vi "数据编码.vi"(0 "table输入":string(combo), 1 "仪器参数上传时间":enum16{"精确到小时", "原始时间"}(ring), 5 "错误常量 2":errorcluster caption="错误输入", 7 "仪器参数":string[](array[string]), 9 "QN":string, 11 "参数":string, 13 "MN":string, 14 "PW":string) -> (4 "错误常量":errorcluster caption="错误输出", 15 "通讯包字符串":string)   [LabVIEW 2016, in "数据传输系统-02.lvlib"]
panel:
  out "核查数据发送次数":i32
  out "小时数据发送次数":i32
  out "长度":i32
  in  "数据块":T1
  out "通讯包":T2={"包头（2）"="##", "数据段长度（4）"="", "数据段"="", "CRC校验"="", "包尾"=""}
  # "范例代码：\n\n##0101QN=20160801085857223;ST=32;CN=1062;PW=100000;MN=010000A8900016F000169DC0;Flag=5\n;CP=&&RtdInterval=30&&1C80\\r\\n"
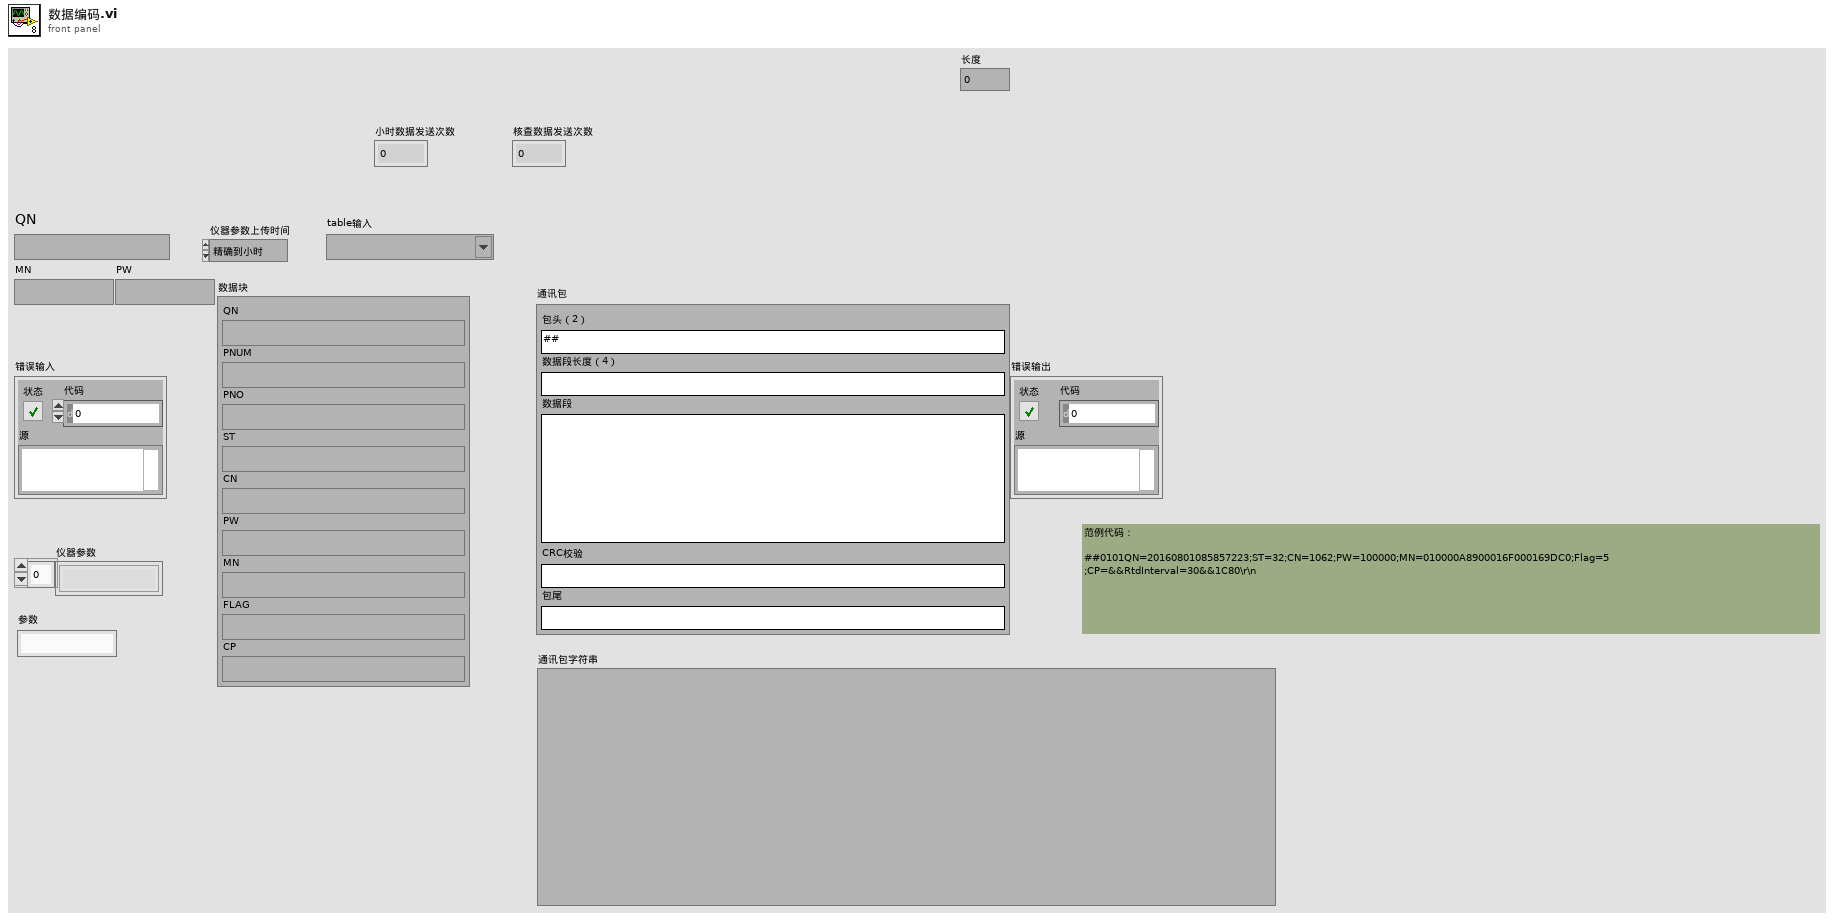
[diagram p1: front panel]
types:
  T1 = cluster{"QN":string, "ST":string, "CN":string, "PW":string, "MN":string, "FLAG":string, "PNUM":string, "PNO":string, "CP":string}
  T2 = cluster{"包头（2）":string, "数据段长度（4）":string, "数据段":string, "CRC校验":string, "包尾":string}
  T3 = cluster{"PH":string[][], "CODCr":string[][], "氨氮":string[][], "CODMn":string[][], "总氮":string[][], "总磷":string[][], "电导率":string[][], "水温":string[][], "COD":string[][], "DO":string[][], "浊度":string[][], "叶绿素":string[][], "藻密度":string[][], "铜":string[][], "盐度":string[][], "水位":string[][], "流速":string[][], "方向":string[][], "瞬时流量":string[][], "累积流量":string[][], "正累积流量":string[][], "负累积流量":string[][], "亚硝酸盐":string[][], "硫化物":string[][], "ORP":string[][], "铅":string[][], "镉":string[][], "锌":string[][], "镍":string[][], "锰":string[][], "汞":string[][], "气温":string[][], "气压":string[][], "风速":string[][], "风向":string[][], "空气温度":string[][], "相对湿度":string[][], "分钟雨量":string[][], "小时雨量":string[][], "日雨量":string[][], "累积雨量":string[][], "盐度":string[][], "磷酸盐":string[][], "硝氮":string[][], "氟化物":string[][], "挥发酚":string[][], "氯化物":string[][], "蓝绿藻":string[][], "余氯":string[][], "综合生物毒性":string[][], "水深":string[][]}
  T4 = enum16{"小时数据", "实时数据", "平行样测试", "集成干预测试", "加标回收测试", "核查数据", "空白零点跨度数据", "提取小时数据", "提取实时数据"}
  T5 = enum16{"小时数据", "实时数据", "平行样测试", "集成干预测试", "加标回收测试", "核查数据", "空白零点跨度数据", "提取小时数据", "提取实时数据", "操作日志"}
  T6 = enum16{"小时数据", "实时数据", "平行样测试", "集成干预测试", "加标回收测试", "核查数据", "空白零点跨度数据", "提取小时数据", "提取实时数据", "操作日志", "仪器参数", "3090仪器参数", "提取仪器参数", "报警信息"}
  T7 = cluster{"CODMn固件信息":string, "氨氮固件信息":string, "总磷固件信息":string, "总氮固件信息":string, "CODCr固件信息":string}
  T8 = typedef "数据传输系统-02.lvlib/应用环境.ctl" = enum16{"STD", "GB212", "婉仪平台"}
  T9 = cluster{"CODMn":dbl, "CODCr":dbl, "DO":dbl, "铜":dbl, "PH":dbl, "氨氮":dbl, "比电导率":dbl, "水温":dbl, "COD":dbl, "浊度":dbl, "总氮":dbl, "总磷":dbl, "叶绿素a":dbl, "藻密度":dbl, "水位":dbl, "流速":dbl, "方向":dbl, "瞬时流量":dbl, "累积流量":dbl, "正累积流量":dbl, "负累积流量":dbl, "亚硝酸盐":dbl, "硫化物":dbl, "ORP":dbl, "铅":dbl, "镉":dbl, "锌":dbl, "镍":dbl, "锰":dbl, "汞":dbl, "气温":dbl, "气压":dbl, "风速":dbl, "风向":dbl, "空气温度":dbl, "相对湿度":dbl, "分钟雨量":dbl, "小时雨量":dbl, "日雨量":dbl, "累积雨量":dbl, "盐度":dbl, "磷酸盐":dbl, "硝氮":dbl, "氟化物":dbl, "挥发酚":dbl, "氯化物":dbl, "蓝绿藻":dbl, "余氯":dbl, "综合生物毒性":dbl, "艏向":dbl, "横摇":dbl, "纵摇":dbl, "分层标志":dbl, "层状态1":dbl, "层状态2":dbl, "水平平均流速":dbl, "流向":dbl, "北向流速分量":dbl, "东向流速分量":dbl, "垂直流速分量":dbl, "最大波高":dbl, "最大波周期":dbl, "1/10波高":dbl, "1/10波周期":dbl, "有效波高":dbl, "有效波周期":dbl, "平均波高":dbl, "平均波周期":dbl, "波向":dbl, "波个数":dbl, "水深":dbl, "X轴流速":dbl, "Y轴流速":dbl, "信号强度":dbl, "电压":dbl, "悬浮物":dbl}
  T10 = cluster{"CODMn":string, "CODCr":string, "DO":string, "铜":string, "PH":string, "氨氮":string, "比电导率":string, "水温":string, "COD":string, "浊度":string, "总氮":string, "总磷":string, "叶绿素a":string, "藻密度":string, "水位":string, "流速":string, "方向":string, "瞬时流量":string, "累积流量":string, "正累积流量":string, "负累积流量":string, "亚硝酸盐":string, "硫化物":string, "ORP":string, "铅":string, "镉":string, "锌":string, "镍":string, "锰":string, "汞":string, "气温":string, "气压":string, "风速":string, "风向":string, "空气温度":string, "相对湿度":string, "分钟雨量":string, "小时雨量":string, "日雨量":string, "累积雨量":string, "盐度":string, "磷酸盐":string, "硝氮":string, "氟化物":string, "挥发酚":string, "氯化物":string, "蓝绿藻":string, "余氯":string, "综合生物毒性":string, "艏向":string, "横摇":string, "纵摇":string, "分层标志":string, "层状态1":string, "层状态2":string, "水平平均流速":string, "流向":string, "北向流速分量":string, "东向流速分量":string, "垂直流速分量":string, "最大波高":string, "最大波周期":string, "1/10波高":string, "1/10波周期":string, "有效波高":string, "有效波周期":string, "平均波高":string, "平均波周期":string, "波向":string, "波个数":string, "水深":string, "X轴流速":string, "Y轴流速":string, "信号强度":string, "电压":string, "悬浮物":string}
  T11 = typedef "LVDateTimeRec.ctl" = cluster{"秒数的小数部分":dbl, "秒":i32, "分":i32, "时":i32, "日":i32, "月":i32, "年":i32, "天数（周）":i32, "天数（年）":i32, "DST":i32}
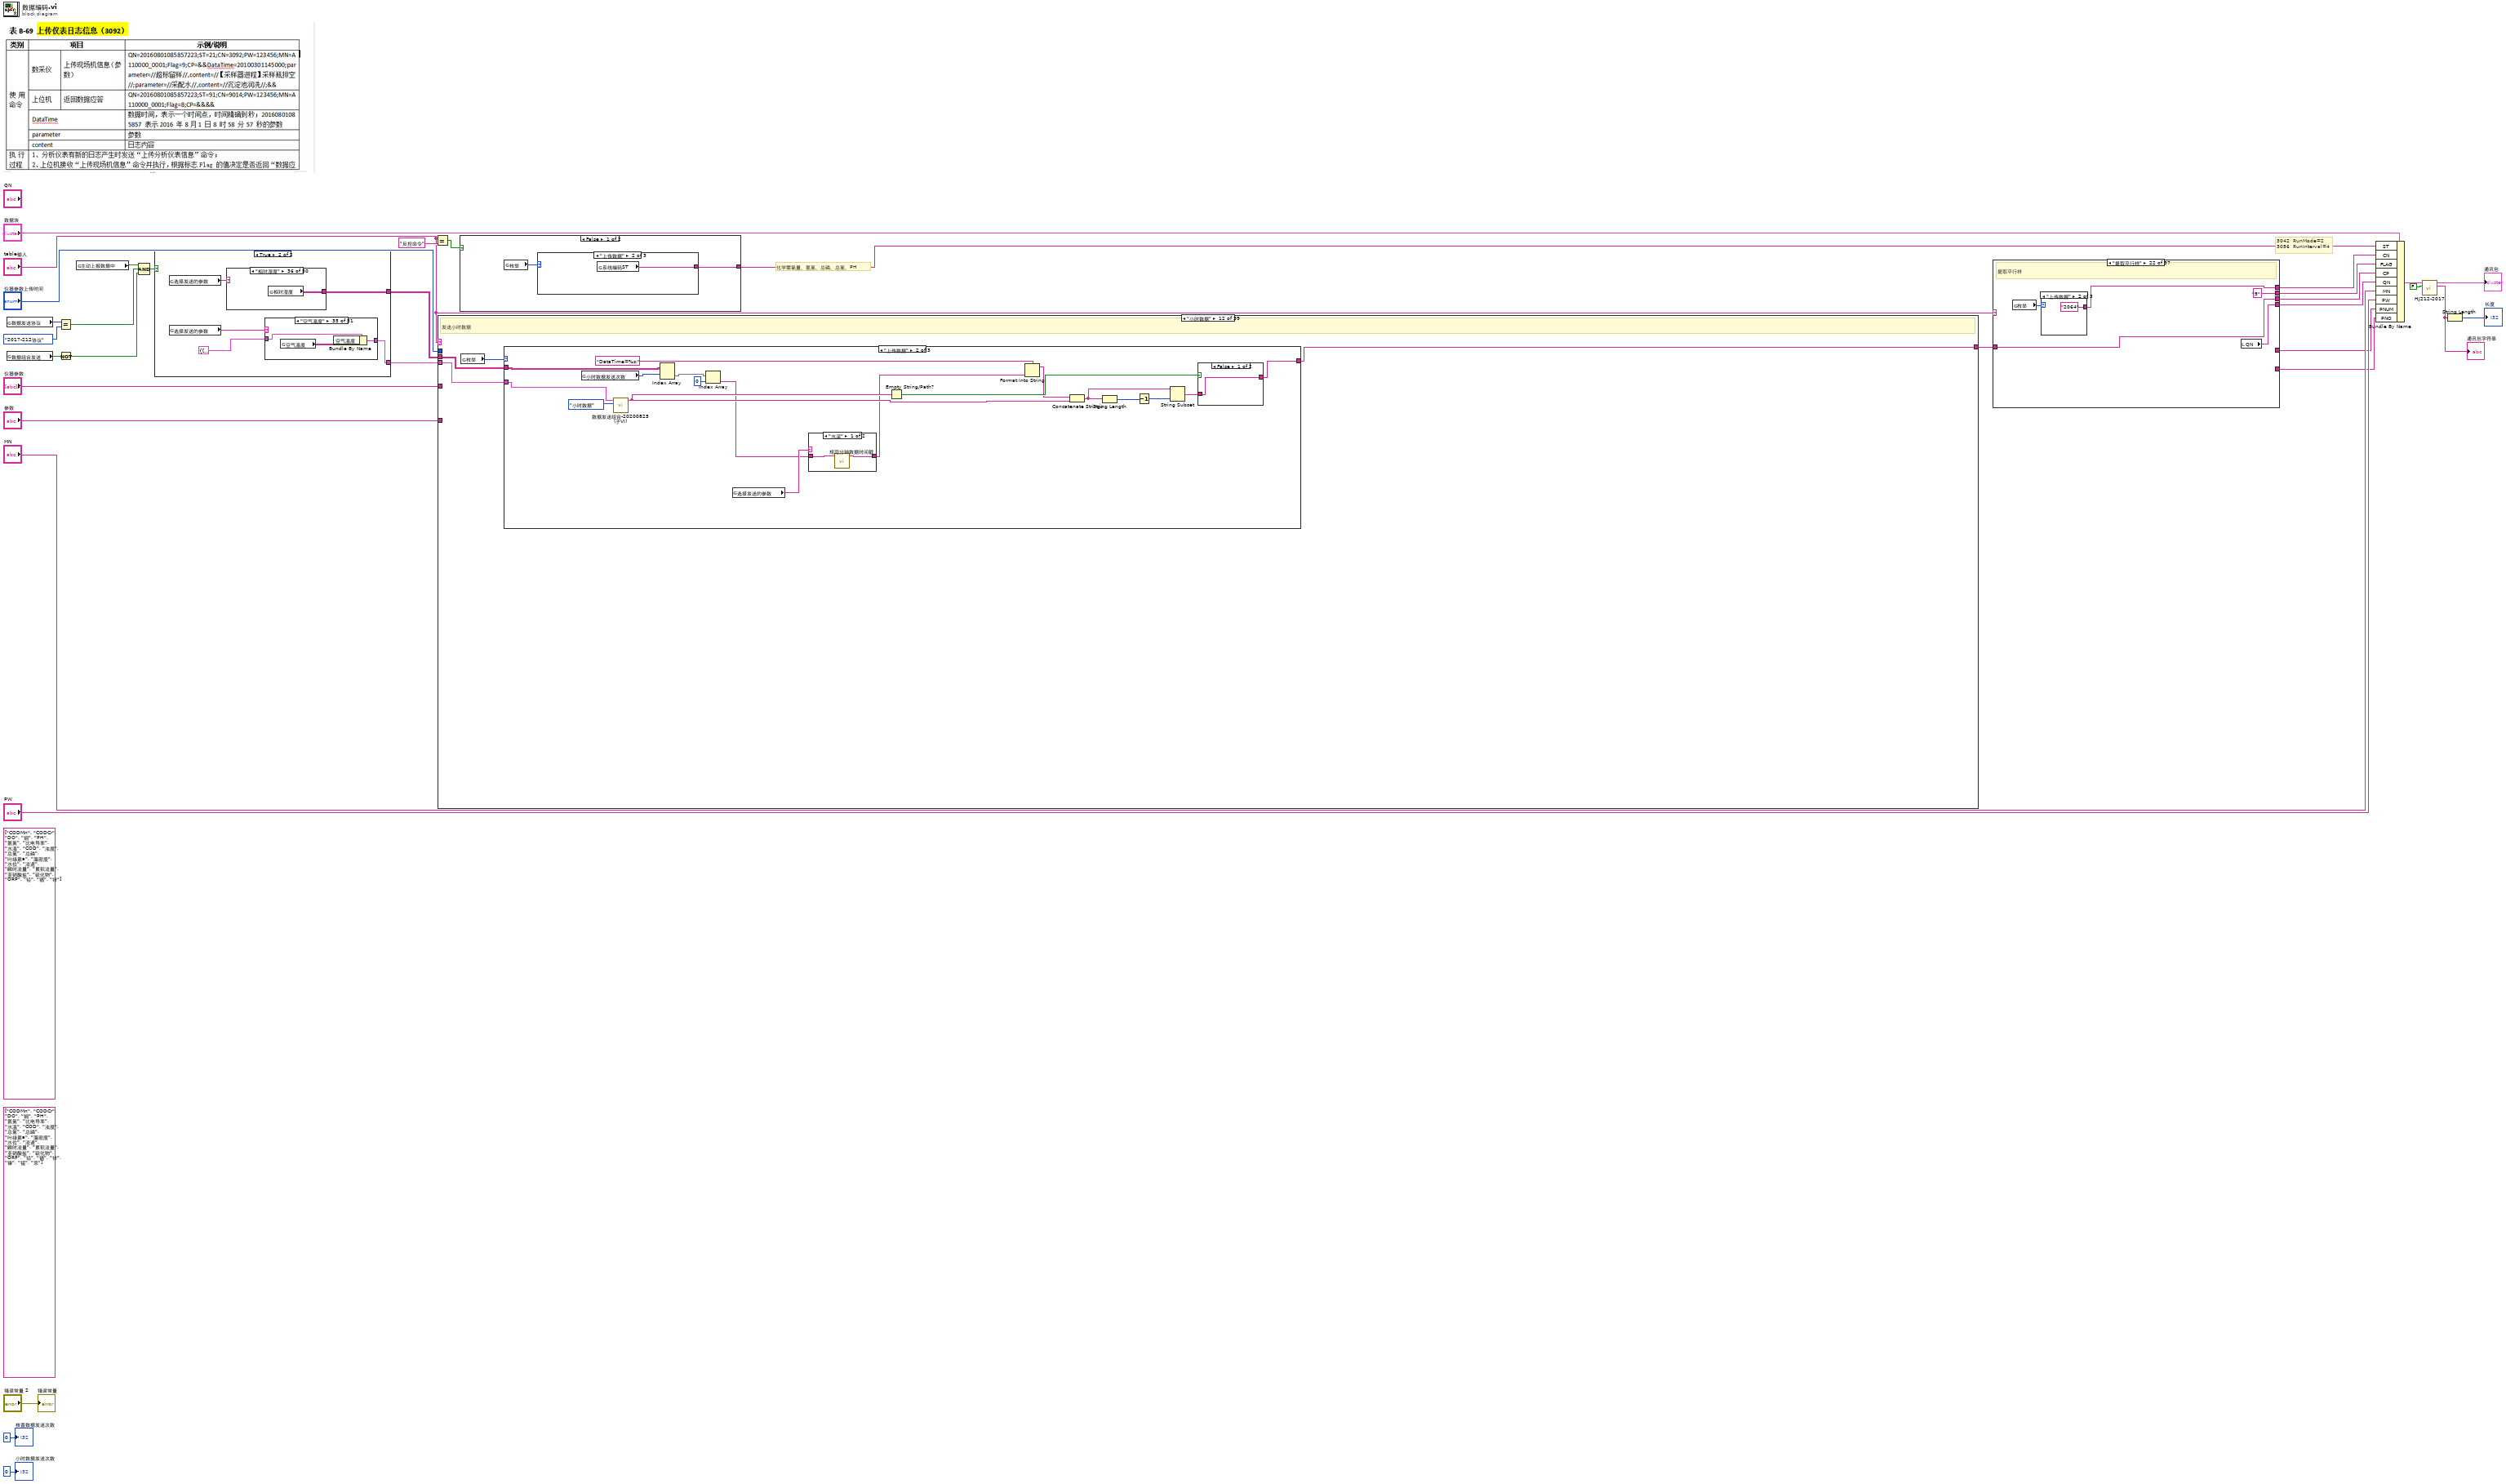
[diagram p0: block diagram]
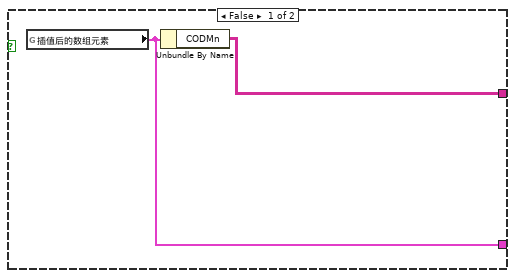
[diagram p2: hidden frame]
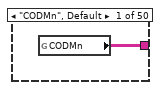
[diagram p3: hidden frame]
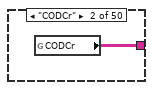
[diagram p4: hidden frame]
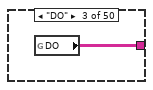
[diagram p5: hidden frame]
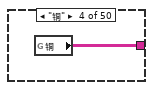
[diagram p6: hidden frame]
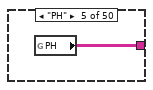
[diagram p7: hidden frame]
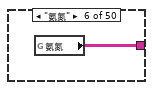
[diagram p8: hidden frame]
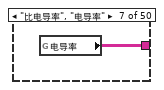
[diagram p9: hidden frame]
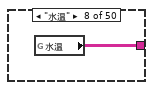
[diagram p10: hidden frame]
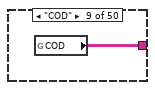
[diagram p11: hidden frame]
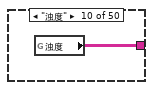
[diagram p12: hidden frame]
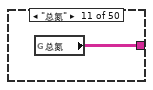
[diagram p13: hidden frame]
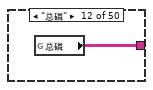
[diagram p14: hidden frame]
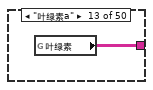
[diagram p15: hidden frame]
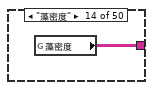
[diagram p16: hidden frame]
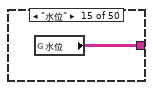
[diagram p17: hidden frame]
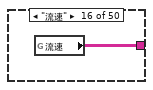
[diagram p18: hidden frame]
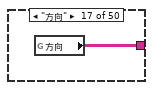
[diagram p19: hidden frame]
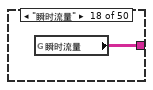
[diagram p20: hidden frame]
diagram:
  (unwired) string[] ["CODMn", "CODCr", "DO", "铜", "PH", "氨氮", "比电导率", "水温", "COD", "浊度", "总氮", "总磷", "叶绿素a", "藻密度", "水位", "流速", "瞬时流量", "累积流量", "亚硝酸盐", "硫化物", "ORP", "铅", "镉", "锌"] ("数组")
  (unwired) string[] ["CODMn", "CODCr", "DO", "铜", "PH", "氨氮", "比电导率", "水温", "COD", "浊度", "总氮", "总磷", "叶绿素a", "藻密度", "水位", "流速", "瞬时流量", "累积流量", "亚硝酸盐", "硫化物", "ORP", "铅", "镉", "锌", "镍", "锰", "汞"] ("数组")
  # "化学需氧量、氨氮、总磷、总氮、PH"
  # "3042  RunMode=2\n3056  RunInterval=4"
  n1 = global read "断电保存全局.vi" "数据发送协议"() -> (w13:enum16{"2005-212协议", "2017-212协议"})
  n2 = global read "断电保存全局.vi" "数据组合发送"() -> (w15:bool)
  n3 = Equal?(x=w13, y=enum16{"2005-212协议", "2017-212协议"}."2017-212协议" ("数据发送版本")) -> (x = y?=w16:bool)
  n4 = Not(x=w15) -> (.not. x?=w14:bool)
  n5 = global read "全局 数据发送重叠.vi" "主动上报数据中"() -> (w19:bool)
  n6 = Compound Arithmetic op=AND ("复合运算")(w19, w16, w14) -> (w17:bool)
  n7 = case shown="True" w17 {
    tunnel: [w36 w40] -> w11
    tunnel: [w35 w38] -> w10
    frame False {
      n8 = global read "插值后的新数组.vi" "插值后的数组元素"() -> (w36:T3)
      n9 = Unbundle By Name(w36) -> ("CODMn"=w35:string[][])
    }
    frame True {
      n10 = global read "全局 水样时间.vi" "选择发送的参数"() -> (w39:string)
      n11 = global read "全局 水样时间.vi" "选择发送的参数"() -> (w41:string)
      n12 = case shown="\"相对湿度\"" w39 {
        tunnel: [w42 w43 w44 w45 w46 w47 w48 w49 w50 w51 w52 w53 w54 w55 w56 w57 w58 w59 w60 w61 w62 w63 w64 w65 w66 w67 w68 w69 w70 w71 w72 w73 w74 w75 w76 w77 w78 w79 w80 w81 w82 w83 w84 w85 w86 w87 w88 w89 w90 w91] -> w38
        frame "CODMn", Default {
          n13 = global read "全局 所有参数.vi" "CODMn"() -> (w42:string[][])
        }
        frame "CODCr" {
          n14 = global read "全局 所有参数.vi" "CODCr"() -> (w43:string[][])
        }
        frame "DO" {
          n15 = global read "全局 所有参数.vi" "DO"() -> (w44:string[][])
        }
        frame "铜" {
          n16 = global read "全局 所有参数.vi" "铜"() -> (w45:string[][])
        }
        frame "PH" {
          n17 = global read "全局 所有参数.vi" "PH"() -> (w46:string[][])
        }
        frame "氨氮" {
          n18 = global read "全局 所有参数.vi" "氨氮"() -> (w47:string[][])
        }
        frame "比电导率", "电导率" {
          n19 = global read "全局 所有参数.vi" "电导率"() -> (w48:string[][])
        }
        frame "水温" {
          n20 = global read "全局 所有参数.vi" "水温"() -> (w49:string[][])
        }
        frame "COD" {
          n21 = global read "全局 所有参数.vi" "COD"() -> (w50:string[][])
        }
        frame "浊度" {
          n22 = global read "全局 所有参数.vi" "浊度"() -> (w51:string[][])
        }
        frame "总氮" {
          n23 = global read "全局 所有参数.vi" "总氮"() -> (w52:string[][])
        }
        frame "总磷" {
          n24 = global read "全局 所有参数.vi" "总磷"() -> (w53:string[][])
        }
        frame "叶绿素a" {
          n25 = global read "全局 所有参数.vi" "叶绿素"() -> (w54:string[][])
        }
        frame "藻密度" {
          n26 = global read "全局 所有参数.vi" "藻密度"() -> (w55:string[][])
        }
        frame "水位" {
          n27 = global read "全局 所有参数.vi" "水位"() -> (w56:string[][])
        }
        frame "流速" {
          n28 = global read "全局 所有参数.vi" "流速"() -> (w57:string[][])
        }
        frame "方向" {
          n29 = global read "全局 所有参数.vi" "方向"() -> (w58:string[][])
        }
        frame "瞬时流量" {
          n30 = global read "全局 所有参数.vi" "瞬时流量"() -> (w59:string[][])
        }
        frame "累积流量" {
          n31 = global read "全局 所有参数.vi" "累积流量"() -> (w60:string[][])
        }
        frame "正累积流量" {
          n32 = global read "全局 所有参数.vi" "正累积流量"() -> (w61:string[][])
        }
        frame "负累积流量" {
          n33 = global read "全局 所有参数.vi" "负累积流量"() -> (w62:string[][])
        }
        frame "亚硝氮" {
          n34 = global read "全局 所有参数.vi" "亚硝酸盐"() -> (w63:string[][])
        }
        frame "硫化物" {
          n35 = global read "全局 所有参数.vi" "硫化物"() -> (w64:string[][])
        }
        frame "ORP" {
          n36 = global read "全局 所有参数.vi" "ORP"() -> (w65:string[][])
        }
        frame "铅" {
          n37 = global read "全局 所有参数.vi" "铅"() -> (w66:string[][])
        }
        frame "镉" {
          n38 = global read "全局 所有参数.vi" "镉"() -> (w67:string[][])
        }
        frame "锌" {
          n39 = global read "全局 所有参数.vi" "锌"() -> (w68:string[][])
        }
        frame "镍" {
          n40 = global read "全局 所有参数.vi" "镍"() -> (w69:string[][])
        }
        frame "锰" {
          n41 = global read "全局 所有参数.vi" "锰"() -> (w70:string[][])
        }
        frame "汞" {
          n42 = global read "全局 所有参数.vi" "汞"() -> (w71:string[][])
        }
        frame "气温" {
          n43 = global read "全局 所有参数.vi" "气温"() -> (w72:string[][])
        }
        frame "气压" {
          n44 = global read "全局 所有参数.vi" "气压"() -> (w73:string[][])
        }
        frame "风速" {
          n45 = global read "全局 所有参数.vi" "风速"() -> (w74:string[][])
        }
        frame "风向" {
          n46 = global read "全局 所有参数.vi" "风向"() -> (w75:string[][])
        }
        frame "空气温度" {
          n47 = global read "全局 所有参数.vi" "空气温度"() -> (w76:string[][])
        }
        frame "相对湿度" {
          n48 = global read "全局 所有参数.vi" "相对湿度"() -> (w77:string[][])
        }
        frame "分钟雨量" {
          n49 = global read "全局 所有参数.vi" "分钟雨量"() -> (w78:string[][])
        }
        frame "小时雨量" {
          n50 = global read "全局 所有参数.vi" "小时雨量"() -> (w79:string[][])
        }
        frame "日雨量" {
          n51 = global read "全局 所有参数.vi" "日雨量"() -> (w80:string[][])
        }
        frame "累积雨量" {
          n52 = global read "全局 所有参数.vi" "累积雨量"() -> (w81:string[][])
        }
        frame "盐度" {
          n53 = global read "全局 所有参数.vi" "盐度"() -> (w82:string[][])
        }
        frame "磷酸盐" {
          n54 = global read "全局 所有参数.vi" "磷酸盐"() -> (w83:string[][])
        }
        frame "硝氮" {
          n55 = global read "全局 所有参数.vi" "硝氮"() -> (w84:string[][])
        }
        frame "氟化物" {
          n56 = global read "全局 所有参数.vi" "氟化物"() -> (w85:string[][])
        }
        frame "挥发酚" {
          n57 = global read "全局 所有参数.vi" "挥发酚"() -> (w86:string[][])
        }
        frame "氯化物" {
          n58 = global read "全局 所有参数.vi" "氯化物"() -> (w87:string[][])
        }
        frame "蓝绿藻" {
          n59 = global read "全局 所有参数.vi" "蓝绿藻"() -> (w88:string[][])
        }
        frame "余氯" {
          n60 = global read "全局 所有参数.vi" "余氯"() -> (w89:string[][])
        }
        frame "综合生物毒性" {
          n61 = global read "全局 所有参数.vi" "综合生物毒性"() -> (w90:string[][])
        }
        frame "水深" {
          n62 = global read "全局 所有参数.vi" "水深"() -> (w91:string[][])
        }
      }
      n63 = case shown="\"空气温度\"" w41 {
        tunnel: T3 {"PH"=[], "CODCr"=[], "氨氮"=[], "CODMn"=[], "总氮"=[], "总磷"=[], "电导率"=[], "水温"=[], "COD"=[], "DO"=[], "浊度"=[], "叶绿素"=[], "藻密度"=[], "铜"=[], "盐度"=[], "水位"=[], "流速"=[], "方向"=[], "瞬时流量"=[], "累积流量"=[], "正累积流量"=[], "负累积流量"=[], "亚硝酸盐"=[], "硫化物"=[], "ORP"=[], "铅"=[], "镉"=[], "锌"=[], "镍"=[], "锰"=[], "汞"=[], "气温"=[], "气压"=[], "风速"=[], "风向"=[], "空气温度"=[], "相对湿度"=[], "分钟雨量"=[], "小时雨量"=[], "日雨量"=[], "累积雨量"=[], "盐度"=[], "磷酸盐"=[], "硝氮"=[], "氟化物"=[], "挥发酚"=[], "氯化物"=[], "蓝绿藻"=[], "余氯"=[], "综合生物毒性"=[], "水深"=[]} ("插值后的数组元素") -> [w92 w94 w98 w101 w104 w107 w110 w113 w116 w119 w122 w125 w128 w130 w134 w137 w140 w142 w145 w148 w151 w154 w157 w160 w163 w166 w169 w172 w175 w178 w181 w184 w187 w190 w193 w196 w199 w202 w205 w208 w211 w214 w217 w220 w223 w226 w229 w232 w235 w238 w241]
        tunnel: [w92 w93 w96 w99 w102 w105 w108 w112 w115 w117 w120 w123 w126 w129 w132 w135 w138 w141 w144 w147 w150 w153 w156 w159 w162 w165 w168 w171 w174 w177 w180 w183 w186 w189 w192 w195 w198 w201 w204 w207 w210 w213 w216 w219 w222 w225 w228 w231 w234 w237 w240] -> w40
        frame Default {
        }
        frame "CODMn" {
          n64 = global read "全局 所有参数.vi" "CODMn"() -> (w95:string[][])
          n65 = Bundle By Name(cluster=w94, "CODMn"=w95) -> (w93:T3)
        }
        frame "CODCr" {
          n66 = global read "全局 所有参数.vi" "CODCr"() -> (w97:string[][])
          n67 = Bundle By Name(cluster=w98, "CODCr"=w97) -> (w96:T3)
        }
        frame "DO" {
          n68 = global read "全局 所有参数.vi" "DO"() -> (w100:string[][])
          n69 = Bundle By Name(cluster=w101, "DO"=w100) -> (w99:T3)
        }
        frame "铜" {
          n70 = global read "全局 所有参数.vi" "铜"() -> (w103:string[][])
          n71 = Bundle By Name(cluster=w104, "铜"=w103) -> (w102:T3)
        }
        frame "PH" {
          n72 = global read "全局 所有参数.vi" "PH"() -> (w106:string[][])
          n73 = Bundle By Name(cluster=w107, "PH"=w106) -> (w105:T3)
        }
        frame "氨氮" {
          n74 = global read "全局 所有参数.vi" "氨氮"() -> (w109:string[][])
          n75 = Bundle By Name(cluster=w110, "氨氮"=w109) -> (w108:T3)
        }
        frame "比电导率", "电导率" {
          n76 = global read "全局 所有参数.vi" "电导率"() -> (w111:string[][])
          n77 = Bundle By Name(cluster=w113, "电导率"=w111) -> (w112:T3)
        }
        frame "水温" {
          n78 = global read "全局 所有参数.vi" "水温"() -> (w114:string[][])
          n79 = Bundle By Name(cluster=w116, "水温"=w114) -> (w115:T3)
        }
        frame "浊度" {
          n80 = global read "全局 所有参数.vi" "浊度"() -> (w118:string[][])
          n81 = Bundle By Name(cluster=w119, "浊度"=w118) -> (w117:T3)
        }
        frame "总氮" {
          n82 = global read "全局 所有参数.vi" "总氮"() -> (w121:string[][])
          n83 = Bundle By Name(cluster=w122, "总氮"=w121) -> (w120:T3)
        }
        frame "总磷" {
          n84 = global read "全局 所有参数.vi" "总磷"() -> (w124:string[][])
          n85 = Bundle By Name(cluster=w125, "总磷"=w124) -> (w123:T3)
        }
        frame "叶绿素a" {
          n86 = global read "全局 所有参数.vi" "叶绿素"() -> (w127:string[][])
          n87 = Bundle By Name(cluster=w128, "叶绿素"=w127) -> (w126:T3)
        }
        frame "藻密度" {
          n88 = global read "全局 所有参数.vi" "藻密度"() -> (w131:string[][])
          n89 = Bundle By Name(cluster=w130, "藻密度"=w131) -> (w129:T3)
        }
        frame "水位" {
          n90 = global read "全局 所有参数.vi" "水位"() -> (w133:string[][])
          n91 = Bundle By Name(cluster=w134, "水位"=w133) -> (w132:T3)
        }
        frame "流速" {
          n92 = global read "全局 所有参数.vi" "流速"() -> (w136:string[][])
          n93 = Bundle By Name(cluster=w137, "流速"=w136) -> (w135:T3)
        }
        frame "方向" {
          n94 = global read "全局 所有参数.vi" "方向"() -> (w139:string[][])
          n95 = Bundle By Name(cluster=w140, "方向"=w139) -> (w138:T3)
        }
        frame "瞬时流量" {
          n96 = global read "全局 所有参数.vi" "瞬时流量"() -> (w143:string[][])
          n97 = Bundle By Name(cluster=w142, "瞬时流量"=w143) -> (w141:T3)
        }
        frame "累积流量" {
          n98 = global read "全局 所有参数.vi" "累积流量"() -> (w146:string[][])
          n99 = Bundle By Name(cluster=w145, "累积流量"=w146) -> (w144:T3)
        }
        frame "正累积流量" {
          n100 = global read "全局 所有参数.vi" "正累积流量"() -> (w149:string[][])
          n101 = Bundle By Name(cluster=w148, "正累积流量"=w149) -> (w147:T3)
        }
        frame "负累积流量" {
          n102 = global read "全局 所有参数.vi" "负累积流量"() -> (w152:string[][])
          n103 = Bundle By Name(cluster=w151, "负累积流量"=w152) -> (w150:T3)
        }
        frame "亚硝氮" {
          n104 = global read "全局 所有参数.vi" "亚硝酸盐"() -> (w155:string[][])
          n105 = Bundle By Name(cluster=w154, "亚硝酸盐"=w155) -> (w153:T3)
        }
        frame "硫化物" {
          n106 = global read "全局 所有参数.vi" "硫化物"() -> (w158:string[][])
          n107 = Bundle By Name(cluster=w157, "硫化物"=w158) -> (w156:T3)
        }
        frame "ORP" {
          n108 = global read "全局 所有参数.vi" "ORP"() -> (w161:string[][])
          n109 = Bundle By Name(cluster=w160, "ORP"=w161) -> (w159:T3)
        }
        frame "铅" {
          n110 = global read "全局 所有参数.vi" "铅"() -> (w164:string[][])
          n111 = Bundle By Name(cluster=w163, "铅"=w164) -> (w162:T3)
        }
        frame "镉" {
          n112 = global read "全局 所有参数.vi" "镉"() -> (w167:string[][])
          n113 = Bundle By Name(cluster=w166, "镉"=w167) -> (w165:T3)
        }
        frame "锌" {
          n114 = global read "全局 所有参数.vi" "锌"() -> (w170:string[][])
          n115 = Bundle By Name(cluster=w169, "锌"=w170) -> (w168:T3)
        }
        frame "镍" {
          n116 = global read "全局 所有参数.vi" "镍"() -> (w173:string[][])
          n117 = Bundle By Name(cluster=w172, "镍"=w173) -> (w171:T3)
        }
        frame "锰" {
          n118 = global read "全局 所有参数.vi" "锰"() -> (w176:string[][])
          n119 = Bundle By Name(cluster=w175, "锰"=w176) -> (w174:T3)
        }
        frame "汞" {
          n120 = global read "全局 所有参数.vi" "汞"() -> (w179:string[][])
          n121 = Bundle By Name(cluster=w178, "汞"=w179) -> (w177:T3)
        }
        frame "气温" {
          n122 = global read "全局 所有参数.vi" "气温"() -> (w182:string[][])
          n123 = Bundle By Name(cluster=w181, "气温"=w182) -> (w180:T3)
        }
        frame "气压" {
          n124 = global read "全局 所有参数.vi" "气压"() -> (w185:string[][])
          n125 = Bundle By Name(cluster=w184, "气压"=w185) -> (w183:T3)
        }
        frame "风速" {
          n126 = global read "全局 所有参数.vi" "风速"() -> (w188:string[][])
          n127 = Bundle By Name(cluster=w187, "风速"=w188) -> (w186:T3)
        }
        frame "风向" {
          n128 = global read "全局 所有参数.vi" "风向"() -> (w191:string[][])
          n129 = Bundle By Name(cluster=w190, "风向"=w191) -> (w189:T3)
        }
        frame "空气温度" {
          n130 = global read "全局 所有参数.vi" "空气温度"() -> (w194:string[][])
          n131 = Bundle By Name(cluster=w193, "空气温度"=w194) -> (w192:T3)
        }
        frame "相对湿度" {
          n132 = global read "全局 所有参数.vi" "相对湿度"() -> (w197:string[][])
          n133 = Bundle By Name(cluster=w196, "相对湿度"=w197) -> (w195:T3)
        }
        frame "分钟雨量" {
          n134 = global read "全局 所有参数.vi" "分钟雨量"() -> (w200:string[][])
          n135 = Bundle By Name(cluster=w199, "分钟雨量"=w200) -> (w198:T3)
        }
        frame "小时雨量" {
          n136 = global read "全局 所有参数.vi" "小时雨量"() -> (w203:string[][])
          n137 = Bundle By Name(cluster=w202, "小时雨量"=w203) -> (w201:T3)
        }
        frame "日雨量" {
          n138 = global read "全局 所有参数.vi" "日雨量"() -> (w206:string[][])
          n139 = Bundle By Name(cluster=w205, "日雨量"=w206) -> (w204:T3)
        }
        frame "累积雨量" {
          n140 = global read "全局 所有参数.vi" "累积雨量"() -> (w209:string[][])
          n141 = Bundle By Name(cluster=w208, "累积雨量"=w209) -> (w207:T3)
        }
        frame "盐度" {
          n142 = global read "全局 所有参数.vi" "盐度"() -> (w212:string[][])
          n143 = Bundle By Name(cluster=w211, "盐度"=w212) -> (w210:T3)
        }
        frame "COD" {
          n144 = global read "全局 所有参数.vi" "COD"() -> (w215:string[][])
          n145 = Bundle By Name(cluster=w214, "COD"=w215) -> (w213:T3)
        }
        frame "磷酸盐" {
          n146 = global read "全局 所有参数.vi" "磷酸盐"() -> (w218:string[][])
          n147 = Bundle By Name(cluster=w217, "磷酸盐"=w218) -> (w216:T3)
        }
        frame "硝氮" {
          n148 = global read "全局 所有参数.vi" "硝氮"() -> (w221:string[][])
          n149 = Bundle By Name(cluster=w220, "硝氮"=w221) -> (w219:T3)
        }
        frame "氟化物" {
          n150 = global read "全局 所有参数.vi" "氟化物"() -> (w224:string[][])
          n151 = Bundle By Name(cluster=w223, "氟化物"=w224) -> (w222:T3)
        }
        frame "挥发酚" {
          n152 = global read "全局 所有参数.vi" "挥发酚"() -> (w227:string[][])
          n153 = Bundle By Name(cluster=w226, "挥发酚"=w227) -> (w225:T3)
        }
        frame "氯化物" {
          n154 = global read "全局 所有参数.vi" "氯化物"() -> (w230:string[][])
          n155 = Bundle By Name(cluster=w229, "氯化物"=w230) -> (w228:T3)
        }
        frame "蓝绿藻" {
          n156 = global read "全局 所有参数.vi" "蓝绿藻"() -> (w233:string[][])
          n157 = Bundle By Name(cluster=w232, "蓝绿藻"=w233) -> (w231:T3)
        }
        frame "余氯" {
          n158 = global read "全局 所有参数.vi" "余氯"() -> (w236:string[][])
          n159 = Bundle By Name(cluster=w235, "余氯"=w236) -> (w234:T3)
        }
        frame "综合生物毒性" {
          n160 = global read "全局 所有参数.vi" "综合生物毒性"() -> (w239:string[][])
          n161 = Bundle By Name(cluster=w238, "综合生物毒性"=w239) -> (w237:T3)
        }
        frame "水深" {
          n162 = global read "全局 所有参数.vi" "水深"() -> (w242:string[][])
          n163 = Bundle By Name(cluster=w241, "水深"=w242) -> (w240:T3)
        }
      }
    }
  }
  n164 = Equal?(x="table输入", y="反控命令") -> (x = y?=w25:bool)
  n165 = case shown="\"小时数据\"" "table输入" {
    tunnel: [w244 w251 w265 w307 w345 _ w359 w368 w375 w385 w396 w551 w587 w638 w666 w684 w732 w784 w818 w850 w881 w907 w936 w966 w1002 w1035 w1068 w1107 w1272 w1314 w1479 w1507 w1530 w1566 w1589 w1600 w1608 w1618 w1628] -> w20
    tunnel: w10 -> [_ _ _ _ _ _ _ _ _ _ w393 w550 _ _ _ _ _ w783 w819 w845 w876 w908 w935 w965 w1001 _ _ _ _ _ w1478 _ w1529 _ _ _ _ _ _]
    tunnel: w11 -> [_ _ _ _ _ _ _ _ _ _ w394 w552 _ _ _ _ _ w779 w814 w846 w877 w906 w934 w964 w997 _ _ _ _ _ w1474 w1505 w1525 _ _ _ _ _ _]
    tunnel: "仪器参数" -> [_ _ _ _ _ _ _ _ _ _ _ _ _ _ _ _ _ _ _ _ _ _ _ _ _ _ _ w1103 w1270 w1310 _ _ _ _ _ _ _ _ _]
    tunnel: "参数" -> [_ _ _ _ _ _ _ _ _ _ _ _ _ _ _ _ _ _ _ _ _ _ _ _ _ _ _ w1105 _ w1312 _ _ _ _ _ _ _ _ _]
    tunnel: "仪器参数上传时间" -> [_ _ _ _ _ _ _ _ _ _ _ _ _ _ _ _ _ _ _ _ _ _ _ _ _ _ _ w1102 w1269 w1309 _ _ _ _ _ _ _ _ _]
    frame "反控命令" {
      n166 = global read "全局 反控命令枚举.vi" "反控命令枚举"() -> (w243:enum16{"返回请求应答", "返回执行结果"})
      n167 = case shown="\"返回执行结果\"" w243 {
        tunnel: ["QnRtn=1" w247] -> w244
        frame "返回请求应答", Default {
        }
        frame "返回执行结果" {
          n168 = global read "全局 反控命令枚举.vi" "执行结果定义"() -> (w248:u16)
          n169 = Number To Decimal String(number=w248) -> (decimal integer string=w246:string)  [unwired: 1 in]
          n170 = Concatenate Strings("ExeRtn=", w246) -> (w247:string)
        }
      }
    }
    frame "超标留样返回" {
      n171 = global read "全局1.vi" "枚举"() -> (w250:enum16{"返回请求应答", "上传数据", "返回执行结果"})
      n172 = case shown="\"上传数据\"" w250 {
        tunnel: ["QnRtn=1" w253 "ExeRtn=1"] -> w251
        frame "返回请求应答", Default {
        }
        frame "上传数据" {
          n173 = global read "全局1.vi" "register values"() -> (w262:u16[])
          n174 = Get Date/Time In Seconds() -> (seconds since 1Jan1904=w260:timestamp)
          n175 = Index Array(array=w262, index=7 ("索引")) -> (element=w255:u16)
          n176 = Format Date/Time String(time format string (%c)="%Y%m%d%H%M%S" ("时间格式字符串(%c)"), seconds (now)=w260) -> (date/time string=w258:string)  [unwired: 1 in]
          n177 = Number To Decimal String(number=w255) -> (decimal integer string=w256:string)  [unwired: 1 in]
          n178 = Format Into String(format string="VaseNo=%s" ("格式字符串"), w256) -> (resulting string=w254:string)  [unwired: 2 in, 1 out]
          n179 = Format Into String(format string="DataTime=%s;%s" ("格式字符串"), w258, w254) -> (resulting string=w253:string)  [unwired: 2 in, 1 out]
        }
        frame "返回执行结果" {
        }
      }
    }
    frame "提取经纬度环境信息" {
      # "BDS纬度"
      # "BDS纬度"
      # "GPS纬度"
      # "GPS经度"
      # "湿度"
      # "温度"
      # "电压"
      # "时间"
      n180 = global read "全局1.vi" "枚举"() -> (w266:enum16{"返回请求应答", "上传数据", "返回执行结果"})
      n181 = case shown="\"返回执行结果\"" w266 {
        tunnel: ["QnRtn=1" w279 "ExeRtn=1"] -> w265
        frame "返回请求应答", Default {
        }
        frame "上传数据" {
          n182 = global read "全局 环境参数.vi" "环境参数"() -> (w269:string[][])
          n183 = global read "全局 环境参数.vi" "columns输出"() -> (w276:string[])
          n184 = Index Array(array=w269, index (row)=0 ("索引 (行)")) -> (element=w272:string[])  [unwired: 1 in]
          n185 = Get Date/Time In Seconds() -> (seconds since 1Jan1904=w281:timestamp)
          n186 = Array Subset(array=w276, index=1 ("索引")) -> (w277:string[])  [unwired: 1 in]
          n187 = for {
            tunnel: w277 -> [w285] mode=indexing
            tunnel: [w284] -> w278 mode=indexing
            n188 = case shown="\"BDS经度\"" w285 {
              tunnel: ["" "Volt=%s;" "Temp=%s;" ("格式字符串") "Hum=%s;" ("格式字符串") "Lng=%s;" "Lat=%s;" "Lng2=%s;" "Lat2=%s;"] -> w284
              frame "假", Default {
              }
              frame "电压" {
              }
              frame "室温" {
              }
              frame "湿度" {
              }
              frame "GPS经度" {
              }
              frame "GPS纬度" {
              }
              frame "BDS经度" {
              }
              frame "BDS纬度" {
              }
            }
          }
          n189 = Format Date/Time String(time format string (%c)="%Y%m%d%H%M%S" ("时间格式字符串(%c)"), seconds (now)=w281) -> (date/time string=w280:string)  [unwired: 1 in]
          n190 = Array Subset(array=w272, index=1 ("索引")) -> (w274:string[])  [unwired: 1 in]
          n191 = for {
            shift-right: [w299] -> w268
            shift-left: "" -> [w298]
            tunnel: w278 -> [w297] mode=indexing
            tunnel: w274 -> [w295] mode=indexing
            n192 = Empty String/Path?(string/path=w295) -> (empty?=w301:bool)
            n193 = Fract/Exp String To Number(string=w295) -> (number=w296:dbl)  [unwired: 3 in, 1 out]
            n194 = Number To Fractional String(number=w296) -> (F-format string=w294:string)  [unwired: 3 in]
            n195 = case shown="False" w301 {
              tunnel: [w304 w305] -> w300
              tunnel: w297 -> [w303 _]
              tunnel: w294 -> [w302 _]
              tunnel: w294 -> [_ w305]
              frame False {
                n196 = Format Into String(format string=w303, w302) -> (resulting string=w304:string)  [unwired: 2 in, 1 out]
              }
              frame True {
              }
            }
            n197 = Concatenate Strings(w298, w300) -> (w299:string)
          }
          n198 = Format Into String(format string="DataTime=%s;%s" ("格式字符串"), w280, w268) -> (resulting string=w279:string)  [unwired: 2 in, 1 out]
        }
        frame "返回执行结果" {
        }
      }
    }
    frame "提取现场系统信息" {
      n199 = global read "全局1.vi" "枚举"() -> (w308:enum16{"返回请求应答", "上传数据", "返回执行结果"})
      n200 = case shown="\"返回执行结果\"" w308 {
        tunnel: ["QnRtn=1" w342 "ExeRtn=1"] -> w307
        frame "返回请求应答", Default {
        }
        frame "上传数据" {
          n201 = global read "全局1.vi" "register values"() -> (w341:u16[])
          n202 = global read "全局1.vi" "系统信息"() -> (w323:u16[])
          n203 = Get Date/Time In Seconds() -> (seconds since 1Jan1904=w328:timestamp)
          n204 = Format Date/Time String(time format string (%c)="%Y%m%d%H%M%S%u" ("时间格式字符串(%c)"), seconds (now)=w328) -> (date/time string=w331:string)  [unwired: 1 in]
          n205 = Number To Decimal String(number=w323) -> (decimal integer string=w322:string[])  [unwired: 1 in]
          n206 = Index Array(array=w341, index #1=0 ("索引"), index #2=6 ("索引")) -> (element #1=w337:u16, element #2=w325:u16)
          n207 = Number To Decimal String(number=w337) -> (decimal integer string=w339:string)  [unwired: 1 in]
          n208 = Number To Decimal String(number=w325) -> (decimal integer string=w334:string)  [unwired: 1 in]
          n209 = Index Array(array=w322) -> (element #1=w320:string, element #2=w317:string, element #3=w314:string, element #4=w311:string)  [unwired: 4 in]
          n210 = Search and Replace String(input string=w331, search string="." ("搜索字符串")) -> (result string=w327:string)  [unwired: 6 in, 3 out]
          n211 = Format Into String(format string="SystemTask=%s;" ("格式字符串"), w320) -> (resulting string=w319:string)  [unwired: 2 in, 1 out]
          n212 = Format Into String(format string="PumpState=%s;" ("格式字符串"), w317) -> (resulting string=w316:string)  [unwired: 2 in, 1 out]
          n213 = Format Into String(format string="AlgClean=%s;" ("格式字符串"), w314) -> (resulting string=w313:string)  [unwired: 2 in, 1 out]
          n214 = Format Into String(format string="SystemAlarm=0%s;" ("格式字符串"), w311) -> (resulting string=w310:string)  [unwired: 2 in, 1 out]
          n215 = Format Into String(format string="RunMode=%s;" ("格式字符串"), w339) -> (resulting string=w324:string)  [unwired: 2 in, 1 out]
          n216 = Format Into String(format string="RunInterval=%s;" ("格式字符串"), w334) -> (resulting string=w335:string)  [unwired: 2 in, 1 out]
          n217 = Format Into String(format string="SystemTime=%s;" ("格式字符串"), w327) -> (resulting string=w332:string)  [unwired: 2 in, 1 out]
          n218 = Concatenate Strings(w324, w316, w319, w313, w310, w335, w332) -> (w342:string)
        }
        frame "返回执行结果" {
        }
      }
    }
    frame "提取监测仪表时间" {
      n219 = global read "全局1.vi" "枚举"() -> (w344:enum16{"返回请求应答", "上传数据", "返回执行结果"})
      n220 = case shown="\"上传数据\"" w344 {
        tunnel: ["QnRtn=1" w357 "ExeRtn=1"] -> w345
        frame "返回请求应答", Default {
        }
        frame "上传数据" {
          n221 = global read "全局 提取仪器参数.vi" "仪器编码"() -> (w347:string)
          n222 = Format Into String(format string="PolId=%s;" ("格式字符串"), w347) -> (resulting string=w355:string)  [unwired: 2 in, 1 out]
          n223 = Get Date/Time In Seconds() -> (seconds since 1Jan1904=w350:timestamp)
          n224 = Format Date/Time String(time format string (%c)="%Y%m%d%H%M%S%u" ("时间格式字符串(%c)"), seconds (now)=w350) -> (date/time string=w353:string)  [unwired: 1 in]
          n225 = Search and Replace String(input string=w353, search string="." ("搜索字符串")) -> (result string=w349:string)  [unwired: 6 in, 3 out]
          n226 = Format Into String(format string="SystemTime=%s;" ("格式字符串"), w349) -> (resulting string=w348:string)  [unwired: 2 in, 1 out]
          n227 = Concatenate Strings(w355, w348) -> (w357:string)
        }
        frame "返回执行结果" {
        }
      }
    }
    frame "心跳包", Default {
    }
    frame "提取数采仪时间" {
      (unwired) ""
      n228 = global read "全局1.vi" "枚举"() -> (w360:enum16{"返回请求应答", "上传数据", "返回执行结果"})
      n229 = case shown="\"上传数据\"" w360 {
        tunnel: ["QnRtn=1" w362 "ExeRtn=1"] -> w359
        frame "返回请求应答", Default {
        }
        frame "上传数据" {
          n230 = Get Date/Time In Seconds() -> (seconds since 1Jan1904=w366:timestamp)
          n231 = Format Date/Time String(time format string (%c)="%Y%m%d%H%M%S" ("时间格式字符串(%c)"), seconds (now)=w366) -> (date/time string=w363:string)  [unwired: 1 in]
          n232 = Concatenate Strings("SystemTime=", w363) -> (w362:string)
        }
        frame "返回执行结果" {
        }
      }
    }
    frame "获取软件版本号" {
      (unwired) ""
      n233 = global read "全局1.vi" "枚举"() -> (w369:enum16{"返回请求应答", "上传数据", "返回执行结果"})
      n234 = case shown="\"上传数据\"" w369 {
        tunnel: ["QnRtn=1" w372 "ExeRtn=1"] -> w368
        frame "返回请求应答", Default {
        }
        frame "上传数据" {
          n235 = global read "全局1.vi" "版本信息"() -> (w371:string)
          n236 = Concatenate Strings("Version=", w371) -> (w372:string)
        }
        frame "返回执行结果" {
        }
      }
    }
    frame "获取仪器软件版本号" {
      (unwired) ""
      n237 = global read "全局1.vi" "枚举"() -> (w376:enum16{"返回请求应答", "上传数据", "返回执行结果"})
      n238 = case shown="\"上传数据\"" w376 {
        tunnel: ["QnRtn=1" w382 "ExeRtn=1"] -> w375
        frame "返回请求应答", Default {
        }
        frame "上传数据" {
          n239 = global read "全局1.vi" "固件版本"() -> (w381:T7)
          n240 = global read "全局 小时数据发送次数.vi" "小时数据发送次数"() -> (w379:i32)
          n241 = Cluster To Array(cluster=w381) -> (array=w380:string[])
          n242 = Index Array(array=w380, index=w379) -> (element=w378:string)
          n243 = Concatenate Strings("FirmwareVersion=", w378) -> (w382:string)
        }
        frame "返回执行结果" {
        }
      }
    }
    frame "提取实时数据间隔" {
      (unwired) ""
      n244 = global read "全局1.vi" "枚举"() -> (w386:enum16{"返回请求应答", "上传数据", "返回执行结果"})
      n245 = case shown="\"上传数据\"" w386 {
        tunnel: ["QnRtn=1" w390 "ExeRtn=1"] -> w385
        frame "返回请求应答", Default {
        }
        frame "上传数据" {
          n246 = global read "实时数据发送间隔全局.vi" "实时数据发送间隔"() -> (w389:u32)
          n247 = Number To Decimal String(number=w389) -> (decimal integer string=w388:string)  [unwired: 1 in]
          n248 = Concatenate Strings("RtdInterval=", w388) -> (w390:string)
        }
        frame "返回执行结果" {
        }
      }
    }
    frame "实时数据" {
      # "包含质控数据主动上传"
      n249 = global read "全局 实时数据参数.vi" "实时数据参数"() -> (w395:string)
      n250 = case shown="\"平行样测试\"" w395 {
        tunnel: [w399 w424 w449 w480 w504 w525] -> w396
        tunnel: w394 -> [w398 w423 w448 w478 w502 w523]
        tunnel: w393 -> [w397 w422 w447 w477 w501 w522]
        frame "水样测试", Default {
          n251 = global read "全局1.vi" "枚举"() -> (w400:enum16{"返回请求应答", "上传数据", "返回执行结果"})
          n252 = case shown="\"上传数据\"" w400 {
            tunnel: ["QnRtn=1" w418 "ExeRtn=1"] -> w399
            tunnel: w398 -> [_ w404 _]
            tunnel: w397 -> [_ w402 _]
            frame "返回请求应答", Default {
            }
            frame "上传数据" {
              n253 = call "数据发送组合-20200825 (子VI).vi"("枚举"=T4."实时数据", "插值后的数组元素"=w404) -> ("字符串"=w405:string)  [unwired: 9 in]
              n254 = global read "全局 小时数据发送次数.vi" "小时数据发送次数"() -> (w416:i32)
              n255 = Index Array(array=w402, index (row)=w416) -> (element=w415:string[])  [unwired: 1 in]
              n256 = Index Array(array=w415, index=0 ("索引")) -> (element=w413:string)
              n257 = call "规范时间戳.vi"("字符串"=w413) -> ("result string"=w411:string)  [unwired: 10 in]
              n258 = Empty String/Path?(string/path=w405) -> (empty?=w417:bool)
              n259 = Format Into String(format string="DataTime=%s;", w411) -> (resulting string=w410:string)  [unwired: 2 in, 1 out]
              n260 = Concatenate Strings(w410, w405) -> (w407:string)
              n261 = String Length(string=w407) -> (length=w409:i32)
              n262 = Decrement(x=w409) -> (x-1=w408:i32)
              n263 = String Subset(string=w407, length (rest)=w408) -> (substring=w406:string)  [unwired: 1 in]
              n264 = case shown="False" w417 {
                tunnel: [w419 ""] -> w418
                tunnel: w406 -> [w419 _]
                frame False {
                }
                frame True {
                }
              }
            }
            frame "返回执行结果" {
            }
          }
        }
        frame "平行样测试" {
          n265 = global read "全局1.vi" "枚举"() -> (w425:enum16{"返回请求应答", "上传数据", "返回执行结果"})
          n266 = case shown="\"上传数据\"" w425 {
            tunnel: ["QnRtn=1" w437 "ExeRtn=1"] -> w424
            tunnel: w422 -> [_ w431 _]
            tunnel: w423 -> [_ w428 _]
            frame "返回请求应答", Default {
            }
            frame "上传数据" {
              # "CODMn"
              n267 = call "数据发送组合-20200825 (子VI).vi"("枚举"=T4."平行样测试", "插值后的数组元素"=w428) -> ("字符串"=w427:string)  [unwired: 9 in]
              n268 = global read "全局 小时数据发送次数.vi" "小时数据发送次数"() -> (w430:i32)
              n269 = Index Array(array=w431, index (row)=w430) -> (element=w435:string[])  [unwired: 1 in]
              n270 = Index Array(array=w435, index=0 ("索引")) -> (element=w432:string)
              n271 = call "规范时间戳.vi"("字符串"=w432) -> ("result string"=w433:string)  [unwired: 10 in]
              n272 = Empty String/Path?(string/path=w432) -> (empty?=w436:bool)
              n273 = Format Into String(format string="DataTime=%s;%s" ("格式字符串"), w433, w427) -> (resulting string=w438:string)  [unwired: 2 in, 1 out]
              n274 = case shown="True" w436 {
                tunnel: [w442 ""] -> w437
                tunnel: w438 -> [w442 _]
                frame False {
                  n275 = global read "全局 小时数据发送次数.vi" "小时数据发送次数"() -> (w441:i32)
                  n276 = Increment(x=w441) -> (x+1=w440:i32)
                  n277 = global write "全局 小时数据发送次数.vi" "小时数据发送次数"(w440) -> ()
                }
                frame True {
                  n278 = global read "全局 小时数据发送次数.vi" "小时数据发送次数"() -> (w444:i32)
                  n279 = Increment(x=w444) -> (x+1=w443:i32)
                  n280 = global write "全局 小时数据发送次数.vi" "小时数据发送次数"(w443) -> ()
                }
              }
            }
            frame "返回执行结果" {
            }
          }
        }
        frame "集成干预测试" {
          n281 = global read "全局1.vi" "枚举"() -> (w450:enum16{"返回请求应答", "上传数据", "返回执行结果"})
          n282 = case shown="\"上传数据\"" w450 {
            tunnel: ["QnRtn=1" w463 "ExeRtn=1"] -> w449
            tunnel: w447 -> [_ w457 _]
            tunnel: w448 -> [_ w454 _]
            frame "返回请求应答", Default {
            }
            frame "上传数据" {
              # "CODMn"
              n283 = global read "全局 小时数据发送次数.vi" "小时数据发送次数"() -> (w456:i32)
              n284 = call "数据发送组合-20200825 (子VI).vi"("枚举"=T4."集成干预测试", "插值后的数组元素"=w454) -> ("字符串"=w453:string)  [unwired: 9 in]
              n285 = Index Array(array=w457, index (row)=w456) -> (element=w461:string[])  [unwired: 1 in]
              n286 = global read "断电保存全局.vi" "应用环境"() -> (w452:T8)
              n287 = Index Array(array=w461, index=0 ("索引")) -> (element=w458:string)
              n288 = case shown="\"GB212\", Default" w452 {
                tunnel: [w467 w468] -> w459
                tunnel: w458 -> [w466 w469]
                frame "STD" {
                  n289 = call "规范时间戳.vi"("字符串"=w466) -> ("result string"=w467:string)  [unwired: 10 in]
                }
                frame "GB212", Default {
                  n290 = call "规范分钟数据时间戳.vi"("字符串"=w469) -> ("result string"=w468:string)  [unwired: 10 in]
                }
              }
              n291 = Empty String/Path?(string/path=w458) -> (empty?=w462:bool)
              n292 = Format Into String(format string="DataTime=%s;%s" ("格式字符串"), w459, w453) -> (resulting string=w464:string)  [unwired: 2 in, 1 out]
              n293 = case shown="False" w462 {
                tunnel: [w472 ""] -> w463
                tunnel: w464 -> [w472 _]
                frame False {
                  n294 = global read "全局 小时数据发送次数.vi" "小时数据发送次数"() -> (w471:i32)
                  n295 = Increment(x=w471) -> (x+1=w470:i32)
                  n296 = global write "全局 小时数据发送次数.vi" "小时数据发送次数"(w470) -> ()
                }
                frame True {
                  n297 = global read "全局 小时数据发送次数.vi" "小时数据发送次数"() -> (w474:i32)
                  n298 = Increment(x=w474) -> (x+1=w473:i32)
                  n299 = global write "全局 小时数据发送次数.vi" "小时数据发送次数"(w473) -> ()
                }
              }
            }
            frame "返回执行结果" {
            }
          }
        }
        frame "加标回收测试" {
          n300 = global read "全局1.vi" "枚举"() -> (w479:enum16{"返回请求应答", "上传数据", "返回执行结果"})
          n301 = case shown="\"上传数据\"" w479 {
            tunnel: ["QnRtn=1" w490 "ExeRtn=1"] -> w480
            tunnel: w477 -> [_ w485 _]
            tunnel: w478 -> [_ w487 _]
            frame "返回请求应答", Default {
            }
            frame "上传数据" {
              # "w01001-Check=63.0,w01001-WaterTime=20160801080000,w01001-Water=45.23,w01001-Chroma=1000,w01001-Volume=0.2,w01001-DVolume=200,w01003-Flag=N;"
              # "CODMn"
              n302 = global read "全局 小时数据发送次数.vi" "小时数据发送次数"() -> (w484:i32)
              n303 = call "加标回收数据组合 (子VI).vi"("小时数据发送次数"=w484, "数据"=w485, "污染物编码"="CODMn") -> ("datatime"=w483:string)  [unwired: 7 in, 1 out]
              n304 = call "规范时间戳.vi"("字符串"=w483) -> ("result string"=w492:string)  [unwired: 10 in]
              n305 = Empty String/Path?(string/path=w492) -> (empty?=w489:bool)
              n306 = call "数据发送组合-20200825 (子VI).vi"("枚举"=T4."加标回收测试", "插值后的数组元素"=w487) -> ("字符串"=w486:string)  [unwired: 9 in]
              n307 = Format Into String(format string="DataTime=%s;%s" ("格式字符串"), w492, w486) -> (resulting string=w491:string)  [unwired: 2 in, 1 out]
              n308 = case shown="True" w489 {
                tunnel: [w496 ""] -> w490
                tunnel: w491 -> [w496 _]
                frame False {
                  n309 = global read "全局 小时数据发送次数.vi" "小时数据发送次数"() -> (w495:i32)
                  n310 = Increment(x=w495) -> (x+1=w494:i32)
                  n311 = global write "全局 小时数据发送次数.vi" "小时数据发送次数"(w494) -> ()
                }
                frame True {
                  n312 = global read "全局 小时数据发送次数.vi" "小时数据发送次数"() -> (w498:i32)
                  n313 = Increment(x=w498) -> (x+1=w497:i32)
                  n314 = global write "全局 小时数据发送次数.vi" "小时数据发送次数"(w497) -> ()
                }
              }
            }
            frame "返回执行结果" {
            }
          }
        }
        frame "核查数据" {
          n315 = global read "全局1.vi" "枚举"() -> (w503:enum16{"返回请求应答", "上传数据", "返回执行结果"})
          n316 = case shown="\"上传数据\"" w503 {
            tunnel: ["QnRtn=1" w514 "ExeRtn=1"] -> w504
            tunnel: w502 -> [_ w507 _]
            tunnel: w501 -> [_ w506 _]
            frame "返回请求应答", Default {
            }
            frame "上传数据" {
              # "将非空数组的时间戳写入"
              n317 = global read "全局 小时数据发送次数.vi" "小时数据发送次数"() -> (w510:i32)
              n318 = Index Array(array=w506, index (row)=w510) -> (element=w513:string[])  [unwired: 1 in]
              n319 = call "数据发送组合-20200825 (子VI).vi"("枚举"=T4."核查数据", "插值后的数组元素"=w507) -> ("字符串"=w508:string)  [unwired: 9 in]
              n320 = Index Array(array=w513, index=0 ("索引")) -> (element=w512:string)
              n321 = call "规范分钟数据时间戳.vi"("字符串"=w512) -> ("result string"=w511:string)  [unwired: 10 in]
              n322 = Empty String/Path?(string/path=w511) -> (empty?=w516:bool)
              n323 = Format Into String(format string="DataTime=%s;%s" ("格式字符串"), w511, w508) -> (resulting string=w515:string)  [unwired: 2 in, 1 out]
              n324 = case shown="False" w516 {
                tunnel: [w519 ""] -> w514
                tunnel: w515 -> [w519 _]
                frame False {
                }
                frame True {
                }
              }
            }
            frame "返回执行结果" {
            }
          }
        }
        frame "空白测试", "跨度核查" {
          n325 = global read "全局1.vi" "枚举"() -> (w524:enum16{"返回请求应答", "上传数据", "返回执行结果"})
          n326 = case shown="\"上传数据\"" w524 {
            tunnel: ["QnRtn=1" w536 "ExeRtn=1"] -> w525
            tunnel: w523 -> [_ w532 _]
            tunnel: w522 -> [_ w530 _]
            frame "返回请求应答", Default {
            }
            frame "上传数据" {
              n327 = global read "全局 小时数据发送次数.vi" "小时数据发送次数"() -> (w534:i32)
              n328 = call "数据发送组合-20200825 (子VI).vi"("枚举"=T4."空白零点跨度数据", "插值后的数组元素"=w532) -> ("字符串"=w531:string)  [unwired: 9 in]
              n329 = Index Array(array=w530, index (row)=w534) -> (element=w540:string[])  [unwired: 1 in]
              n330 = Index Array(array=w540, index #1=0 ("索引"), index #2=3 ("索引"), index #3=5 ("索引")) -> (element #1=w528:string, element #3=w529:string)  [unwired: 1 out]
              n331 = case shown="\"pf\"" w529 {
                tunnel: [w543 w545] -> w527
                tunnel: w528 -> [w544 w546]
                frame "假", Default {
                  n332 = call "规范小时时间戳.vi"("字符串"=w544) -> ("result string"=w543:string)  [unwired: 10 in]
                }
                frame "pf" {
                  # "pf数据时间戳不变"
                  n333 = call "规范时间戳.vi"("字符串"=w546) -> ("result string"=w545:string)  [unwired: 10 in]
                }
              }
              n334 = Empty String/Path?(string/path=w527) -> (empty?=w537:bool)
              n335 = Format Into String(format string="DataTime=%s;%s" ("格式字符串"), w527, w531) -> (resulting string=w535:string)  [unwired: 2 in, 1 out]
              n336 = case shown="False" w537 {
                tunnel: [w547 ""] -> w536
                tunnel: w535 -> [w547 _]
                frame False {
                }
                frame True {
                }
              }
            }
            frame "返回执行结果" {
            }
          }
        }
      }
    }
    frame "小时数据" {
      # "发送小时数据"
      n337 = global read "全局1.vi" "枚举"() -> (w553:enum16{"返回请求应答", "上传数据", "返回执行结果"})
      n338 = case shown="\"上传数据\"" w553 {
        tunnel: ["QnRtn=1" w576 "ExeRtn=1"] -> w551
        tunnel: w552 -> [_ w566 _]
        tunnel: w550 -> [_ w564 _]
        frame "返回请求应答", Default {
          (unwired) 0 ("当前包数")
          n339 = global read "全局 数据数组大小.vi" "数据数组大小"() -> (w554:i32)
          n340 = global write "全局1.vi" "枚举"(enum16{"返回请求应答", "上传数据", "返回执行结果"}."上传数据" ("枚举")) -> ()
          n341 = Equal To 0?(x=w554) -> (x = 0?=w555:bool)
          n342 = case shown="True" w555 {
            frame False {
            }
            frame True {
              n343 = global read "全局 小时数据发送次数.vi" "小时数据发送次数"() -> (w559:i32)
              n344 = Increment(x=w559) -> (x+1=w558:i32)
              n345 = global write "全局 小时数据发送次数.vi" "小时数据发送次数"(w558) -> ()
            }
          }
        }
        frame "上传数据" {
          n346 = global read "全局 小时数据发送次数.vi" "小时数据发送次数"() -> (w575:i32)
          n347 = call "数据发送组合-20200825 (子VI).vi"("枚举"=enum16{"小时数据", "实时数据"}."小时数据", "插值后的数组元素"=w566) -> ("字符串"=w563:string)  [unwired: 9 in]
          n348 = Index Array(array=w564, index (row)=w575) -> (element=w574:string[])  [unwired: 1 in]
          n349 = Index Array(array=w574, index=0 ("索引")) -> (element=w561:string)
          n350 = global read "全局 水样时间.vi" "选择发送的参数"() -> (w562:string)
          n351 = case shown="\"水深\"" w562 {
            tunnel: [w578 w581] -> w560
            tunnel: w561 -> [w579 w580]
            frame "水深" {
              n352 = call "规范分钟数据时间戳.vi"("字符串"=w579) -> ("result string"=w578:string)  [unwired: 10 in]
            }
            frame "真", Default {
              n353 = call "规范小时时间戳.vi"("字符串"=w580) -> ("result string"=w581:string)  [unwired: 10 in]
            }
          }
          n354 = Empty String/Path?(string/path=w563) -> (empty?=w577:bool)
          n355 = Format Into String(format string="DataTime=%s;", w560) -> (resulting string=w572:string)  [unwired: 2 in, 1 out]
          n356 = Concatenate Strings(w572, w563) -> (w568:string)
          n357 = String Length(string=w568) -> (length=w570:i32)
          n358 = Decrement(x=w570) -> (x-1=w569:i32)
          n359 = String Subset(string=w568, length (rest)=w569) -> (substring=w567:string)  [unwired: 1 in]
          n360 = case shown="False" w577 {
            tunnel: [w582 ""] -> w576
            tunnel: w567 -> [w582 _]
            frame False {
            }
            frame True {
            }
          }
        }
        frame "返回执行结果" {
          (unwired) 0 ("当前包数")
          n361 = global write "全局1.vi" "枚举"(enum16{"返回请求应答", "上传数据", "返回执行结果"}."返回请求应答" ("枚举")) -> ()
        }
      }
    }
    frame "剖面数据" {
      # "{\"data\":[{\"time\":\"21-06-08 01:08:00\",\"w01010Value\":23,\"w01001Value\":7,\"w01009Value\":6,\"w01014Value\":22,\"w01003Value\":100,\"depth\":0.5,\"row\":3},{\"time\":\"21-06-08 01:08:00\",\"w01010Value\":22,\"w01001Value\":8,\"w01009Value\":7,\"w01014Value\":25,\"w01003Value\":96,\"depth\":0.8,\"row\":3},{\"time\":\"21-06-08 01:08:00\",\"w01010Value\":21,\"w01001Value\":7,\"w01009Value\":7,\"w01014Value\":24,\"w01003Value\":95,\"depth\":1,\"row\":3}]}"
      # "发送剖面数据"
      n362 = global read "全局1.vi" "枚举"() -> (w586:enum16{"返回请求应答", "上传数据", "返回执行结果"})
      n363 = case shown="\"上传数据\"" w586 {
        tunnel: ["QnRtn=1" w597 "ExeRtn=1"] -> w587
        frame "返回请求应答", Default {
          (unwired) 0 ("当前包数")
          n364 = global read "全局 数据数组大小.vi" "数据数组大小"() -> (w588:i32)
          n365 = global write "全局1.vi" "枚举"(enum16{"返回请求应答", "上传数据", "返回执行结果"}."上传数据" ("枚举")) -> ()
          n366 = Equal To 0?(x=w588) -> (x = 0?=w589:bool)
          n367 = case shown="True" w589 {
            frame False {
            }
            frame True {
              n368 = global read "全局 小时数据发送次数.vi" "小时数据发送次数"() -> (w593:i32)
              n369 = Increment(x=w593) -> (x+1=w592:i32)
              n370 = global write "全局 小时数据发送次数.vi" "小时数据发送次数"(w592) -> ()
            }
          }
        }
        frame "上传数据" {
          n371 = global read "断电保存全局.vi" "数据发送协议"() -> (w596:enum16{"2005-212协议", "2017-212协议"})
          n372 = case shown="\"2017-212协议\", Default" w596 {
            tunnel: ["" ("编码输出") w618] -> w595
            tunnel: [_ w614] -> w594
            frame "2005-212协议" {
            }
            frame "2017-212协议", Default {
              w608 = 0 ("索引 (行)")
              (unwired) "w01010" ("污染物编码")
              (unwired) "w01016" ("污染物编码")
              (unwired) "w01003" ("污染物编码")
              (unwired) "w01014" ("污染物编码")
              # "时间,测量模式,数据类型,数据标识,层数,Temp,SpCond,Cond,Sal,TDS,pH,pHmV,ORP,ODO%,ODOmg/L,Turb,Chla,Depth,"
              n373 = global read "全局 小时数据发送次数.vi" "小时数据发送次数"() -> (w617:i32)
              n374 = global read "全局 所有参数.vi" "剖面多参数"() -> (w605:string[][])
              n375 = global read "全局 数据数组大小.vi" "分包标准"() -> (w616:i32)
              n376 = global read "全局 所有参数.vi" "columns"() -> (w615:string[])
              n377 = Array Subset(array=w605, index (row)=w617, length (row)=w616) -> (w614:string[][])  [unwired: 2 in]
              n378 = Array Subset(array=w605, index (row)=0 ("索引"), length (row)=1 ("长度")) -> (w603:string[][])  [unwired: 2 in]
              n379 = call "新剖面数据组合.vi"("columns"=w615, "剖面数据"=w614) -> ("结果字符串"=w612:string)  [unwired: 9 in]
              n380 = Index Array(array=w603, index (row) #1=w608, index (col) #1=0 ("索引 (行)"), index (row) #2=w608, index (col) #2=1 ("索引 (列)"), index (row) #3=w608, index (col) #3=2 ("索引 (列)")) -> (element #1=w601:string, element #2=w607:string, element #3=w606:string)
              n381 = call "规范小时时间戳.vi"("字符串"=w601) -> ("result string"=w600:string)  [unwired: 10 in]
              n382 = Empty String/Path?(string/path=w612) -> (empty?=w619:bool)
              n383 = Format Into String(format string="DataTime=%s;total=%s;waterdepth=%s;data=%s", w600, w607, w606, w612) -> (resulting string=w611:string)  [unwired: 2 in, 1 out]
              n384 = case shown="True" w619 {
                tunnel: [w621 ""] -> w618
                tunnel: w611 -> [w621 _]
                frame False {
                }
                frame True {
                }
              }
            }
          }
          n385 = Empty String/Path?(string/path=w595) -> (empty?=w598:bool)
          n386 = case shown="False" w598 {
            tunnel: [w628 ""] -> w597
            tunnel: w595 -> [w628 _]
            tunnel: w594 -> [w627 w629]
            frame False {
              n387 = Array Size(array=w627) -> (size(s)=w626:i32[])
              n388 = global read "全局 小时数据发送次数.vi" "小时数据发送次数"() -> (w624:i32)
              n389 = Index Array(array=w626) -> (element=w625:i32)  [unwired: 1 in]
              n390 = Add(x=w625, y=w624) -> (x+y=w623:i32)
              n391 = global write "全局 小时数据发送次数.vi" "小时数据发送次数"(w623) -> ()
            }
            frame True {
              n392 = Array Size(array=w629) -> (size(s)=w633:i32[])
              n393 = global read "全局 小时数据发送次数.vi" "小时数据发送次数"() -> (w631:i32)
              n394 = Index Array(array=w633) -> (element=w632:i32)  [unwired: 1 in]
              n395 = Add(x=w632, y=w631) -> (x+y=w630:i32)
              n396 = global write "全局 小时数据发送次数.vi" "小时数据发送次数"(w630) -> ()
            }
          }
        }
        frame "返回执行结果" {
          (unwired) 0 ("当前包数")
          n397 = global write "全局1.vi" "枚举"(enum16{"返回请求应答", "上传数据", "返回执行结果"}."返回请求应答" ("枚举")) -> ()
        }
      }
    }
    frame "海流计" {
      # "发送海流计剖面数据"
      n398 = global read "全局1.vi" "枚举"() -> (w637:enum16{"返回请求应答", "上传数据", "返回执行结果"})
      n399 = case shown="\"上传数据\"" w637 {
        tunnel: ["QnRtn=1" w648 "ExeRtn=1"] -> w638
        frame "返回请求应答", Default {
          n400 = global write "全局1.vi" "枚举"(enum16{"返回请求应答", "上传数据", "返回执行结果"}."上传数据" ("枚举")) -> ()
          n401 = disable-structure shown="禁用" {
            frame Disabled {
              (unwired) 0 ("当前包数")
              n402 = global read "全局 数据数组大小.vi" "数据数组大小"() -> (w641:i32)
              n403 = Equal To 0?(x=w641) -> (x = 0?=w642:bool)
              n404 = case shown="True" w642 {
                frame False {
                }
                frame True {
                  n405 = global read "全局 小时数据发送次数.vi" "小时数据发送次数"() -> (w644:i32)
                  n406 = Increment(x=w644) -> (x+1=w643:i32)
                  n407 = global write "全局 小时数据发送次数.vi" "小时数据发送次数"(w643) -> ()
                }
              }
            }
            frame Enabled {
            }
          }
        }
        frame "上传数据" {
          n408 = global read "断电保存全局.vi" "数据发送协议"() -> (w647:enum16{"2005-212协议", "2017-212协议"})
          n409 = case shown="\"2017-212协议\", Default" w647 {
            tunnel: ["" ("编码输出") w652] -> w646
            tunnel: [_ w651] -> w645
            frame "2005-212协议" {
            }
            frame "2017-212协议", Default {
              # "上传的数据进行分包"
              n410 = disable-structure shown="Enabled" {
                disable-tunnel: [w655 w660] -> w652
                disable-tunnel: [w654 _] -> w651
                frame Disabled {
                  n411 = call "海流计数据拆分.vi"() -> ("不再发送"=w653:bool, "当前要发送的海流计参数"=w654:string[][])  [unwired: 10 in]
                  n412 = case shown="False" w653 {
                    tunnel: [w658 ""] -> w655
                    tunnel: w654 -> [w657 _]
                    tunnel: w653 -> [w656 _]
                    frame False {
                      n413 = call "海流计数据组合.vi"("不再发送"=w656, "要发送的海流计参数"=w657) -> ("发送的信息"=w658:string)  [unwired: 9 in]
                    }
                    frame True {
                    }
                  }
                  n414 = global write "全局 数据数组大小.vi" "海流计数据发送完毕"(w653) -> ()
                }
                frame Enabled {
                  n415 = call "海流计数据编码.vi"() -> ("发送的信息"=w660:string)  [unwired: 11 in]
                }
              }
            }
          }
          n416 = Empty String/Path?(string/path=w646) -> (empty?=w649:bool)
          n417 = case shown="False" w649 {
            tunnel: [w661 ""] -> w648
            tunnel: w646 -> [w661 _]
            tunnel: w645 -> [_ _]
            frame False {
            }
            frame True {
            }
          }
        }
        frame "返回执行结果" {
          (unwired) 0 ("当前包数")
          n418 = global write "全局1.vi" "枚举"(enum16{"返回请求应答", "上传数据", "返回执行结果"}."返回请求应答" ("枚举")) -> ()
        }
      }
    }
    frame "ADCP过程数据" {
      # "发送海流计剖面数据"
      n419 = global read "全局1.vi" "枚举"() -> (w665:enum16{"返回请求应答", "上传数据", "返回执行结果"})
      n420 = case shown="\"上传数据\"" w665 {
        tunnel: ["QnRtn=1" w675 "ExeRtn=1"] -> w666
        frame "返回请求应答", Default {
          (unwired) 0 ("当前包数")
          n421 = global write "全局1.vi" "枚举"(enum16{"返回请求应答", "上传数据", "返回执行结果"}."上传数据" ("枚举")) -> ()
          n422 = disable-structure shown="禁用" {
            frame Disabled {
              n423 = global read "全局 数据数组大小.vi" "数据数组大小"() -> (w669:i32)
              n424 = Equal To 0?(x=w669) -> (x = 0?=w670:bool)
              n425 = case shown="True" w670 {
                frame False {
                }
                frame True {
                  n426 = global read "全局 小时数据发送次数.vi" "小时数据发送次数"() -> (w672:i32)
                  n427 = Increment(x=w672) -> (x+1=w671:i32)
                  n428 = global write "全局 小时数据发送次数.vi" "小时数据发送次数"(w671) -> ()
                }
              }
            }
            frame Enabled {
            }
          }
        }
        frame "上传数据" {
          n429 = global read "断电保存全局.vi" "数据发送协议"() -> (w674:enum16{"2005-212协议", "2017-212协议"})
          n430 = case shown="\"2017-212协议\", Default" w674 {
            tunnel: ["" ("编码输出") w678] -> w673
            frame "2005-212协议" {
            }
            frame "2017-212协议", Default {
              # "上传的数据进行分包"
              n431 = call "ADCP过程数据编码.vi"() -> ("发送的信息"=w678:string)  [unwired: 11 in]
            }
          }
          n432 = Empty String/Path?(string/path=w673) -> (empty?=w676:bool)
          n433 = case shown="False" w676 {
            tunnel: [w679 ""] -> w675
            tunnel: w673 -> [w679 _]
            frame False {
            }
            frame True {
            }
          }
        }
        frame "返回执行结果" {
          (unwired) 0 ("当前包数")
          n434 = global write "全局1.vi" "枚举"(enum16{"返回请求应答", "上传数据", "返回执行结果"}."返回请求应答" ("枚举")) -> ()
        }
      }
    }
    frame "剖面多参数H" {
      # "发送小时数据"
      n435 = global read "全局1.vi" "枚举"() -> (w683:enum16{"返回请求应答", "上传数据", "返回执行结果"})
      n436 = case shown="\"上传数据\"" w683 {
        tunnel: ["QnRtn=1" w693 "ExeRtn=1"] -> w684
        frame "返回请求应答", Default {
          (unwired) 0 ("当前包数")
          n437 = global read "全局 数据数组大小.vi" "数据数组大小"() -> (w685:i32)
          n438 = global write "全局1.vi" "枚举"(enum16{"返回请求应答", "上传数据", "返回执行结果"}."上传数据" ("枚举")) -> ()
          n439 = Equal To 0?(x=w685) -> (x = 0?=w686:bool)
          n440 = case shown="True" w686 {
            frame False {
            }
            frame True {
              n441 = global read "全局 小时数据发送次数.vi" "小时数据发送次数"() -> (w690:i32)
              n442 = Increment(x=w690) -> (x+1=w689:i32)
              n443 = global write "全局 小时数据发送次数.vi" "小时数据发送次数"(w689) -> ()
            }
          }
        }
        frame "上传数据" {
          n444 = global read "断电保存全局.vi" "数据发送协议"() -> (w692:enum16{"2005-212协议", "2017-212协议"})
          n445 = case shown="\"2017-212协议\", Default" w692 {
            tunnel: ["" ("编码输出") w699] -> w691
            frame "2005-212协议" {
            }
            frame "2017-212协议", Default {
              (unwired) "w01010" ("污染物编码")
              (unwired) "w01016" ("污染物编码")
              (unwired) "w01003" ("污染物编码")
              (unwired) "w01009" ("污染物编码")
              (unwired) "w01001" ("污染物编码")
              (unwired) "w01014" ("污染物编码")
              (unwired) "w01100" ("污染物编码")
              # "时间,测量模式,数据类型,数据标识,层数,Temp,SpCond,Cond,Sal,TDS,pH,pHmV,ORP,ODO%,ODOmg/L,Turb,Chla,Depth,"
              n446 = global read "全局 小时数据发送次数.vi" "小时数据发送次数"() -> (w717:i32)
              n447 = global read "全局 所有参数.vi" "剖面多参数"() -> (w720:string[][])
              n448 = Index Array(array=w720, index (row)=w717) -> (element=w718:string[])  [unwired: 1 in]
              n449 = Index Array(array=w718, index #1=0 ("索引")) -> (element #1=w702:string, element #3=w716:string, element #4=w715:string, element #5=w714:string, element #6=w713:string, element #7=w712:string, element #11=w710:string, element #13=w709:string, element #15=w708:string, element #16=w707:string, element #17=w706:string, element #18=w696:string)  [unwired: 17 in, 6 out]
              n450 = call "规范小时时间戳.vi"("字符串"=w702) -> ("result string"=w703:string)  [unwired: 10 in]
              n451 = Build Array(w713, w712, w710, w709, w708, w707, w706, w696) -> (w711:string[])
              n452 = call "剖面多参数组合(子VI).vi"("数据类型实时小时"="-Avg=", "数据值"=w711, "层数"=w714, "数据标识"=w715, "数据类型"=w716) -> ("编码输出"=w698:string)  [unwired: 6 in]
              n453 = Format Into String(format string="DataTime=%s;", w703) -> (resulting string=w704:string)  [unwired: 2 in, 1 out]
              n454 = Empty String/Path?(string/path=w698) -> (empty?=w701:bool)
              n455 = Concatenate Strings(w704, w698) -> (w700:string)
              n456 = case shown="True" w701 {
                tunnel: [w721 ""] -> w699
                tunnel: w700 -> [w721 _]
                frame False {
                }
                frame True {
                }
              }
            }
          }
          n457 = Empty String/Path?(string/path=w691) -> (empty?=w694:bool)
          n458 = case shown="False" w694 {
            tunnel: [w725 ""] -> w693
            tunnel: w691 -> [w725 _]
            frame False {
              n459 = global read "全局 小时数据发送次数.vi" "小时数据发送次数"() -> (w724:i32)
              n460 = Increment(x=w724) -> (x+1=w723:i32)
              n461 = global write "全局 小时数据发送次数.vi" "小时数据发送次数"(w723) -> ()
            }
            frame True {
              n462 = global read "全局 小时数据发送次数.vi" "小时数据发送次数"() -> (w727:i32)
              n463 = Increment(x=w727) -> (x+1=w726:i32)
              n464 = global write "全局 小时数据发送次数.vi" "小时数据发送次数"(w726) -> ()
            }
          }
        }
        frame "返回执行结果" {
          (unwired) 0 ("当前包数")
          n465 = global write "全局1.vi" "枚举"(enum16{"返回请求应答", "上传数据", "返回执行结果"}."返回请求应答" ("枚举")) -> ()
        }
      }
    }
    frame "剖面多参数S" {
      # "发送实时数据"
      n466 = global read "全局1.vi" "枚举"() -> (w731:enum16{"返回请求应答", "上传数据", "返回执行结果"})
      n467 = case shown="\"上传数据\"" w731 {
        tunnel: ["QnRtn=1" w741 "ExeRtn=1"] -> w732
        frame "返回请求应答", Default {
          (unwired) 0 ("当前包数")
          n468 = global read "全局 数据数组大小.vi" "数据数组大小"() -> (w733:i32)
          n469 = global write "全局1.vi" "枚举"(enum16{"返回请求应答", "上传数据", "返回执行结果"}."上传数据" ("枚举")) -> ()
          n470 = Equal To 0?(x=w733) -> (x = 0?=w734:bool)
          n471 = case shown="True" w734 {
            frame False {
            }
            frame True {
              n472 = global read "全局 小时数据发送次数.vi" "小时数据发送次数"() -> (w738:i32)
              n473 = Increment(x=w738) -> (x+1=w737:i32)
              n474 = global write "全局 小时数据发送次数.vi" "小时数据发送次数"(w737) -> ()
            }
          }
        }
        frame "上传数据" {
          n475 = global read "断电保存全局.vi" "数据发送协议"() -> (w740:enum16{"2005-212协议", "2017-212协议"})
          n476 = case shown="\"2017-212协议\", Default" w740 {
            tunnel: ["" ("编码输出") w749] -> w739
            frame "2005-212协议" {
            }
            frame "2017-212协议", Default {
              (unwired) "w01010" ("污染物编码")
              (unwired) "w01016" ("污染物编码")
              (unwired) "w01003" ("污染物编码")
              (unwired) "w01009" ("污染物编码")
              (unwired) "w01001" ("污染物编码")
              (unwired) "w01014" ("污染物编码")
              (unwired) "w01100" ("污染物编码")
              # "时间,测量模式,数据类型,数据标识,层数,Temp,SpCond,Cond,Sal,TDS,pH,pHmV,ORP,ODO%,ODOmg/L,Turb,Chla,Depth,"
              n477 = global read "全局 小时数据发送次数.vi" "小时数据发送次数"() -> (w765:i32)
              n478 = global read "全局 所有参数.vi" "剖面多参数"() -> (w768:string[][])
              n479 = Index Array(array=w768, index (row)=w765) -> (element=w766:string[])  [unwired: 1 in]
              n480 = Index Array(array=w766, index #1=0 ("索引")) -> (element #1=w746:string, element #3=w764:string, element #4=w763:string, element #5=w762:string, element #6=w761:string, element #7=w760:string, element #11=w758:string, element #13=w757:string, element #15=w756:string, element #16=w755:string, element #17=w754:string, element #18=w744:string)  [unwired: 17 in, 6 out]
              n481 = call "规范时间戳.vi"("字符串"=w746) -> ("result string"=w745:string)  [unwired: 10 in]
              n482 = Build Array(w761, w760, w758, w757, w756, w755, w754, w744) -> (w759:string[])
              n483 = call "剖面多参数组合(子VI).vi"("数据类型实时小时"="-Rtd=", "数据值"=w759, "层数"=w762, "数据标识"=w763, "数据类型"=w764) -> ("编码输出"=w748:string)  [unwired: 6 in]
              n484 = Format Into String(format string="DataTime=%s;", w745) -> (resulting string=w752:string)  [unwired: 2 in, 1 out]
              n485 = Empty String/Path?(string/path=w748) -> (empty?=w751:bool)
              n486 = Concatenate Strings(w752, w748) -> (w750:string)
              n487 = case shown="False" w751 {
                tunnel: [w769 ""] -> w749
                tunnel: w750 -> [w769 _]
                frame False {
                }
                frame True {
                }
              }
            }
          }
          n488 = Empty String/Path?(string/path=w739) -> (empty?=w742:bool)
          n489 = case shown="False" w742 {
            tunnel: [w773 ""] -> w741
            tunnel: w739 -> [w773 _]
            frame False {
              n490 = global read "全局 小时数据发送次数.vi" "小时数据发送次数"() -> (w772:i32)
              n491 = Increment(x=w772) -> (x+1=w771:i32)
              n492 = global write "全局 小时数据发送次数.vi" "小时数据发送次数"(w771) -> ()
            }
            frame True {
              n493 = global read "全局 小时数据发送次数.vi" "小时数据发送次数"() -> (w775:i32)
              n494 = Increment(x=w775) -> (x+1=w774:i32)
              n495 = global write "全局 小时数据发送次数.vi" "小时数据发送次数"(w774) -> ()
            }
          }
        }
        frame "返回执行结果" {
          (unwired) 0 ("当前包数")
          n496 = global write "全局1.vi" "枚举"(enum16{"返回请求应答", "上传数据", "返回执行结果"}."返回请求应答" ("枚举")) -> ()
        }
      }
    }
    frame "提取小时数据" {
      # "发送小时数据"
      n497 = global read "全局 小时数据发送次数.vi" "小时数据发送次数"() -> (w781:i32)
      n498 = Index Array(array=w783, index (row)=w781) -> (element=w780:string[])  [unwired: 1 in]
      n499 = global read "全局1.vi" "枚举"() -> (w782:enum16{"返回请求应答", "上传数据", "返回执行结果"})
      n500 = case shown="\"上传数据\"" w782 {
        tunnel: ["QnRtn=1" w799 "ExeRtn=1"] -> w784
        tunnel: w780 -> [_ w801 _]
        tunnel: w779 -> [_ w792 _]
        frame "返回请求应答", Default {
          n501 = global read "全局 数据数组大小.vi" "数据数组大小"() -> (w785:i32)
          n502 = Equal To 0?(x=w785) -> (x = 0?=w786:bool)
          n503 = case shown="True" w786 {
            frame False {
            }
            frame True {
              n504 = global read "全局 小时数据发送次数.vi" "小时数据发送次数"() -> (w789:i32)
              n505 = Increment(x=w789) -> (x+1=w788:i32)
              n506 = global write "全局 小时数据发送次数.vi" "小时数据发送次数"(w788) -> ()
            }
          }
        }
        frame "上传数据" {
          n507 = global read "全局 水样时间.vi" "选择发送的参数"() -> (w791:string)
          n508 = Index Array(array=w801, index #2=1 ("索引")) -> (element #1=w795:string)  [unwired: 1 in, 1 out]
          n509 = case shown="\"水深\"" w791 {
            tunnel: [w803 w806] -> w796
            tunnel: w795 -> [w804 w805]
            frame "水深" {
              n510 = call "规范分钟数据时间戳.vi"("字符串"=w804) -> ("result string"=w803:string)  [unwired: 10 in]
            }
            frame "真", Default {
              n511 = call "规范小时时间戳.vi"("字符串"=w805) -> ("result string"=w806:string)  [unwired: 10 in]
            }
          }
          n512 = call "数据发送组合-20200825 (子VI).vi"("枚举"=T4."提取小时数据", "插值后的数组元素"=w792) -> ("字符串"=w793:string)  [unwired: 9 in]
          n513 = Format Into String(format string="DataTime=%s;", w796) -> (resulting string=w798:string)  [unwired: 2 in, 1 out]
          n514 = Empty String/Path?(string/path=w793) -> (empty?=w800:bool)
          n515 = Concatenate Strings(w798, w793) -> (w790:string)
          n516 = case shown="False" w800 {
            tunnel: [w809 ""] -> w799
            tunnel: w790 -> [w809 _]
            frame False {
              n517 = global read "全局 小时数据发送次数.vi" "小时数据发送次数"() -> (w808:i32)
              n518 = Increment(x=w808) -> (x+1=w807:i32)
              n519 = global write "全局 小时数据发送次数.vi" "小时数据发送次数"(w807) -> ()
            }
            frame True {
              n520 = global read "全局 小时数据发送次数.vi" "小时数据发送次数"() -> (w811:i32)
              n521 = Increment(x=w811) -> (x+1=w810:i32)
              n522 = global write "全局 小时数据发送次数.vi" "小时数据发送次数"(w810) -> ()
            }
          }
        }
        frame "返回执行结果" {
        }
      }
    }
    frame "提取实时数据" {
      # "提取实时数据"
      n523 = global read "全局 小时数据发送次数.vi" "小时数据发送次数"() -> (w816:i32)
      n524 = Index Array(array=w819, index (row)=w816) -> (element=w815:string[])  [unwired: 1 in]
      n525 = global read "全局1.vi" "枚举"() -> (w817:enum16{"返回请求应答", "上传数据", "返回执行结果"})
      n526 = case shown="\"上传数据\"" w817 {
        tunnel: ["QnRtn=1" w828 "ExeRtn=1"] -> w818
        tunnel: w815 -> [_ w834 _]
        tunnel: w814 -> [_ w826 _]
        frame "返回请求应答", Default {
          n527 = global read "全局 数据数组大小.vi" "数据数组大小"() -> (w820:i32)
          n528 = Equal To 0?(x=w820) -> (x = 0?=w821:bool)
          n529 = case shown="True" w821 {
            frame False {
            }
            frame True {
              n530 = global read "全局 小时数据发送次数.vi" "小时数据发送次数"() -> (w824:i32)
              n531 = Increment(x=w824) -> (x+1=w823:i32)
              n532 = global write "全局 小时数据发送次数.vi" "小时数据发送次数"(w823) -> ()
            }
          }
        }
        frame "上传数据" {
          n533 = Index Array(array=w834, index #1=0 ("索引"), index #2=3 ("索引"), index #3=5 ("索引")) -> (element #1=w832:string)  [unwired: 2 out]
          n534 = call "规范时间戳.vi"("字符串"=w832) -> ("result string"=w831:string)  [unwired: 10 in]
          n535 = call "数据发送组合-20200825 (子VI).vi"("枚举"=T4."提取实时数据", "插值后的数组元素"=w826) -> ("字符串"=w825:string)  [unwired: 9 in]
          n536 = Empty String/Path?(string/path=w831) -> (empty?=w830:bool)
          n537 = Format Into String(format string="DataTime=%s;%s" ("格式字符串"), w831, w825) -> (resulting string=w829:string)  [unwired: 2 in, 1 out]
          n538 = case shown="True" w830 {
            tunnel: [w838 ""] -> w828
            tunnel: w829 -> [w838 _]
            frame False {
              n539 = global read "全局 小时数据发送次数.vi" "小时数据发送次数"() -> (w840:i32)
              n540 = Increment(x=w840) -> (x+1=w839:i32)
              n541 = global write "全局 小时数据发送次数.vi" "小时数据发送次数"(w839) -> ()
            }
            frame True {
              n542 = global read "全局 小时数据发送次数.vi" "小时数据发送次数"() -> (w842:i32)
              n543 = Increment(x=w842) -> (x+1=w841:i32)
              n544 = global write "全局 小时数据发送次数.vi" "小时数据发送次数"(w841) -> ()
            }
          }
        }
        frame "返回执行结果" {
        }
      }
    }
    frame "核查数据" {
      # "提取标样核查数据"
      n545 = global read "全局 小时数据发送次数.vi" "小时数据发送次数"() -> (w848:i32)
      n546 = Index Array(array=w845, index (row)=w848) -> (element=w847:string[])  [unwired: 1 in]
      n547 = global read "全局1.vi" "枚举"() -> (w849:enum16{"返回请求应答", "上传数据", "返回执行结果"})
      n548 = case shown="\"上传数据\"" w849 {
        tunnel: ["QnRtn=1" w861 "ExeRtn=1"] -> w850
        tunnel: w847 -> [_ w867 _]
        tunnel: w846 -> [_ w857 _]
        frame "返回请求应答", Default {
          n549 = global read "全局 数据数组大小.vi" "数据数组大小"() -> (w852:i32)
          n550 = Equal To 0?(x=w852) -> (x = 0?=w851:bool)
          n551 = case shown="True" w851 {
            frame False {
            }
            frame True {
              n552 = global read "全局 小时数据发送次数.vi" "小时数据发送次数"() -> (w855:i32)
              n553 = Increment(x=w855) -> (x+1=w854:i32)
              n554 = global write "全局 小时数据发送次数.vi" "小时数据发送次数"(w854) -> ()
            }
          }
        }
        frame "上传数据" {
          # "将非空数组的时间戳写入"
          n555 = Index Array(array=w867, index #1=0 ("索引"), index #2=3 ("索引"), index #3=6 ("索引")) -> (element #1=w860:string)  [unwired: 2 out]
          n556 = call "数据发送组合-20200825 (子VI).vi"("枚举"=T4."核查数据", "插值后的数组元素"=w857) -> ("字符串"=w856:string)  [unwired: 9 in]
          n557 = call "规范时间戳.vi"("字符串"=w860) -> ("result string"=w859:string)  [unwired: 10 in]
          n558 = Empty String/Path?(string/path=w859) -> (empty?=w863:bool)
          n559 = Format Into String(format string="DataTime=%s;%s" ("格式字符串"), w859, w856) -> (resulting string=w862:string)  [unwired: 2 in, 1 out]
          n560 = case shown="False" w863 {
            tunnel: [w871 ""] -> w861
            tunnel: w862 -> [w871 _]
            frame False {
              n561 = global read "全局 小时数据发送次数.vi" "小时数据发送次数"() -> (w870:i32)
              n562 = Increment(x=w870) -> (x+1=w869:i32)
              n563 = global write "全局 小时数据发送次数.vi" "小时数据发送次数"(w869) -> ()
            }
            frame True {
              n564 = global read "全局 小时数据发送次数.vi" "小时数据发送次数"() -> (w873:i32)
              n565 = Increment(x=w873) -> (x+1=w872:i32)
              n566 = global write "全局 小时数据发送次数.vi" "小时数据发送次数"(w872) -> ()
            }
          }
        }
        frame "返回执行结果" {
        }
      }
    }
    frame "空白测试", "跨度核查", "零点核查" {
      # "提取空白测试数据/零点核查数据/跨度核查数据"
      n567 = global read "全局 小时数据发送次数.vi" "小时数据发送次数"() -> (w879:i32)
      n568 = Index Array(array=w876, index (row)=w879) -> (element=w878:string[])  [unwired: 1 in]
      n569 = global read "全局1.vi" "枚举"() -> (w880:enum16{"返回请求应答", "上传数据", "返回执行结果"})
      n570 = case shown="\"上传数据\"" w880 {
        tunnel: ["QnRtn=1" w892 "ExeRtn=1"] -> w881
        tunnel: w878 -> [_ w897 _]
        tunnel: w877 -> [_ w888 _]
        frame "返回请求应答", Default {
          (unwired) 0 ("当前包数")
          n571 = global read "全局 数据数组大小.vi" "数据数组大小"() -> (w883:i32)
          n572 = Equal To 0?(x=w883) -> (x = 0?=w882:bool)
          n573 = case shown="True" w882 {
            frame False {
            }
            frame True {
              n574 = global read "全局 小时数据发送次数.vi" "小时数据发送次数"() -> (w886:i32)
              n575 = Increment(x=w886) -> (x+1=w885:i32)
              n576 = global write "全局 小时数据发送次数.vi" "小时数据发送次数"(w885) -> ()
            }
          }
        }
        frame "上传数据" {
          # "将非空数组的时间戳写入"
          n577 = Index Array(array=w897, index #1=0 ("索引"), index #2=3 ("索引")) -> (element #1=w891:string)  [unwired: 1 out]
          n578 = call "数据发送组合-20200825 (子VI).vi"("枚举"=T4."空白零点跨度数据", "插值后的数组元素"=w888) -> ("字符串"=w887:string)  [unwired: 9 in]
          n579 = call "规范时间戳.vi"("字符串"=w891) -> ("result string"=w890:string)  [unwired: 10 in]
          n580 = Empty String/Path?(string/path=w890) -> (empty?=w894:bool)
          n581 = Format Into String(format string="DataTime=%s;%s" ("格式字符串"), w890, w887) -> (resulting string=w893:string)  [unwired: 2 in, 1 out]
          n582 = case shown="False" w894 {
            tunnel: [w901 ""] -> w892
            tunnel: w893 -> [w901 _]
            frame False {
              n583 = global read "全局 小时数据发送次数.vi" "小时数据发送次数"() -> (w900:i32)
              n584 = Increment(x=w900) -> (x+1=w899:i32)
              n585 = global write "全局 小时数据发送次数.vi" "小时数据发送次数"(w899) -> ()
            }
            frame True {
              n586 = global read "全局 小时数据发送次数.vi" "小时数据发送次数"() -> (w903:i32)
              n587 = Increment(x=w903) -> (x+1=w902:i32)
              n588 = global write "全局 小时数据发送次数.vi" "小时数据发送次数"(w902) -> ()
            }
          }
        }
        frame "返回执行结果" {
        }
      }
    }
    frame "提取加标回收" {
      # "提取加标回收数据"
      n589 = global read "全局1.vi" "枚举"() -> (w909:enum16{"返回请求应答", "上传数据", "返回执行结果"})
      n590 = case shown="\"上传数据\"" w909 {
        tunnel: ["QnRtn=1" w921 "ExeRtn=1"] -> w907
        tunnel: w908 -> [_ w923 _]
        tunnel: w906 -> [_ w915 _]
        frame "返回请求应答", Default {
          n591 = global read "全局 数据数组大小.vi" "数据数组大小"() -> (w910:i32)
          n592 = Equal To 0?(x=w910) -> (x = 0?=w911:bool)
          n593 = case shown="True" w911 {
            frame False {
            }
            frame True {
              n594 = global read "全局 小时数据发送次数.vi" "小时数据发送次数"() -> (w914:i32)
              n595 = Increment(x=w914) -> (x+1=w913:i32)
              n596 = global write "全局 小时数据发送次数.vi" "小时数据发送次数"(w913) -> ()
            }
          }
        }
        frame "上传数据" {
          # "w01001-Check=63.0,w01001-WaterTime=20160801080000,w01001-Water=45.23,w01001-Chroma=1000,w01001-Volume=0.2,w01001-DVolume=200,w01003-Flag=N;"
          # "CODMn"
          n597 = global read "全局 小时数据发送次数.vi" "小时数据发送次数"() -> (w918:i32)
          n598 = call "数据发送组合-20200825 (子VI).vi"("枚举"=T4."加标回收测试", "插值后的数组元素"=w915) -> ("字符串"=w916:string)  [unwired: 9 in]
          n599 = call "加标回收数据组合 (子VI).vi"("小时数据发送次数"=w918, "数据"=w923, "污染物编码"="w01019") -> ("datatime"=w925:string)  [unwired: 7 in, 1 out]
          n600 = call "规范时间戳.vi"("字符串"=w925) -> ("result string"=w924:string)  [unwired: 10 in]
          n601 = Empty String/Path?(string/path=w924) -> (empty?=w920:bool)
          n602 = Format Into String(format string="DataTime=%s;%s" ("格式字符串"), w924, w916) -> (resulting string=w922:string)  [unwired: 2 in, 1 out]
          n603 = case shown="True" w920 {
            tunnel: [w929 ""] -> w921
            tunnel: w922 -> [w929 _]
            frame False {
              n604 = global read "全局 小时数据发送次数.vi" "小时数据发送次数"() -> (w928:i32)
              n605 = Increment(x=w928) -> (x+1=w927:i32)
              n606 = global write "全局 小时数据发送次数.vi" "小时数据发送次数"(w927) -> ()
            }
            frame True {
              n607 = global read "全局 小时数据发送次数.vi" "小时数据发送次数"() -> (w931:i32)
              n608 = Increment(x=w931) -> (x+1=w930:i32)
              n609 = global write "全局 小时数据发送次数.vi" "小时数据发送次数"(w930) -> ()
            }
          }
        }
        frame "返回执行结果" {
        }
      }
    }
    frame "提取平行样" {
      # "提取平行样数据"
      n610 = global read "全局1.vi" "枚举"() -> (w937:enum16{"返回请求应答", "上传数据", "返回执行结果"})
      n611 = case shown="\"上传数据\"" w937 {
        tunnel: ["QnRtn=1" w953 "ExeRtn=1"] -> w936
        tunnel: w935 -> [_ w947 _]
        tunnel: w934 -> [_ w943 _]
        frame "返回请求应答", Default {
          n612 = global read "全局 数据数组大小.vi" "数据数组大小"() -> (w938:i32)
          n613 = Equal To 0?(x=w938) -> (x = 0?=w939:bool)
          n614 = case shown="True" w939 {
            frame False {
            }
            frame True {
              n615 = global read "全局 小时数据发送次数.vi" "小时数据发送次数"() -> (w942:i32)
              n616 = Increment(x=w942) -> (x+1=w941:i32)
              n617 = global write "全局 小时数据发送次数.vi" "小时数据发送次数"(w941) -> ()
            }
          }
        }
        frame "上传数据" {
          # "CODMn"
          n618 = global read "全局 小时数据发送次数.vi" "小时数据发送次数"() -> (w946:i32)
          n619 = call "数据发送组合-20200825 (子VI).vi"("枚举"=T4."平行样测试", "插值后的数组元素"=w943) -> ("字符串"=w944:string)  [unwired: 9 in]
          n620 = Index Array(array=w947, index (row)=w946) -> (element=w951:string[])  [unwired: 1 in]
          n621 = Index Array(array=w951, index=0 ("索引")) -> (element=w948:string)
          n622 = call "规范时间戳.vi"("字符串"=w948) -> ("result string"=w949:string)  [unwired: 10 in]
          n623 = Empty String/Path?(string/path=w948) -> (empty?=w952:bool)
          n624 = Format Into String(format string="DataTime=%s;%s" ("格式字符串"), w949, w944) -> (resulting string=w954:string)  [unwired: 2 in, 1 out]
          n625 = case shown="True" w952 {
            tunnel: [w958 ""] -> w953
            tunnel: w954 -> [w958 _]
            frame False {
              n626 = global read "全局 小时数据发送次数.vi" "小时数据发送次数"() -> (w957:i32)
              n627 = Increment(x=w957) -> (x+1=w956:i32)
              n628 = global write "全局 小时数据发送次数.vi" "小时数据发送次数"(w956) -> ()
            }
            frame True {
              n629 = global read "全局 小时数据发送次数.vi" "小时数据发送次数"() -> (w960:i32)
              n630 = Increment(x=w960) -> (x+1=w959:i32)
              n631 = global write "全局 小时数据发送次数.vi" "小时数据发送次数"(w959) -> ()
            }
          }
        }
        frame "返回执行结果" {
        }
      }
    }
    frame "提取集成干预" {
      # "提取平行样数据"
      n632 = global read "全局1.vi" "枚举"() -> (w963:enum16{"返回请求应答", "上传数据", "返回执行结果"})
      n633 = case shown="\"上传数据\"" w963 {
        tunnel: ["QnRtn=1" w983 "ExeRtn=1"] -> w966
        tunnel: w965 -> [_ w978 _]
        tunnel: w964 -> [_ w975 _]
        frame "返回请求应答", Default {
          n634 = global read "全局 数据数组大小.vi" "数据数组大小"() -> (w967:i32)
          n635 = Equal To 0?(x=w967) -> (x = 0?=w968:bool)
          n636 = case shown="True" w968 {
            frame False {
            }
            frame True {
              n637 = global read "全局 小时数据发送次数.vi" "小时数据发送次数"() -> (w971:i32)
              n638 = Increment(x=w971) -> (x+1=w970:i32)
              n639 = global write "全局 小时数据发送次数.vi" "小时数据发送次数"(w970) -> ()
            }
          }
        }
        frame "上传数据" {
          # "CODMn"
          n640 = global read "全局 小时数据发送次数.vi" "小时数据发送次数"() -> (w979:i32)
          n641 = call "数据发送组合-20200825 (子VI).vi"("枚举"=T4."集成干预测试", "插值后的数组元素"=w975) -> ("字符串"=w976:string)  [unwired: 9 in]
          n642 = Index Array(array=w978, index (row)=w979) -> (element=w981:string[])  [unwired: 1 in]
          n643 = global read "断电保存全局.vi" "应用环境"() -> (w974:T8)
          n644 = Index Array(array=w981, index=0 ("索引")) -> (element=w973:string)
          n645 = case shown="\"GB212\", Default" w974 {
            tunnel: [w987 w988] -> w972
            tunnel: w973 -> [w986 w989]
            frame "STD" {
              n646 = call "规范时间戳.vi"("字符串"=w986) -> ("result string"=w987:string)  [unwired: 10 in]
            }
            frame "GB212", Default {
              n647 = call "规范分钟数据时间戳.vi"("字符串"=w989) -> ("result string"=w988:string)  [unwired: 10 in]
            }
          }
          n648 = Empty String/Path?(string/path=w973) -> (empty?=w982:bool)
          n649 = Format Into String(format string="DataTime=%s;%s" ("格式字符串"), w972, w976) -> (resulting string=w984:string)  [unwired: 2 in, 1 out]
          n650 = case shown="True" w982 {
            tunnel: [w992 ""] -> w983
            tunnel: w984 -> [w992 _]
            frame False {
              n651 = global read "全局 小时数据发送次数.vi" "小时数据发送次数"() -> (w991:i32)
              n652 = Increment(x=w991) -> (x+1=w990:i32)
              n653 = global write "全局 小时数据发送次数.vi" "小时数据发送次数"(w990) -> ()
            }
            frame True {
              n654 = global read "全局 小时数据发送次数.vi" "小时数据发送次数"() -> (w994:i32)
              n655 = Increment(x=w994) -> (x+1=w993:i32)
              n656 = global write "全局 小时数据发送次数.vi" "小时数据发送次数"(w993) -> ()
            }
          }
        }
        frame "返回执行结果" {
        }
      }
    }
    frame "操作日志" {
      n657 = global read "全局 小时数据发送次数.vi" "小时数据发送次数"() -> (w999:i32)
      n658 = Index Array(array=w1001, index (row)=w999) -> (element=w998:string[])  [unwired: 1 in]
      n659 = global read "全局1.vi" "枚举"() -> (w1000:enum16{"返回请求应答", "上传数据", "返回执行结果"})
      n660 = case shown="\"上传数据\"" w1000 {
        tunnel: ["QnRtn=1" w1019 "ExeRtn=1"] -> w1002
        tunnel: w998 -> [_ w1021 _]
        tunnel: w997 -> [_ w1009 _]
        frame "返回请求应答", Default {
          n661 = global read "全局 数据数组大小.vi" "数据数组大小"() -> (w1005:i32)
          n662 = Equal To 0?(x=w1005) -> (x = 0?=w1004:bool)
          n663 = case shown="True" w1004 {
            frame False {
            }
            frame True {
              n664 = global read "全局 小时数据发送次数.vi" "小时数据发送次数"() -> (w1007:i32)
              n665 = Increment(x=w1007) -> (x+1=w1006:i32)
              n666 = global write "全局 小时数据发送次数.vi" "小时数据发送次数"(w1006) -> ()
            }
          }
        }
        frame "上传数据" {
          n667 = Index Array(array=w1021, index #1=0 ("索引"), index #2=2 ("索引")) -> (element #1=w1014:string)  [unwired: 1 out]
          n668 = call "规范时间戳.vi"("字符串"=w1014) -> ("result string"=w1012:string)  [unwired: 10 in]
          n669 = call "数据发送组合-20200825 (子VI).vi"("枚举"=T5."操作日志", "插值后的数组元素"=w1009) -> ("字符串"=w1008:string)  [unwired: 9 in]
          n670 = Format Into String(format string="DataTime=%s;", w1012) -> (resulting string=w1011:string)  [unwired: 2 in, 1 out]
          n671 = Concatenate Strings(w1011, w1008) -> (w1016:string)
          n672 = Empty String/Path?(string/path=w1016) -> (empty?=w1020:bool)
          n673 = String Length(string=w1016) -> (length=w1018:i32)
          n674 = Decrement(x=w1018) -> (x-1=w1017:i32)
          n675 = String Subset(string=w1016, length (rest)=w1017) -> (substring=w1015:string)  [unwired: 1 in]
          n676 = case shown="False" w1020 {
            tunnel: [w1026 ""] -> w1019
            tunnel: w1015 -> [w1026 _]
            frame False {
              n677 = global read "全局 小时数据发送次数.vi" "小时数据发送次数"() -> (w1025:i32)
              n678 = Increment(x=w1025) -> (x+1=w1024:i32)
              n679 = global write "全局 小时数据发送次数.vi" "小时数据发送次数"(w1024) -> ()
            }
            frame True {
              n680 = global read "全局 小时数据发送次数.vi" "小时数据发送次数"() -> (w1028:i32)
              n681 = Increment(x=w1028) -> (x+1=w1027:i32)
              n682 = global write "全局 小时数据发送次数.vi" "小时数据发送次数"(w1027) -> ()
            }
          }
        }
        frame "返回执行结果" {
        }
      }
    }
    frame "3092日志信息" {
      n683 = global read "全局 小时数据发送次数.vi" "小时数据发送次数"() -> (w1033:i32)
      n684 = global read "全局 所有参数.vi" "CODMn"() -> (w1031:string[][])
      n685 = Index Array(array=w1031, index (row)=w1033) -> (element=w1032:string[])  [unwired: 1 in]
      n686 = global read "全局1.vi" "枚举"() -> (w1034:enum16{"返回请求应答", "上传数据", "返回执行结果"})
      n687 = case shown="\"上传数据\"" w1034 {
        tunnel: ["QnRtn=1" w1053 "ExeRtn=1"] -> w1035
        tunnel: w1032 -> [_ w1055 _]
        frame "返回请求应答", Default {
          n688 = global read "全局 数据数组大小.vi" "数据数组大小"() -> (w1038:i32)
          n689 = Equal To 0?(x=w1038) -> (x = 0?=w1037:bool)
          n690 = case shown="True" w1037 {
            frame False {
            }
            frame True {
              n691 = global read "全局 小时数据发送次数.vi" "小时数据发送次数"() -> (w1040:i32)
              n692 = Increment(x=w1040) -> (x+1=w1039:i32)
              n693 = global write "全局 小时数据发送次数.vi" "小时数据发送次数"(w1039) -> ()
            }
          }
        }
        frame "上传数据" {
          n694 = Index Array(array=w1055, index #1=0 ("索引")) -> (element #1=w1048:string, element #2=w1041:string, element #3=w1043:string)  [unwired: 2 in]
          n695 = Empty String/Path?(string/path=w1041) -> (empty?=w1054:bool)
          n696 = call "规范时间戳.vi"("字符串"=w1048) -> ("result string"=w1045:string)  [unwired: 10 in]
          n697 = Format Into String(format string="DataTime=%s;", w1045) -> (resulting string=w1046:string)  [unwired: 2 in, 1 out]
          n698 = Format Into String(format string="parameter=//%s//,content==//%s//;" ("格式字符串"), w1041, w1043) -> (resulting string=w1042:string)  [unwired: 2 in, 1 out]
          n699 = Concatenate Strings(w1046, w1042) -> (w1050:string)
          n700 = String Length(string=w1050) -> (length=w1052:i32)
          n701 = Decrement(x=w1052) -> (x-1=w1051:i32)
          n702 = String Subset(string=w1050, length (rest)=w1051) -> (substring=w1049:string)  [unwired: 1 in]
          n703 = case shown="False" w1054 {
            tunnel: [w1059 ""] -> w1053
            tunnel: w1049 -> [w1059 _]
            frame False {
              n704 = global read "全局 小时数据发送次数.vi" "小时数据发送次数"() -> (w1058:i32)
              n705 = Increment(x=w1058) -> (x+1=w1057:i32)
              n706 = global write "全局 小时数据发送次数.vi" "小时数据发送次数"(w1057) -> ()
            }
            frame True {
              n707 = global read "全局 小时数据发送次数.vi" "小时数据发送次数"() -> (w1061:i32)
              n708 = Increment(x=w1061) -> (x+1=w1060:i32)
              n709 = global write "全局 小时数据发送次数.vi" "小时数据发送次数"(w1060) -> ()
            }
          }
        }
        frame "返回执行结果" {
        }
      }
    }
    frame "3093报警信息" {
      n710 = global read "全局 小时数据发送次数.vi" "小时数据发送次数"() -> (w1066:i32)
      n711 = global read "全局 所有参数.vi" "CODMn"() -> (w1064:string[][])
      n712 = Index Array(array=w1064, index (row)=w1066) -> (element=w1065:string[])  [unwired: 1 in]
      n713 = global read "全局1.vi" "枚举"() -> (w1067:enum16{"返回请求应答", "上传数据", "返回执行结果"})
      n714 = case shown="\"上传数据\"" w1067 {
        tunnel: ["QnRtn=1" w1089 "ExeRtn=1"] -> w1068
        tunnel: w1065 -> [_ w1091 _]
        frame "返回请求应答", Default {
          n715 = global read "全局 数据数组大小.vi" "数据数组大小"() -> (w1071:i32)
          n716 = Equal To 0?(x=w1071) -> (x = 0?=w1070:bool)
          n717 = case shown="True" w1070 {
            frame False {
            }
            frame True {
              n718 = global read "全局 小时数据发送次数.vi" "小时数据发送次数"() -> (w1073:i32)
              n719 = Increment(x=w1073) -> (x+1=w1072:i32)
              n720 = global write "全局 小时数据发送次数.vi" "小时数据发送次数"(w1072) -> ()
            }
          }
        }
        frame "上传数据" {
          n721 = Index Array(array=w1091, index #1=0 ("索引")) -> (element #1=w1084:string, element #2=w1078:string, element #3=w1077:string, element #5=w1076:string, element #6=w1075:string)  [unwired: 5 in, 1 out]
          n722 = case shown="\"消除\", Default" w1075 {
            tunnel: ["0" "1"] -> w1074
            frame "消除", Default {
            }
            frame "产生" {
            }
          }
          n723 = Empty String/Path?(string/path=w1078) -> (empty?=w1090:bool)
          n724 = call "规范时间戳.vi"("字符串"=w1084) -> ("result string"=w1081:string)  [unwired: 10 in]
          n725 = Format Into String(format string="DataTime=%s;", w1081) -> (resulting string=w1082:string)  [unwired: 2 in, 1 out]
          n726 = Format Into String(format string="parameter=//%s//,code=//%s//,content=//%s//,state=%s;" ("格式字符串"), w1078, w1076, w1077, w1074) -> (resulting string=w1079:string)  [unwired: 2 in, 1 out]
          n727 = Concatenate Strings(w1082, w1079) -> (w1086:string)
          n728 = String Length(string=w1086) -> (length=w1088:i32)
          n729 = Decrement(x=w1088) -> (x-1=w1087:i32)
          n730 = String Subset(string=w1086, length (rest)=w1087) -> (substring=w1085:string)  [unwired: 1 in]
          n731 = case shown="False" w1090 {
            tunnel: [w1097 ""] -> w1089
            tunnel: w1085 -> [w1097 _]
            frame False {
              n732 = global read "全局 小时数据发送次数.vi" "小时数据发送次数"() -> (w1096:i32)
              n733 = Increment(x=w1096) -> (x+1=w1095:i32)
              n734 = global write "全局 小时数据发送次数.vi" "小时数据发送次数"(w1095) -> ()
            }
            frame True {
              n735 = global read "全局 小时数据发送次数.vi" "小时数据发送次数"() -> (w1099:i32)
              n736 = Increment(x=w1099) -> (x+1=w1098:i32)
              n737 = global write "全局 小时数据发送次数.vi" "小时数据发送次数"(w1098) -> ()
            }
          }
        }
        frame "返回执行结果" {
        }
      }
    }
    frame "仪器参数" {
      n738 = case shown="\"悬浮物\"" w1105 {
        selector: w1105 -> [w1109 _ _ _ _ _ _ _ _ _ _ _ _ _ _ _ _ _ _ _ _ _ _ _ _ _ _ _ _ _ _ _ _]
        tunnel: [w1109 w1112 w1116 w1120 w1124 w1128 w1132 w1136 w1140 w1144 w1148 w1152 w1156 w1160 w1164 w1168 w1172 w1176 w1180 w1184 w1188 w1192 w1196 w1200 w1204 w1208 w1212 w1216 w1220 w1224 w1228 w1232 w1236] -> w1104
        tunnel: [1.0 ("风向") w1110 w1114 w1118 w1122 w1126 w1130 w1134 w1138 w1142 w1146 w1150 w1154 w1158 w1162 w1166 w1170 w1174 w1178 w1182 w1186 w1190 w1194 w1198 w1202 w1206 w1210 w1214 w1218 w1222 w1226 w1230 w1234] -> _
        frame "假", Default {
        }
        frame "CODMn" {
          n739 = global read "断电保存全局.vi" "参数系数簇"() -> (w1111:T9)
          n740 = global read "断电保存全局.vi" "因子编码簇"() -> (w1113:T10)
          n741 = Unbundle By Name(w1111) -> ("CODMn"=w1110:dbl)
          n742 = Unbundle By Name(w1113) -> ("CODMn"=w1112:string)
        }
        frame "CODCr" {
          n743 = global read "断电保存全局.vi" "参数系数簇"() -> (w1115:T9)
          n744 = global read "断电保存全局.vi" "因子编码簇"() -> (w1117:T10)
          n745 = Unbundle By Name(w1115) -> ("CODCr"=w1114:dbl)
          n746 = Unbundle By Name(w1117) -> ("CODCr"=w1116:string)
        }
        frame "DO" {
          n747 = global read "断电保存全局.vi" "参数系数簇"() -> (w1119:T9)
          n748 = global read "断电保存全局.vi" "因子编码簇"() -> (w1121:T10)
          n749 = Unbundle By Name(w1119) -> ("DO"=w1118:dbl)
          n750 = Unbundle By Name(w1121) -> ("DO"=w1120:string)
        }
        frame "铜" {
          n751 = global read "断电保存全局.vi" "参数系数簇"() -> (w1123:T9)
          n752 = global read "断电保存全局.vi" "因子编码簇"() -> (w1125:T10)
          n753 = Unbundle By Name(w1123) -> ("铜"=w1122:dbl)
          n754 = Unbundle By Name(w1125) -> ("铜"=w1124:string)
        }
        frame "PH" {
          n755 = global read "断电保存全局.vi" "参数系数簇"() -> (w1127:T9)
          n756 = global read "断电保存全局.vi" "因子编码簇"() -> (w1129:T10)
          n757 = Unbundle By Name(w1127) -> ("PH"=w1126:dbl)
          n758 = Unbundle By Name(w1129) -> ("PH"=w1128:string)
        }
        frame "氨氮" {
          n759 = global read "断电保存全局.vi" "参数系数簇"() -> (w1131:T9)
          n760 = global read "断电保存全局.vi" "因子编码簇"() -> (w1133:T10)
          n761 = Unbundle By Name(w1131) -> ("氨氮"=w1130:dbl)
          n762 = Unbundle By Name(w1133) -> ("氨氮"=w1132:string)
        }
        frame "比电导率" {
          n763 = global read "断电保存全局.vi" "参数系数簇"() -> (w1135:T9)
          n764 = global read "断电保存全局.vi" "因子编码簇"() -> (w1137:T10)
          n765 = Unbundle By Name(w1135) -> ("比电导率"=w1134:dbl)
          n766 = Unbundle By Name(w1137) -> ("比电导率"=w1136:string)
        }
        frame "水温" {
          n767 = global read "断电保存全局.vi" "参数系数簇"() -> (w1139:T9)
          n768 = global read "断电保存全局.vi" "因子编码簇"() -> (w1141:T10)
          n769 = Unbundle By Name(w1139) -> ("水温"=w1138:dbl)
          n770 = Unbundle By Name(w1141) -> ("水温"=w1140:string)
        }
        frame "COD" {
          n771 = global read "断电保存全局.vi" "参数系数簇"() -> (w1143:T9)
          n772 = global read "断电保存全局.vi" "因子编码簇"() -> (w1145:T10)
          n773 = Unbundle By Name(w1143) -> ("COD"=w1142:dbl)
          n774 = Unbundle By Name(w1145) -> ("COD"=w1144:string)
        }
        frame "浊度" {
          n775 = global read "断电保存全局.vi" "参数系数簇"() -> (w1147:T9)
          n776 = global read "断电保存全局.vi" "因子编码簇"() -> (w1149:T10)
          n777 = Unbundle By Name(w1147) -> ("浊度"=w1146:dbl)
          n778 = Unbundle By Name(w1149) -> ("浊度"=w1148:string)
        }
        frame "悬浮物" {
          n779 = global read "断电保存全局.vi" "参数系数簇"() -> (w1151:T9)
          n780 = global read "断电保存全局.vi" "因子编码簇"() -> (w1153:T10)
          n781 = Unbundle By Name(w1151) -> ("悬浮物"=w1150:dbl)
          n782 = Unbundle By Name(w1153) -> ("悬浮物"=w1152:string)
        }
        frame "总氮" {
          n783 = global read "断电保存全局.vi" "参数系数簇"() -> (w1155:T9)
          n784 = global read "断电保存全局.vi" "因子编码簇"() -> (w1157:T10)
          n785 = Unbundle By Name(w1155) -> ("总氮"=w1154:dbl)
          n786 = Unbundle By Name(w1157) -> ("总氮"=w1156:string)
        }
        frame "总磷" {
          n787 = global read "断电保存全局.vi" "参数系数簇"() -> (w1159:T9)
          n788 = global read "断电保存全局.vi" "因子编码簇"() -> (w1161:T10)
          n789 = Unbundle By Name(w1159) -> ("总磷"=w1158:dbl)
          n790 = Unbundle By Name(w1161) -> ("总磷"=w1160:string)
        }
        frame "叶绿素a" {
          n791 = global read "断电保存全局.vi" "参数系数簇"() -> (w1163:T9)
          n792 = global read "断电保存全局.vi" "因子编码簇"() -> (w1165:T10)
          n793 = Unbundle By Name(w1163) -> ("叶绿素a"=w1162:dbl)
          n794 = Unbundle By Name(w1165) -> ("叶绿素a"=w1164:string)
        }
        frame "藻密度" {
          n795 = global read "断电保存全局.vi" "参数系数簇"() -> (w1167:T9)
          n796 = global read "断电保存全局.vi" "因子编码簇"() -> (w1169:T10)
          n797 = Unbundle By Name(w1167) -> ("藻密度"=w1166:dbl)
          n798 = Unbundle By Name(w1169) -> ("藻密度"=w1168:string)
        }
        frame "水位" {
          n799 = global read "断电保存全局.vi" "参数系数簇"() -> (w1171:T9)
          n800 = global read "断电保存全局.vi" "因子编码簇"() -> (w1173:T10)
          n801 = Unbundle By Name(w1171) -> ("水位"=w1170:dbl)
          n802 = Unbundle By Name(w1173) -> ("水位"=w1172:string)
        }
        frame "流速" {
          n803 = global read "断电保存全局.vi" "参数系数簇"() -> (w1175:T9)
          n804 = global read "断电保存全局.vi" "因子编码簇"() -> (w1177:T10)
          n805 = Unbundle By Name(w1175) -> ("流速"=w1174:dbl)
          n806 = Unbundle By Name(w1177) -> ("流速"=w1176:string)
        }
        frame "瞬时流量" {
          n807 = global read "断电保存全局.vi" "参数系数簇"() -> (w1179:T9)
          n808 = global read "断电保存全局.vi" "因子编码簇"() -> (w1181:T10)
          n809 = Unbundle By Name(w1179) -> ("瞬时流量"=w1178:dbl)
          n810 = Unbundle By Name(w1181) -> ("瞬时流量"=w1180:string)
        }
        frame "累积流量" {
          n811 = global read "断电保存全局.vi" "参数系数簇"() -> (w1183:T9)
          n812 = global read "断电保存全局.vi" "因子编码簇"() -> (w1185:T10)
          n813 = Unbundle By Name(w1183) -> ("累积流量"=w1182:dbl)
          n814 = Unbundle By Name(w1185) -> ("累积流量"=w1184:string)
        }
        frame "亚硝酸盐" {
          n815 = global read "断电保存全局.vi" "参数系数簇"() -> (w1187:T9)
          n816 = global read "断电保存全局.vi" "因子编码簇"() -> (w1189:T10)
          n817 = Unbundle By Name(w1187) -> ("亚硝酸盐"=w1186:dbl)
          n818 = Unbundle By Name(w1189) -> ("亚硝酸盐"=w1188:string)
        }
        frame "硫化物" {
          n819 = global read "断电保存全局.vi" "参数系数簇"() -> (w1191:T9)
          n820 = global read "断电保存全局.vi" "因子编码簇"() -> (w1193:T10)
          n821 = Unbundle By Name(w1191) -> ("硫化物"=w1190:dbl)
          n822 = Unbundle By Name(w1193) -> ("硫化物"=w1192:string)
        }
        frame "ORP" {
          n823 = global read "断电保存全局.vi" "参数系数簇"() -> (w1195:T9)
          n824 = global read "断电保存全局.vi" "因子编码簇"() -> (w1197:T10)
          n825 = Unbundle By Name(w1195) -> ("ORP"=w1194:dbl)
          n826 = Unbundle By Name(w1197) -> ("ORP"=w1196:string)
        }
        frame "铅" {
          n827 = global read "断电保存全局.vi" "参数系数簇"() -> (w1199:T9)
          n828 = global read "断电保存全局.vi" "因子编码簇"() -> (w1201:T10)
          n829 = Unbundle By Name(w1199) -> ("铅"=w1198:dbl)
          n830 = Unbundle By Name(w1201) -> ("铅"=w1200:string)
        }
        frame "镉" {
          n831 = global read "断电保存全局.vi" "参数系数簇"() -> (w1203:T9)
          n832 = global read "断电保存全局.vi" "因子编码簇"() -> (w1205:T10)
          n833 = Unbundle By Name(w1203) -> ("镉"=w1202:dbl)
          n834 = Unbundle By Name(w1205) -> ("镉"=w1204:string)
        }
        frame "锌" {
          n835 = global read "断电保存全局.vi" "参数系数簇"() -> (w1207:T9)
          n836 = global read "断电保存全局.vi" "因子编码簇"() -> (w1209:T10)
          n837 = Unbundle By Name(w1207) -> ("锌"=w1206:dbl)
          n838 = Unbundle By Name(w1209) -> ("锌"=w1208:string)
        }
        frame "镍" {
          n839 = global read "断电保存全局.vi" "参数系数簇"() -> (w1211:T9)
          n840 = global read "断电保存全局.vi" "因子编码簇"() -> (w1213:T10)
          n841 = Unbundle By Name(w1211) -> ("镍"=w1210:dbl)
          n842 = Unbundle By Name(w1213) -> ("镍"=w1212:string)
        }
        frame "锰" {
          n843 = global read "断电保存全局.vi" "参数系数簇"() -> (w1215:T9)
          n844 = global read "断电保存全局.vi" "因子编码簇"() -> (w1217:T10)
          n845 = Unbundle By Name(w1215) -> ("锰"=w1214:dbl)
          n846 = Unbundle By Name(w1217) -> ("锰"=w1216:string)
        }
        frame "汞" {
          n847 = global read "断电保存全局.vi" "参数系数簇"() -> (w1219:T9)
          n848 = global read "断电保存全局.vi" "因子编码簇"() -> (w1221:T10)
          n849 = Unbundle By Name(w1219) -> ("汞"=w1218:dbl)
          n850 = Unbundle By Name(w1221) -> ("汞"=w1220:string)
        }
        frame "气温" {
          n851 = global read "断电保存全局.vi" "参数系数簇"() -> (w1223:T9)
          n852 = global read "断电保存全局.vi" "因子编码簇"() -> (w1225:T10)
          n853 = Unbundle By Name(w1223) -> ("气温"=w1222:dbl)
          n854 = Unbundle By Name(w1225) -> ("气温"=w1224:string)
        }
        frame "气压" {
          n855 = global read "断电保存全局.vi" "参数系数簇"() -> (w1227:T9)
          n856 = global read "断电保存全局.vi" "因子编码簇"() -> (w1229:T10)
          n857 = Unbundle By Name(w1227) -> ("气压"=w1226:dbl)
          n858 = Unbundle By Name(w1229) -> ("气压"=w1228:string)
        }
        frame "风速" {
          n859 = global read "断电保存全局.vi" "参数系数簇"() -> (w1231:T9)
          n860 = global read "断电保存全局.vi" "因子编码簇"() -> (w1233:T10)
          n861 = Unbundle By Name(w1231) -> ("风速"=w1230:dbl)
          n862 = Unbundle By Name(w1233) -> ("风速"=w1232:string)
        }
        frame "风向" {
          n863 = global read "断电保存全局.vi" "参数系数簇"() -> (w1235:T9)
          n864 = global read "断电保存全局.vi" "因子编码簇"() -> (w1237:T10)
          n865 = Unbundle By Name(w1235) -> ("风向"=w1234:dbl)
          n866 = Unbundle By Name(w1237) -> ("风向"=w1236:string)
        }
      }
      n867 = global read "全局1.vi" "枚举"() -> (w1106:enum16{"返回请求应答", "上传数据", "返回执行结果"})
      n868 = case shown="\"上传数据\"" w1106 {
        tunnel: ["QnRtn=1" w1255 "ExeRtn=1"] -> w1107
        tunnel: w1103 -> [_ w1247 _]
        tunnel: w1104 -> [_ w1246 _]
        tunnel: w1102 -> [_ w1244 _]
        frame "返回请求应答", Default {
          n869 = global read "全局 数据数组大小.vi" "数据数组大小"() -> (w1240:i32)
          n870 = Equal To 0?(x=w1240) -> (x = 0?=w1239:bool)
          n871 = case shown="True" w1239 {
            frame False {
            }
            frame True {
              n872 = global read "全局 小时数据发送次数.vi" "小时数据发送次数"() -> (w1242:i32)
              n873 = Increment(x=w1242) -> (x+1=w1241:i32)
              n874 = global write "全局 小时数据发送次数.vi" "小时数据发送次数"(w1241) -> ()
            }
          }
        }
        frame "上传数据" {
          n875 = Index Array(array=w1247) -> (element=w1248:string)  [unwired: 1 in]
          n876 = case shown="\"原始时间\"" w1244 {
            tunnel: [w1258 w1260] -> w1249
            tunnel: w1248 -> [w1257 w1259]
            frame "精确到小时", Default {
              n877 = call "规范小时时间戳.vi"("字符串"=w1257) -> ("result string"=w1258:string)  [unwired: 10 in]
            }
            frame "原始时间" {
              n878 = call "日期字符串格式至时间格式转换(子VI).vi"("data[0]"=w1259) -> ("time stamp"=w1262:timestamp)  [unwired: 10 in]
              n879 = Seconds To Date/Time(time stamp (now)=w1262) -> (date time rec=w1261:T11)  [unwired: 1 in]
              n880 = Date/Time To Seconds(2:w1261) -> (0:w1263:timestamp)  [unwired: 1 in]
              n881 = Format Date/Time String(time format string (%c)="%Y%m%d%H%M%S" ("时间格式字符串(%c)"), seconds (now)=w1263) -> (date/time string=w1260:string)  [unwired: 1 in]
            }
          }
          n882 = call "关键参数组合 (子VI).vi"("table"="仪器参数", "因子编码"=w1246, "data"=w1247) -> ("字符串"=w1243:string)  [unwired: 8 in]
          n883 = Empty String/Path?(string/path=w1243) -> (empty?=w1256:bool)
          n884 = Format Into String(format string="DataTime=%s;%s" ("格式字符串"), w1249, w1243) -> (resulting string=w1251:string)  [unwired: 2 in, 1 out]
          n885 = String Length(string=w1251) -> (length=w1252:i32)
          n886 = Decrement(x=w1252) -> (x-1=w1253:i32)
          n887 = String Subset(string=w1251, length (rest)=w1253) -> (substring=w1250:string)  [unwired: 1 in]
          n888 = case shown="False" w1256 {
            tunnel: [w1265 ""] -> w1255
            tunnel: w1250 -> [w1265 _]
            frame False {
            }
            frame True {
            }
          }
        }
        frame "返回执行结果" {
        }
      }
    }
    frame "采配水仪器参数" {
      n889 = global read "全局1.vi" "枚举"() -> (w1271:enum16{"返回请求应答", "上传数据", "返回执行结果"})
      n890 = case shown="\"上传数据\"" w1271 {
        tunnel: ["QnRtn=1" w1296 "ExeRtn=1"] -> w1272
        tunnel: w1270 -> [_ w1284 _]
        tunnel: "w00000" -> [_ w1285 _]
        tunnel: w1269 -> [_ w1288 _]
        frame "返回请求应答", Default {
          n891 = global read "全局 数据数组大小.vi" "数据数组大小"() -> (w1275:i32)
          n892 = Equal To 0?(x=w1275) -> (x = 0?=w1274:bool)
          n893 = case shown="True" w1274 {
            frame False {
            }
            frame True {
              n894 = global read "全局 小时数据发送次数.vi" "小时数据发送次数"() -> (w1277:i32)
              n895 = Increment(x=w1277) -> (x+1=w1276:i32)
              n896 = global write "全局 小时数据发送次数.vi" "小时数据发送次数"(w1276) -> ()
            }
          }
        }
        frame "上传数据" {
          n897 = Index Array(array=w1284) -> (element=w1289:string)  [unwired: 1 in]
          n898 = case shown="\"原始时间\"" w1288 {
            tunnel: [w1299 w1301] -> w1290
            tunnel: w1289 -> [w1298 w1300]
            frame "精确到小时", Default {
              n899 = call "规范小时时间戳.vi"("字符串"=w1298) -> ("result string"=w1299:string)  [unwired: 10 in]
            }
            frame "原始时间" {
              n900 = call "日期字符串格式至时间格式转换(子VI).vi"("data[0]"=w1300) -> ("time stamp"=w1303:timestamp)  [unwired: 10 in]
              n901 = Seconds To Date/Time(time stamp (now)=w1303) -> (date time rec=w1302:T11)  [unwired: 1 in]
              n902 = Date/Time To Seconds(2:w1302) -> (0:w1304:timestamp)  [unwired: 1 in]
              n903 = Format Date/Time String(time format string (%c)="%Y%m%d%H%M%S" ("时间格式字符串(%c)"), seconds (now)=w1304) -> (date/time string=w1301:string)  [unwired: 1 in]
            }
          }
          n904 = Index Array(array=w1284, index #1=2 ("索引"), index #2=3 ("索引"), index #3=4 ("索引")) -> (element #1=w1280:string, element #2=w1279:string, element #3=w1278:string)
          n905 = Format Into String(format string="PolId=%s,i13111-Info=%s,i13112-Info=%s,i13113-Info=%s;", w1285, w1280, w1279, w1278) -> (resulting string=w1286:string)  [unwired: 2 in, 1 out]
          n906 = Empty String/Path?(string/path=w1286) -> (empty?=w1297:bool)
          n907 = Format Into String(format string="DataTime=%s;%s" ("格式字符串"), w1290, w1286) -> (resulting string=w1292:string)  [unwired: 2 in, 1 out]
          n908 = String Length(string=w1292) -> (length=w1293:i32)
          n909 = Decrement(x=w1293) -> (x-1=w1294:i32)
          n910 = String Subset(string=w1292, length (rest)=w1294) -> (substring=w1291:string)  [unwired: 1 in]
          n911 = case shown="False" w1297 {
            tunnel: [w1306 ""] -> w1296
            tunnel: w1291 -> [w1306 _]
            frame False {
            }
            frame True {
            }
          }
        }
        frame "返回执行结果" {
        }
      }
    }
    frame "3091校准信息" {
      n912 = case shown="\"悬浮物\"" w1312 {
        selector: w1312 -> [w1316 _ _ _ _ _ _ _ _ _ _ _ _ _ _ _ _ _ _ _ _ _ _ _ _ _ _ _ _ _ _ _ _]
        tunnel: [w1316 w1319 w1323 w1327 w1331 w1335 w1339 w1343 w1347 w1351 w1355 w1359 w1363 w1367 w1371 w1375 w1379 w1383 w1387 w1391 w1395 w1399 w1403 w1407 w1411 w1415 w1419 w1423 w1427 w1431 w1435 w1439 w1443] -> w1311
        tunnel: [1.0 ("风向") w1317 w1321 w1325 w1329 w1333 w1337 w1341 w1345 w1349 w1353 w1357 w1361 w1365 w1369 w1373 w1377 w1381 w1385 w1389 w1393 w1397 w1401 w1405 w1409 w1413 w1417 w1421 w1425 w1429 w1433 w1437 w1441] -> _
        frame "假", Default {
        }
        frame "CODMn" {
          n913 = global read "断电保存全局.vi" "参数系数簇"() -> (w1318:T9)
          n914 = global read "断电保存全局.vi" "因子编码簇"() -> (w1320:T10)
          n915 = Unbundle By Name(w1318) -> ("CODMn"=w1317:dbl)
          n916 = Unbundle By Name(w1320) -> ("CODMn"=w1319:string)
        }
        frame "CODCr" {
          n917 = global read "断电保存全局.vi" "参数系数簇"() -> (w1322:T9)
          n918 = global read "断电保存全局.vi" "因子编码簇"() -> (w1324:T10)
          n919 = Unbundle By Name(w1322) -> ("CODCr"=w1321:dbl)
          n920 = Unbundle By Name(w1324) -> ("CODCr"=w1323:string)
        }
        frame "DO" {
          n921 = global read "断电保存全局.vi" "参数系数簇"() -> (w1326:T9)
          n922 = global read "断电保存全局.vi" "因子编码簇"() -> (w1328:T10)
          n923 = Unbundle By Name(w1326) -> ("DO"=w1325:dbl)
          n924 = Unbundle By Name(w1328) -> ("DO"=w1327:string)
        }
        frame "铜" {
          n925 = global read "断电保存全局.vi" "参数系数簇"() -> (w1330:T9)
          n926 = global read "断电保存全局.vi" "因子编码簇"() -> (w1332:T10)
          n927 = Unbundle By Name(w1330) -> ("铜"=w1329:dbl)
          n928 = Unbundle By Name(w1332) -> ("铜"=w1331:string)
        }
        frame "PH" {
          n929 = global read "断电保存全局.vi" "参数系数簇"() -> (w1334:T9)
          n930 = global read "断电保存全局.vi" "因子编码簇"() -> (w1336:T10)
          n931 = Unbundle By Name(w1334) -> ("PH"=w1333:dbl)
          n932 = Unbundle By Name(w1336) -> ("PH"=w1335:string)
        }
        frame "氨氮" {
          n933 = global read "断电保存全局.vi" "参数系数簇"() -> (w1338:T9)
          n934 = global read "断电保存全局.vi" "因子编码簇"() -> (w1340:T10)
          n935 = Unbundle By Name(w1338) -> ("氨氮"=w1337:dbl)
          n936 = Unbundle By Name(w1340) -> ("氨氮"=w1339:string)
        }
        frame "比电导率" {
          n937 = global read "断电保存全局.vi" "参数系数簇"() -> (w1342:T9)
          n938 = global read "断电保存全局.vi" "因子编码簇"() -> (w1344:T10)
          n939 = Unbundle By Name(w1342) -> ("比电导率"=w1341:dbl)
          n940 = Unbundle By Name(w1344) -> ("比电导率"=w1343:string)
        }
        frame "水温" {
          n941 = global read "断电保存全局.vi" "参数系数簇"() -> (w1346:T9)
          n942 = global read "断电保存全局.vi" "因子编码簇"() -> (w1348:T10)
          n943 = Unbundle By Name(w1346) -> ("水温"=w1345:dbl)
          n944 = Unbundle By Name(w1348) -> ("水温"=w1347:string)
        }
        frame "COD" {
          n945 = global read "断电保存全局.vi" "参数系数簇"() -> (w1350:T9)
          n946 = global read "断电保存全局.vi" "因子编码簇"() -> (w1352:T10)
          n947 = Unbundle By Name(w1350) -> ("COD"=w1349:dbl)
          n948 = Unbundle By Name(w1352) -> ("COD"=w1351:string)
        }
        frame "浊度" {
          n949 = global read "断电保存全局.vi" "参数系数簇"() -> (w1354:T9)
          n950 = global read "断电保存全局.vi" "因子编码簇"() -> (w1356:T10)
          n951 = Unbundle By Name(w1354) -> ("浊度"=w1353:dbl)
          n952 = Unbundle By Name(w1356) -> ("浊度"=w1355:string)
        }
        frame "悬浮物" {
          n953 = global read "断电保存全局.vi" "参数系数簇"() -> (w1358:T9)
          n954 = global read "断电保存全局.vi" "因子编码簇"() -> (w1360:T10)
          n955 = Unbundle By Name(w1358) -> ("悬浮物"=w1357:dbl)
          n956 = Unbundle By Name(w1360) -> ("悬浮物"=w1359:string)
        }
        frame "总氮" {
          n957 = global read "断电保存全局.vi" "参数系数簇"() -> (w1362:T9)
          n958 = global read "断电保存全局.vi" "因子编码簇"() -> (w1364:T10)
          n959 = Unbundle By Name(w1362) -> ("总氮"=w1361:dbl)
          n960 = Unbundle By Name(w1364) -> ("总氮"=w1363:string)
        }
        frame "总磷" {
          n961 = global read "断电保存全局.vi" "参数系数簇"() -> (w1366:T9)
          n962 = global read "断电保存全局.vi" "因子编码簇"() -> (w1368:T10)
          n963 = Unbundle By Name(w1366) -> ("总磷"=w1365:dbl)
          n964 = Unbundle By Name(w1368) -> ("总磷"=w1367:string)
        }
        frame "叶绿素a" {
          n965 = global read "断电保存全局.vi" "参数系数簇"() -> (w1370:T9)
          n966 = global read "断电保存全局.vi" "因子编码簇"() -> (w1372:T10)
          n967 = Unbundle By Name(w1370) -> ("叶绿素a"=w1369:dbl)
          n968 = Unbundle By Name(w1372) -> ("叶绿素a"=w1371:string)
        }
        frame "藻密度" {
          n969 = global read "断电保存全局.vi" "参数系数簇"() -> (w1374:T9)
          n970 = global read "断电保存全局.vi" "因子编码簇"() -> (w1376:T10)
          n971 = Unbundle By Name(w1374) -> ("藻密度"=w1373:dbl)
          n972 = Unbundle By Name(w1376) -> ("藻密度"=w1375:string)
        }
        frame "水位" {
          n973 = global read "断电保存全局.vi" "参数系数簇"() -> (w1378:T9)
          n974 = global read "断电保存全局.vi" "因子编码簇"() -> (w1380:T10)
          n975 = Unbundle By Name(w1378) -> ("水位"=w1377:dbl)
          n976 = Unbundle By Name(w1380) -> ("水位"=w1379:string)
        }
        frame "流速" {
          n977 = global read "断电保存全局.vi" "参数系数簇"() -> (w1382:T9)
          n978 = global read "断电保存全局.vi" "因子编码簇"() -> (w1384:T10)
          n979 = Unbundle By Name(w1382) -> ("流速"=w1381:dbl)
          n980 = Unbundle By Name(w1384) -> ("流速"=w1383:string)
        }
        frame "瞬时流量" {
          n981 = global read "断电保存全局.vi" "参数系数簇"() -> (w1386:T9)
          n982 = global read "断电保存全局.vi" "因子编码簇"() -> (w1388:T10)
          n983 = Unbundle By Name(w1386) -> ("瞬时流量"=w1385:dbl)
          n984 = Unbundle By Name(w1388) -> ("瞬时流量"=w1387:string)
        }
        frame "累积流量" {
          n985 = global read "断电保存全局.vi" "参数系数簇"() -> (w1390:T9)
          n986 = global read "断电保存全局.vi" "因子编码簇"() -> (w1392:T10)
          n987 = Unbundle By Name(w1390) -> ("累积流量"=w1389:dbl)
          n988 = Unbundle By Name(w1392) -> ("累积流量"=w1391:string)
        }
        frame "亚硝酸盐" {
          n989 = global read "断电保存全局.vi" "参数系数簇"() -> (w1394:T9)
          n990 = global read "断电保存全局.vi" "因子编码簇"() -> (w1396:T10)
          n991 = Unbundle By Name(w1394) -> ("亚硝酸盐"=w1393:dbl)
          n992 = Unbundle By Name(w1396) -> ("亚硝酸盐"=w1395:string)
        }
        frame "硫化物" {
          n993 = global read "断电保存全局.vi" "参数系数簇"() -> (w1398:T9)
          n994 = global read "断电保存全局.vi" "因子编码簇"() -> (w1400:T10)
          n995 = Unbundle By Name(w1398) -> ("硫化物"=w1397:dbl)
          n996 = Unbundle By Name(w1400) -> ("硫化物"=w1399:string)
        }
        frame "ORP" {
          n997 = global read "断电保存全局.vi" "参数系数簇"() -> (w1402:T9)
          n998 = global read "断电保存全局.vi" "因子编码簇"() -> (w1404:T10)
          n999 = Unbundle By Name(w1402) -> ("ORP"=w1401:dbl)
          n1000 = Unbundle By Name(w1404) -> ("ORP"=w1403:string)
        }
        frame "铅" {
          n1001 = global read "断电保存全局.vi" "参数系数簇"() -> (w1406:T9)
          n1002 = global read "断电保存全局.vi" "因子编码簇"() -> (w1408:T10)
          n1003 = Unbundle By Name(w1406) -> ("铅"=w1405:dbl)
          n1004 = Unbundle By Name(w1408) -> ("铅"=w1407:string)
        }
        frame "镉" {
          n1005 = global read "断电保存全局.vi" "参数系数簇"() -> (w1410:T9)
          n1006 = global read "断电保存全局.vi" "因子编码簇"() -> (w1412:T10)
          n1007 = Unbundle By Name(w1410) -> ("镉"=w1409:dbl)
          n1008 = Unbundle By Name(w1412) -> ("镉"=w1411:string)
        }
        frame "锌" {
          n1009 = global read "断电保存全局.vi" "参数系数簇"() -> (w1414:T9)
          n1010 = global read "断电保存全局.vi" "因子编码簇"() -> (w1416:T10)
          n1011 = Unbundle By Name(w1414) -> ("锌"=w1413:dbl)
          n1012 = Unbundle By Name(w1416) -> ("锌"=w1415:string)
        }
        frame "镍" {
          n1013 = global read "断电保存全局.vi" "参数系数簇"() -> (w1418:T9)
          n1014 = global read "断电保存全局.vi" "因子编码簇"() -> (w1420:T10)
          n1015 = Unbundle By Name(w1418) -> ("镍"=w1417:dbl)
          n1016 = Unbundle By Name(w1420) -> ("镍"=w1419:string)
        }
        frame "锰" {
          n1017 = global read "断电保存全局.vi" "参数系数簇"() -> (w1422:T9)
          n1018 = global read "断电保存全局.vi" "因子编码簇"() -> (w1424:T10)
          n1019 = Unbundle By Name(w1422) -> ("锰"=w1421:dbl)
          n1020 = Unbundle By Name(w1424) -> ("锰"=w1423:string)
        }
        frame "汞" {
          n1021 = global read "断电保存全局.vi" "参数系数簇"() -> (w1426:T9)
          n1022 = global read "断电保存全局.vi" "因子编码簇"() -> (w1428:T10)
          n1023 = Unbundle By Name(w1426) -> ("汞"=w1425:dbl)
          n1024 = Unbundle By Name(w1428) -> ("汞"=w1427:string)
        }
        frame "气温" {
          n1025 = global read "断电保存全局.vi" "参数系数簇"() -> (w1430:T9)
          n1026 = global read "断电保存全局.vi" "因子编码簇"() -> (w1432:T10)
          n1027 = Unbundle By Name(w1430) -> ("气温"=w1429:dbl)
          n1028 = Unbundle By Name(w1432) -> ("气温"=w1431:string)
        }
        frame "气压" {
          n1029 = global read "断电保存全局.vi" "参数系数簇"() -> (w1434:T9)
          n1030 = global read "断电保存全局.vi" "因子编码簇"() -> (w1436:T10)
          n1031 = Unbundle By Name(w1434) -> ("气压"=w1433:dbl)
          n1032 = Unbundle By Name(w1436) -> ("气压"=w1435:string)
        }
        frame "风速" {
          n1033 = global read "断电保存全局.vi" "参数系数簇"() -> (w1438:T9)
          n1034 = global read "断电保存全局.vi" "因子编码簇"() -> (w1440:T10)
          n1035 = Unbundle By Name(w1438) -> ("风速"=w1437:dbl)
          n1036 = Unbundle By Name(w1440) -> ("风速"=w1439:string)
        }
        frame "风向" {
          n1037 = global read "断电保存全局.vi" "参数系数簇"() -> (w1442:T9)
          n1038 = global read "断电保存全局.vi" "因子编码簇"() -> (w1444:T10)
          n1039 = Unbundle By Name(w1442) -> ("风向"=w1441:dbl)
          n1040 = Unbundle By Name(w1444) -> ("风向"=w1443:string)
        }
      }
      n1041 = global read "全局1.vi" "枚举"() -> (w1313:enum16{"返回请求应答", "上传数据", "返回执行结果"})
      n1042 = case shown="\"上传数据\"" w1313 {
        tunnel: ["QnRtn=1" w1461 "ExeRtn=1"] -> w1314
        tunnel: w1310 -> [_ w1451 _]
        tunnel: w1311 -> [_ w1450 _]
        tunnel: w1309 -> [_ w1453 _]
        frame "返回请求应答", Default {
          n1043 = global read "全局 数据数组大小.vi" "数据数组大小"() -> (w1447:i32)
          n1044 = Equal To 0?(x=w1447) -> (x = 0?=w1446:bool)
          n1045 = case shown="True" w1446 {
            frame False {
            }
            frame True {
              n1046 = global read "全局 小时数据发送次数.vi" "小时数据发送次数"() -> (w1449:i32)
              n1047 = Increment(x=w1449) -> (x+1=w1448:i32)
              n1048 = global write "全局 小时数据发送次数.vi" "小时数据发送次数"(w1448) -> ()
            }
          }
        }
        frame "上传数据" {
          n1049 = call "校准信息组合 (子VI).vi"("因子编码"=w1450, "data"=w1451) -> ("字符串"=w1452:string)  [unwired: 9 in]
          n1050 = Index Array(array=w1451) -> (element=w1454:string)  [unwired: 1 in]
          n1051 = case shown="\"原始时间\"" w1453 {
            tunnel: [w1464 w1466] -> w1455
            tunnel: w1454 -> [w1463 w1465]
            frame "精确到小时", Default {
              n1052 = call "规范小时时间戳.vi"("字符串"=w1463) -> ("result string"=w1464:string)  [unwired: 10 in]
            }
            frame "原始时间" {
              n1053 = call "日期字符串格式至时间格式转换(子VI).vi"("data[0]"=w1465) -> ("time stamp"=w1468:timestamp)  [unwired: 10 in]
              n1054 = Seconds To Date/Time(time stamp (now)=w1468) -> (date time rec=w1467:T11)  [unwired: 1 in]
              n1055 = Date/Time To Seconds(2:w1467) -> (0:w1469:timestamp)  [unwired: 1 in]
              n1056 = Format Date/Time String(time format string (%c)="%Y%m%d%H%M%S" ("时间格式字符串(%c)"), seconds (now)=w1469) -> (date/time string=w1466:string)  [unwired: 1 in]
            }
          }
          n1057 = Empty String/Path?(string/path=w1452) -> (empty?=w1462:bool)
          n1058 = Format Into String(format string="DataTime=%s;%s" ("格式字符串"), w1455, w1452) -> (resulting string=w1457:string)  [unwired: 2 in, 1 out]
          n1059 = String Length(string=w1457) -> (length=w1458:i32)
          n1060 = Decrement(x=w1458) -> (x-1=w1459:i32)
          n1061 = String Subset(string=w1457, length (rest)=w1459) -> (substring=w1456:string)  [unwired: 1 in]
          n1062 = case shown="False" w1462 {
            tunnel: [w1471 ""] -> w1461
            tunnel: w1456 -> [w1471 _]
            frame False {
            }
            frame True {
            }
          }
        }
        frame "返回执行结果" {
        }
      }
    }
    frame "3090仪器参数" {
      n1063 = global read "全局 小时数据发送次数.vi" "小时数据发送次数"() -> (w1476:i32)
      n1064 = Index Array(array=w1478, index (row)=w1476) -> (element=w1475:string[])  [unwired: 1 in]
      n1065 = global read "全局1.vi" "枚举"() -> (w1477:enum16{"返回请求应答", "上传数据", "返回执行结果"})
      n1066 = case shown="\"上传数据\"" w1477 {
        tunnel: ["QnRtn=1" w1496 "ExeRtn=1"] -> w1479
        tunnel: w1475 -> [_ w1493 _]
        tunnel: w1474 -> [_ w1486 _]
        frame "返回请求应答", Default {
          n1067 = global read "全局 数据数组大小.vi" "数据数组大小"() -> (w1482:i32)
          n1068 = Equal To 0?(x=w1482) -> (x = 0?=w1481:bool)
          n1069 = case shown="True" w1481 {
            frame False {
            }
            frame True {
              n1070 = global read "全局 小时数据发送次数.vi" "小时数据发送次数"() -> (w1484:i32)
              n1071 = Increment(x=w1484) -> (x+1=w1483:i32)
              n1072 = global write "全局 小时数据发送次数.vi" "小时数据发送次数"(w1483) -> ()
            }
          }
        }
        frame "上传数据" {
          n1073 = Index Array(array=w1493) -> (element=w1492:string)  [unwired: 1 in]
          n1074 = call "数据发送组合-20200825 (子VI).vi"("枚举"=T6."3090仪器参数", "插值后的数组元素"=w1486) -> ("字符串"=w1485:string)  [unwired: 9 in]
          n1075 = call "规范时间戳.vi"("字符串"=w1492) -> ("result string"=w1494:string)  [unwired: 10 in]
          n1076 = Format Into String(format string="DataTime=%s;%s" ("格式字符串"), w1494, w1485) -> (resulting string=w1489:string)  [unwired: 2 in, 1 out]
          n1077 = String Length(string=w1489) -> (length=w1490:i32)
          n1078 = Decrement(x=w1490) -> (x-1=w1491:i32)
          n1079 = String Subset(string=w1489, length (rest)=w1491) -> (substring=w1488:string)  [unwired: 1 in]
          n1080 = Empty String/Path?(string/path=w1488) -> (empty?=w1497:bool)
          n1081 = case shown="False" w1497 {
            tunnel: [w1500 ""] -> w1496
            tunnel: w1488 -> [w1500 _]
            frame False {
              n1082 = global read "全局 小时数据发送次数.vi" "小时数据发送次数"() -> (w1499:i32)
              n1083 = Increment(x=w1499) -> (x+1=w1498:i32)
              n1084 = global write "全局 小时数据发送次数.vi" "小时数据发送次数"(w1498) -> ()
            }
            frame True {
              n1085 = global read "全局 小时数据发送次数.vi" "小时数据发送次数"() -> (w1502:i32)
              n1086 = Increment(x=w1502) -> (x+1=w1501:i32)
              n1087 = global write "全局 小时数据发送次数.vi" "小时数据发送次数"(w1501) -> ()
            }
          }
        }
        frame "返回执行结果" {
        }
      }
    }
    frame "提取仪器参数" {
      n1088 = global read "全局1.vi" "枚举"() -> (w1506:enum16{"返回请求应答", "上传数据", "返回执行结果"})
      n1089 = case shown="\"上传数据\"" w1506 {
        tunnel: ["QnRtn=1" w1516 "ExeRtn=1"] -> w1507
        tunnel: w1505 -> [_ w1514 _]
        frame "返回请求应答", Default {
          n1090 = global read "全局 数据数组大小.vi" "数据数组大小"() -> (w1510:i32)
          n1091 = Equal To 0?(x=w1510) -> (x = 0?=w1509:bool)
          n1092 = case shown="False" w1509 {
            frame False {
            }
            frame True {
              n1093 = global read "全局 小时数据发送次数.vi" "小时数据发送次数"() -> (w1512:i32)
              n1094 = Increment(x=w1512) -> (x+1=w1511:i32)
              n1095 = global write "全局 小时数据发送次数.vi" "小时数据发送次数"(w1511) -> ()
            }
          }
        }
        frame "上传数据" {
          n1096 = call "数据发送组合-20200825 (子VI).vi"("枚举"=T6."提取仪器参数", "插值后的数组元素"=w1514) -> ("字符串"=w1513:string)  [unwired: 9 in]
          n1097 = Empty String/Path?(string/path=w1513) -> (empty?=w1517:bool)
          n1098 = case shown="False" w1517 {
            tunnel: [w1520 ""] -> w1516
            tunnel: w1513 -> [w1520 _]
            frame False {
              n1099 = global read "全局 小时数据发送次数.vi" "小时数据发送次数"() -> (w1519:i32)
              n1100 = Increment(x=w1519) -> (x+1=w1518:i32)
              n1101 = global write "全局 小时数据发送次数.vi" "小时数据发送次数"(w1518) -> ()
            }
            frame True {
              n1102 = global read "全局 小时数据发送次数.vi" "小时数据发送次数"() -> (w1522:i32)
              n1103 = Increment(x=w1522) -> (x+1=w1521:i32)
              n1104 = global write "全局 小时数据发送次数.vi" "小时数据发送次数"(w1521) -> ()
            }
          }
        }
        frame "返回执行结果" {
        }
      }
    }
    frame "报警信息" {
      n1105 = global read "全局 小时数据发送次数.vi" "小时数据发送次数"() -> (w1527:i32)
      n1106 = Index Array(array=w1529, index (row)=w1527) -> (element=w1526:string[])  [unwired: 1 in]
      n1107 = global read "全局1.vi" "枚举"() -> (w1528:enum16{"返回请求应答", "上传数据", "返回执行结果"})
      n1108 = case shown="\"上传数据\"" w1528 {
        tunnel: ["QnRtn=1" w1542 "ExeRtn=1"] -> w1530
        tunnel: w1526 -> [_ _ _]
        tunnel: w1525 -> [_ w1537 _]
        frame "返回请求应答", Default {
          n1109 = global read "全局 数据数组大小.vi" "数据数组大小"() -> (w1533:i32)
          n1110 = Equal To 0?(x=w1533) -> (x = 0?=w1532:bool)
          n1111 = case shown="True" w1532 {
            frame False {
            }
            frame True {
              n1112 = global read "全局 小时数据发送次数.vi" "小时数据发送次数"() -> (w1535:i32)
              n1113 = Increment(x=w1535) -> (x+1=w1534:i32)
              n1114 = global write "全局 小时数据发送次数.vi" "小时数据发送次数"(w1534) -> ()
            }
          }
        }
        frame "上传数据" {
          n1115 = call "数据发送组合-20200825 (子VI).vi"("枚举"=T6."报警信息", "插值后的数组元素"=w1537) -> ("字符串"=w1536:string)  [unwired: 9 in]
          n1116 = Empty String/Path?(string/path=w1536) -> (empty?=w1543:bool)
          n1117 = String Length(string=w1536) -> (length=w1541:i32)
          n1118 = Decrement(x=w1541) -> (x-1=w1540:i32)
          n1119 = String Subset(string=w1536, length (rest)=w1540) -> (substring=w1539:string)  [unwired: 1 in]
          n1120 = case shown="False" w1543 {
            tunnel: [w1546 ""] -> w1542
            tunnel: w1539 -> [w1546 _]
            frame False {
              n1121 = global read "全局 小时数据发送次数.vi" "小时数据发送次数"() -> (w1545:i32)
              n1122 = Increment(x=w1545) -> (x+1=w1544:i32)
              n1123 = global write "全局 小时数据发送次数.vi" "小时数据发送次数"(w1544) -> ()
            }
            frame True {
              n1124 = global read "全局 小时数据发送次数.vi" "小时数据发送次数"() -> (w1548:i32)
              n1125 = Increment(x=w1548) -> (x+1=w1547:i32)
              n1126 = global write "全局 小时数据发送次数.vi" "小时数据发送次数"(w1547) -> ()
            }
          }
        }
        frame "返回执行结果" {
        }
      }
    }
    frame "系统状态" {
      # ",i12002-Info=0,i12003-Info=100,i12031-Info=0"
      # "DataTime=20100301145000;PolId=w01018,i12001-Info=1,i12003-Info=100"
      # "100  当前模式\n101  CODMn状态  （0待机，1运行）\n102  氨氮状态\n103  总磷状态\n104  总氮状态\n105  CODCr状态\n106  运行周期"
      n1127 = global read "全局 小时数据发送次数.vi" "小时数据发送次数"() -> (w1553:i32)
      n1128 = Build Array("w00000", "w01019", "w21003", "w21011", "w21001", "w01018") -> (w1561:string[])
      n1129 = global read "全局1.vi" "register values"() -> (w1559:u16[])
      n1130 = Index Array(array=w1559, index=w1553) -> (element=w1558:u16)
      n1131 = Index Array(array=w1561, index=w1553) -> (element=w1560:string)
      n1132 = global read "全局1.vi" "读取试剂余量的值"() -> (w1554:u16[])
      n1133 = Decrement(x=w1553) -> (x-1=w1552:i32)
      n1134 = Index Array(array=w1554, index=w1552) -> (element=w1551:u16)
      n1135 = case shown="1, Default" w1553 {
        tunnel: w1560 -> [w1577 w1581]
        tunnel: w1558 -> [w1578 _]
        tunnel: [w1576 w1580] -> w1557
        tunnel: w1551 -> [w1574 _]
        frame 1, Default {
          n1136 = Number To Decimal String(number=w1578) -> (decimal integer string=w1575:string)  [unwired: 1 in]
          n1137 = Format Into String(format string="PolId=%s,i12001-Info=%s,i12002-Info=0,i12003-Info=%d;" ("格式字符串"), w1577, w1575, w1574) -> (resulting string=w1576:string)  [unwired: 2 in, 1 out]
        }
        frame 0 {
          n1138 = Format Into String(format string="PolId=%s,i22001-Info=0,i22002-Info=1,i22003-Info=0;" ("格式字符串"), w1581) -> (resulting string=w1580:string)  [unwired: 2 in, 1 out]
        }
      }
      n1139 = Get Date/Time In Seconds() -> (seconds since 1Jan1904=w1571:timestamp)
      n1140 = Format Date/Time String(time format string (%c)="%Y%m%d%H%M%S" ("时间格式字符串(%c)"), seconds (now)=w1571) -> (date/time string=w1570:string)  [unwired: 1 in]
      n1141 = Format Into String(format string="DataTime=%s;%s" ("格式字符串"), w1570, w1557) -> (resulting string=w1567:string)  [unwired: 2 in, 1 out]
      n1142 = String Length(string=w1567) -> (length=w1569:i32)
      n1143 = Decrement(x=w1569) -> (x-1=w1568:i32)
      n1144 = String Subset(string=w1567, length (rest)=w1568) -> (substring=w1566:string)  [unwired: 1 in]
    }
    frame "运行模式" {
      # "DataTime=20100301145000;PolId=w01018,i12001-Info=1,i12003-Info=0"
      # "100  当前模式\n101  CODMn状态  （0待机，1运行）\n102  氨氮状态\n103  总磷状态\n104  总氮状态\n105  CODCr状态\n106  运行周期"
      n1145 = Get Date/Time In Seconds() -> (seconds since 1Jan1904=w1590:timestamp)
      n1146 = Format Date/Time String(time format string (%c)="%Y%m%d%H%M%S" ("时间格式字符串(%c)"), seconds (now)=w1590) -> (date/time string=w1587:string)  [unwired: 1 in]
      n1147 = global read "全局1.vi" "register values"() -> (w1592:u16[])
      n1148 = Index Array(array=w1592, index=0 ("索引")) -> (element=w1584:u16)
      n1149 = Number To Decimal String(number=w1584) -> (decimal integer string=w1586:string)  [unwired: 1 in]
      n1150 = Format Into String(format string="RunMode=%s;" ("格式字符串"), w1586) -> (resulting string=w1583:string)  [unwired: 2 in, 1 out]
      n1151 = Format Into String(format string="DataTime=%s;%s" ("格式字符串"), w1587, w1583) -> (resulting string=w1589:string)  [unwired: 2 in, 1 out]
    }
    frame "测量周期" {
      n1152 = global read "全局1.vi" "register values"() -> (w1603:u16[])
      n1153 = Index Array(array=w1603, index=6 ("索引")) -> (element=w1595:u16)
      n1154 = Get Date/Time In Seconds() -> (seconds since 1Jan1904=w1601:timestamp)
      n1155 = Format Date/Time String(time format string (%c)="%Y%m%d%H%M%S" ("时间格式字符串(%c)"), seconds (now)=w1601) -> (date/time string=w1598:string)  [unwired: 1 in]
      n1156 = Number To Decimal String(number=w1595) -> (decimal integer string=w1596:string)  [unwired: 1 in]
      n1157 = Format Into String(format string="RunInterval=%s;" ("格式字符串"), w1596) -> (resulting string=w1594:string)  [unwired: 2 in, 1 out]
      n1158 = Format Into String(format string="DataTime=%s;%s" ("格式字符串"), w1598, w1594) -> (resulting string=w1600:string)  [unwired: 2 in, 1 out]
    }
    frame "各参数测量周期" {
      # "QN=20101108135153914;ST=21;CN=2084;PW=123456;MN=A110000_0001;Flag=9;CP=&&DataTime=20100301145000;PolId=w01018,RunInterval=4;PolId=w01019,RunInterval=4;...&&"
      n1159 = global read "全局1.vi" "读取各参数测量周期的值"() -> (w1606:u16[])
      n1160 = Get Date/Time In Seconds() -> (seconds since 1Jan1904=w1609:timestamp)
      n1161 = call "2084上传各参数测量周期.vi"("读取各参数测量周期的值"=w1606) -> ("字符串"=w1605:string)  [unwired: 10 in]
      n1162 = Format Date/Time String(time format string (%c)="%Y%m%d%H%M%S" ("时间格式字符串(%c)"), seconds (now)=w1609) -> (date/time string=w1607:string)  [unwired: 1 in]
      n1163 = Format Into String(format string="DataTime=%s;%s" ("格式字符串"), w1607, w1605) -> (resulting string=w1608:string)  [unwired: 2 in, 1 out]
    }
    frame "超标留样" {
      # "DataTime=20100301145000;PolId=w01018,i12001-Info=1,i12003-Info=0"
      # "100  当前模式\n101  CODMn状态  （0待机，1运行）\n102  氨氮状态\n103  总磷状态\n104  总氮状态\n105  CODCr状态\n106  运行周期"
      n1164 = global read "全局1.vi" "register values"() -> (w1621:u16[])
      n1165 = Get Date/Time In Seconds() -> (seconds since 1Jan1904=w1619:timestamp)
      n1166 = Format Date/Time String(time format string (%c)="%Y%m%d%H%M%S" ("时间格式字符串(%c)"), seconds (now)=w1619) -> (date/time string=w1616:string)  [unwired: 1 in]
      n1167 = Index Array(array=w1621, index=7 ("索引")) -> (element=w1613:u16)
      n1168 = Number To Decimal String(number=w1613) -> (decimal integer string=w1614:string)  [unwired: 1 in]
      n1169 = Format Into String(format string="VaseNo=%s;" ("格式字符串"), w1614) -> (resulting string=w1612:string)  [unwired: 2 in, 1 out]
      n1170 = Format Into String(format string="DataTime=%s;%s" ("格式字符串"), w1616, w1612) -> (resulting string=w1618:string)  [unwired: 2 in, 1 out]
    }
    frame "3201告警信息" {
      n1171 = global read "全局 小时数据发送次数.vi" "告警码"() -> (w1623:i32)
      n1172 = Number To Decimal String(number=w1623) -> (decimal integer string=w1624:string)  [unwired: 1 in]
      n1173 = Get Date/Time In Seconds() -> (seconds since 1Jan1904=w1629:timestamp)
      n1174 = Format Date/Time String(time format string (%c)="%Y%m%d%H%M%S" ("时间格式字符串(%c)"), seconds (now)=w1629) -> (date/time string=w1627:string)  [unwired: 1 in]
      n1175 = Format Into String(format string="SystemAlarm=%s" ("格式字符串"), w1624) -> (resulting string=w1625:string)  [unwired: 2 in, 1 out]
      n1176 = Format Into String(format string="DataTime=%s;%s" ("格式字符串"), w1627, w1625) -> (resulting string=w1628:string)  [unwired: 2 in, 1 out]
    }
  }
  n1177 = case shown="False" w25 {
    tunnel: [w1633 w1637] -> w27
    frame False {
      n1178 = global read "全局1.vi" "枚举"() -> (w1632:enum16{"返回请求应答", "上传数据", "返回执行结果"})
      n1179 = case shown="\"上传数据\"" w1632 {
        tunnel: ["91" ("CN") w1635 "91" ("CN")] -> w1633
        frame "返回请求应答", Default {
        }
        frame "上传数据" {
          n1180 = global read "全局1.vi" "系统编码ST"() -> (w1635:string)
        }
        frame "返回执行结果" {
        }
      }
    }
    frame True {
      n1181 = global read "全局 反控命令枚举.vi" "反控命令枚举"() -> (w1638:enum16{"返回请求应答", "返回执行结果"})
      n1182 = case shown="\"返回执行结果\"" w1638 {
        tunnel: ["91" "91"] -> w1637
        frame "返回请求应答", Default {
        }
        frame "返回执行结果" {
        }
      }
    }
  }
  n1183 = case shown="\"提取平行样\"" "table输入" {
    tunnel: ["9015" ("ST") w1651 w1659 w1667 w1674 w1681 w1689 w1697 w1705 w1713 w1722 w1737 w1749 w1761 w1773 w1781 w1789 w1798 w1807 w1824 w1832 w1840 w1848 w1856 w1864 w1875 w1887 w1899 w1911 w1923 w1931 "3020" ("ST") "3042" ("ST") "3056" ("ST") "2084" ("ST") "3015" ("ST") "3201" ("ST")] -> w2
    tunnel: ["9" ("ST") "9" ("ST") "9" ("ST") "8" ("ST") "8" ("ST") "9" ("ST") "9" ("ST") "9" ("ST") "8" ("ST") "8" ("ST") "9" ("ST") "9" ("ST") "11" ("ST") "11" ("ST") "11" ("ST") "9" ("ST") "9" ("ST") w1801 "9" ("ST") "9" ("ST") "9" ("ST") "9" ("ST") "9" ("ST") "9" ("ST") "9" ("ST") "9" ("ST") "9" ("ST") "9" ("ST") "9" ("ST") "9" ("ST") "9" ("ST") "9" ("ST") "9" ("ST") "9" ("ST") "9" ("ST") "9" ("ST") "9" ("ST")] -> w29
    tunnel: w20 -> [_ w1649 w1657 w1668 w1675 w1682 w1690 w1698 w1706 w1714 w1723 w1739 w1751 w1763 w1775 w1783 w1791 w1800 w1810 w1826 w1834 w1842 w1850 w1858 w1866 w1877 w1889 w1901 w1913 w1925 w1933 w1939 w1943 w1947 w1951 w1955 w1959]
    tunnel: [_ w1649 w1657 w1668 w1675 w1682 w1690 w1698 w1706 w1714 w1723 w1739 w1751 w1763 w1775 w1783 w1791 w1800 w1810 w1826 w1834 w1842 w1850 w1858 w1866 w1877 w1889 w1901 w1913 w1925 w1933 w1939 w1943 w1947 w1951 w1955 w1959] -> w1
    tunnel: [w1641 w1648 w1656 w1664 w1672 w1679 w1687 w1695 w1703 w1711 w1719 w1736 w1748 w1760 w1772 w1780 w1788 w1797 w1809 w1822 w1830 w1838 w1846 w1854 w1862 w1870 w1882 w1894 w1906 w1918 w1930 w1938 w1942 w1946 w1950 w1954 w1958] -> w21
    tunnel: [_ _ _ _ _ _ _ _ _ _ _ _ w1746 w1758 w1770 _ _ _ _ _ _ _ _ _ _ _ _ _ _ _ _ _ _ _ _ _ _] -> w9
    tunnel: [_ _ _ _ _ _ _ _ _ _ _ _ w1744 w1756 w1768 _ _ _ _ _ _ _ _ _ _ _ _ _ _ _ _ _ _ _ _ _ _] -> w8
    frame "心跳包", Default {
      # "心跳包"
      n1184 = Get Date/Time In Seconds() -> (seconds since 1Jan1904=w1644:timestamp)
      n1185 = Format Date/Time String(time format string (%c)="%Y%m%d%H%M%S%3u" ("时间格式字符串(%c)"), seconds (now)=w1644) -> (date/time string=w1643:string)  [unwired: 1 in]
      n1186 = Search and Replace String(input string=w1643, search string="." ("搜索字符串")) -> (result string=w1641:string)  [unwired: 6 in, 3 out]
    }
    frame "提取数采仪时间" {
      n1187 = global read "全局1.vi" "枚举"() -> (w1652:enum16{"返回请求应答", "上传数据", "返回执行结果"})
      n1188 = case shown="\"上传数据\"" w1652 {
        tunnel: ["9011" ("CN") "1014" ("CN") "9012" ("CN")] -> w1651
        frame "返回请求应答", Default {
        }
        frame "上传数据" {
        }
        frame "返回执行结果" {
        }
      }
      n1189 = local read "QN"() -> (w1648:string)
    }
    frame "提取实时数据间隔" {
      n1190 = global read "全局1.vi" "枚举"() -> (w1660:enum16{"返回请求应答", "上传数据", "返回执行结果"})
      n1191 = case shown="\"上传数据\"" w1660 {
        tunnel: ["9011" ("CN") "1061" ("CN") "9012" ("CN")] -> w1659
        frame "返回请求应答", Default {
        }
        frame "上传数据" {
        }
        frame "返回执行结果" {
        }
      }
      n1192 = local read "QN"() -> (w1656:string)
    }
    frame "反控命令" {
      n1193 = global read "全局 反控命令枚举.vi" "反控命令枚举"() -> (w1665:enum16{"返回请求应答", "返回执行结果"})
      n1194 = case shown="\"返回执行结果\"" w1665 {
        tunnel: ["9011" ("CN") "9012" ("CN")] -> w1667
        frame "返回请求应答", Default {
        }
        frame "返回执行结果" {
        }
      }
      n1195 = local read "QN"() -> (w1664:string)
    }
    frame "超标留样返回" {
      n1196 = global read "全局1.vi" "枚举"() -> (w1671:enum16{"返回请求应答", "上传数据", "返回执行结果"})
      n1197 = case shown="\"上传数据\"" w1671 {
        tunnel: ["9011" ("CN") "3015" ("CN") "9012" ("CN")] -> w1674
        frame "返回请求应答", Default {
        }
        frame "上传数据" {
        }
        frame "返回执行结果" {
        }
      }
      n1198 = local read "QN"() -> (w1672:string)
    }
    frame "提取经纬度环境信息" {
      n1199 = global read "全局1.vi" "枚举"() -> (w1683:enum16{"返回请求应答", "上传数据", "返回执行结果"})
      n1200 = case shown="\"上传数据\"" w1683 {
        tunnel: ["9011" ("CN") "3041" ("CN") "9012" ("CN")] -> w1681
        frame "返回请求应答", Default {
        }
        frame "上传数据" {
        }
        frame "返回执行结果" {
        }
      }
      n1201 = local read "QN"() -> (w1679:string)
    }
    frame "提取现场系统信息" {
      n1202 = global read "全局1.vi" "枚举"() -> (w1691:enum16{"返回请求应答", "上传数据", "返回执行结果"})
      n1203 = case shown="\"上传数据\"" w1691 {
        tunnel: ["9011" ("CN") "3040" ("CN") "9012" ("CN")] -> w1689
        frame "返回请求应答", Default {
        }
        frame "上传数据" {
        }
        frame "返回执行结果" {
        }
      }
      n1204 = local read "QN"() -> (w1687:string)
    }
    frame "提取监测仪表时间" {
      n1205 = global read "全局1.vi" "枚举"() -> (w1699:enum16{"返回请求应答", "上传数据", "返回执行结果"})
      n1206 = case shown="\"上传数据\"" w1699 {
        tunnel: ["9011" ("CN") "1011" ("CN") "9012" ("CN")] -> w1697
        frame "返回请求应答", Default {
        }
        frame "上传数据" {
        }
        frame "返回执行结果" {
        }
      }
      n1207 = local read "QN"() -> (w1695:string)
    }
    frame "获取软件版本号" {
      n1208 = global read "全局1.vi" "枚举"() -> (w1707:enum16{"返回请求应答", "上传数据", "返回执行结果"})
      n1209 = case shown="\"返回执行结果\"" w1707 {
        tunnel: ["9011" ("CN") "3100" ("CN") "9012" ("CN")] -> w1705
        frame "返回请求应答", Default {
        }
        frame "上传数据" {
        }
        frame "返回执行结果" {
        }
      }
      n1210 = local read "QN"() -> (w1703:string)
    }
    frame "获取仪器软件版本号" {
      n1211 = global read "全局1.vi" "枚举"() -> (w1715:enum16{"返回请求应答", "上传数据", "返回执行结果"})
      n1212 = case shown="\"上传数据\"" w1715 {
        tunnel: ["9011" ("CN") "3102" ("CN") "9012" ("CN")] -> w1713
        frame "返回请求应答", Default {
        }
        frame "上传数据" {
        }
        frame "返回执行结果" {
        }
      }
      n1213 = local read "QN"() -> (w1711:string)
    }
    frame "实时数据" {
      n1214 = global read "全局1.vi" "枚举"() -> (w1721:enum16{"返回请求应答", "上传数据", "返回执行结果"})
      n1215 = case shown="\"上传数据\"" w1721 {
        tunnel: ["9011" ("CN") w1726 "9012" ("CN")] -> w1722
        frame "返回请求应答", Default {
        }
        frame "上传数据" {
          n1216 = global read "全局 实时数据参数.vi" "实时数据参数"() -> (w1725:string)
          n1217 = case shown="\"水样测试\", Default" w1725 {
            tunnel: ["2011" ("CN") "2064" ("CN") "2082" ("CN") "2063" ("CN") "2062" ("CN") "2065" ("CN") "2066" ("CN") "fff" ("CN")] -> w1726
            frame "水样测试", Default {
            }
            frame "平行样测试" {
            }
            frame "集成干预测试" {
            }
            frame "加标回收测试" {
            }
            frame "核查数据" {
            }
            frame "空白测试" {
            }
            frame "跨度核查" {
            }
            frame "" {
            }
          }
        }
        frame "返回执行结果" {
        }
      }
      n1218 = local read "QN"() -> (w1719:string)
    }
    frame "小时数据" {
      # "监测小时数据"
      n1219 = global read "全局1.vi" "枚举"() -> (w1738:enum16{"返回请求应答", "上传数据", "返回执行结果"})
      n1220 = case shown="\"上传数据\"" w1738 {
        tunnel: ["9011" ("CN") "2061" ("CN") "9012" ("CN")] -> w1737
        frame "返回请求应答", Default {
        }
        frame "上传数据" {
        }
        frame "返回执行结果" {
        }
      }
      n1221 = local read "QN"() -> (w1736:string)
    }
    frame "剖面数据" {
      n1222 = global read "全局1.vi" "枚举"() -> (w1750:enum16{"返回请求应答", "上传数据", "返回执行结果"})
      n1223 = case shown="\"上传数据\"" w1750 {
        tunnel: ["9011" ("CN") "2083" ("CN") "9012" ("CN")] -> w1749
        frame "返回请求应答", Default {
        }
        frame "上传数据" {
        }
        frame "返回执行结果" {
        }
      }
      n1224 = global read "全局 数据数组大小.vi" "当前包号"() -> (w1745:i32)
      n1225 = global read "全局 数据数组大小.vi" "总包数"() -> (w1747:i32)
      n1226 = Number To Decimal String(number=w1747) -> (decimal integer string=w1746:string)  [unwired: 1 in]
      n1227 = Number To Decimal String(number=w1745) -> (decimal integer string=w1744:string)  [unwired: 1 in]
      n1228 = local read "QN"() -> (w1748:string)
    }
    frame "海流计" {
      n1229 = global read "全局1.vi" "枚举"() -> (w1762:enum16{"返回请求应答", "上传数据", "返回执行结果"})
      n1230 = case shown="\"上传数据\"" w1762 {
        tunnel: ["9011" ("CN") "2083" ("CN") "9012" ("CN")] -> w1761
        frame "返回请求应答", Default {
        }
        frame "上传数据" {
        }
        frame "返回执行结果" {
        }
      }
      n1231 = global read "全局 数据数组大小.vi" "当前包号"() -> (w1757:i32)
      n1232 = global read "全局 数据数组大小.vi" "总包数"() -> (w1759:i32)
      n1233 = Number To Decimal String(number=w1759) -> (decimal integer string=w1758:string)  [unwired: 1 in]
      n1234 = Number To Decimal String(number=w1757) -> (decimal integer string=w1756:string)  [unwired: 1 in]
      n1235 = local read "QN"() -> (w1760:string)
    }
    frame "ADCP过程数据" {
      n1236 = global read "全局1.vi" "枚举"() -> (w1774:enum16{"返回请求应答", "上传数据", "返回执行结果"})
      n1237 = case shown="\"返回执行结果\"" w1774 {
        tunnel: ["9014" ("CN") "5001" ("CN") "9014" ("CN")] -> w1773
        frame "返回请求应答", Default {
        }
        frame "上传数据" {
        }
        frame "返回执行结果" {
        }
      }
      n1238 = global read "全局 数据数组大小.vi" "当前包号"() -> (w1769:i32)
      n1239 = global read "全局 数据数组大小.vi" "总包数"() -> (w1771:i32)
      n1240 = Number To Decimal String(number=w1771) -> (decimal integer string=w1770:string)  [unwired: 1 in]
      n1241 = Number To Decimal String(number=w1769) -> (decimal integer string=w1768:string)  [unwired: 1 in]
      n1242 = local read "QN"() -> (w1772:string)
    }
    frame "剖面多参数H" {
      # "监测小时数据"
      n1243 = global read "全局1.vi" "枚举"() -> (w1782:enum16{"返回请求应答", "上传数据", "返回执行结果"})
      n1244 = case shown="\"上传数据\"" w1782 {
        tunnel: ["9011" ("CN") "2061" ("CN") "9012" ("CN")] -> w1781
        frame "返回请求应答", Default {
        }
        frame "上传数据" {
        }
        frame "返回执行结果" {
        }
      }
      n1245 = local read "QN"() -> (w1780:string)
    }
    frame "剖面多参数S" {
      # "监测小时数据"
      n1246 = global read "全局1.vi" "枚举"() -> (w1790:enum16{"返回请求应答", "上传数据", "返回执行结果"})
      n1247 = case shown="\"上传数据\"" w1790 {
        tunnel: ["9011" ("CN") "2011" ("CN") "9012" ("CN")] -> w1789
        frame "返回请求应答", Default {
        }
        frame "上传数据" {
        }
        frame "返回执行结果" {
        }
      }
      n1248 = local read "QN"() -> (w1788:string)
    }
    frame "提取小时数据" {
      # "监测小时数据"
      n1249 = global read "全局1.vi" "枚举"() -> (w1799:enum16{"返回请求应答", "上传数据", "返回执行结果"})
      n1250 = global read "断电保存全局.vi" "数据组合发送"() -> (w1796:bool)
      n1251 = case shown="\"上传数据\"" w1799 {
        tunnel: ["9011" ("CN") "2061" ("CN") "9012" ("CN")] -> w1798
        frame "返回请求应答", Default {
        }
        frame "上传数据" {
        }
        frame "返回执行结果" {
        }
      }
      n1252 = case shown="False" w1796 {
        tunnel: ["9" ("ST") "9" ("ST")] -> w1801
        frame False {
        }
        frame True {
        }
      }
      n1253 = local read "QN"() -> (w1797:string)
    }
    frame "提取实时数据" {
      # "提取实时数据"
      n1254 = global read "全局1.vi" "枚举"() -> (w1808:enum16{"返回请求应答", "上传数据", "返回执行结果"})
      n1255 = case shown="\"上传数据\"" w1808 {
        tunnel: ["9011" ("CN") w1814 "9012" ("CN")] -> w1807
        frame "返回请求应答", Default {
        }
        frame "上传数据" {
          n1256 = global read "全局 实时数据参数.vi" "实时数据参数"() -> (w1813:string)
          n1257 = case shown="\"加标回收测试\"" w1813 {
            tunnel: ["2011" ("CN") "2064" ("CN") "2063" ("CN") "2065" ("CN") "2066" ("CN") "fff" ("CN")] -> w1814
            frame "水样测试", Default {
            }
            frame "平行样测试" {
            }
            frame "加标回收测试" {
            }
            frame "空白测试" {
            }
            frame "跨度核查" {
            }
            frame "" {
            }
          }
        }
        frame "返回执行结果" {
        }
      }
      n1258 = local read "QN"() -> (w1809:string)
    }
    frame "跨度核查" {
      # "跨度核查"
      n1259 = global read "全局1.vi" "枚举"() -> (w1825:enum16{"返回请求应答", "上传数据", "返回执行结果"})
      n1260 = case shown="\"返回执行结果\"" w1825 {
        tunnel: ["9011" ("CN") "2066" ("ST") "9012" ("CN")] -> w1824
        frame "返回请求应答", Default {
        }
        frame "上传数据" {
        }
        frame "返回执行结果" {
        }
      }
      n1261 = local read "QN"() -> (w1822:string)
    }
    frame "提取加标回收" {
      # "提取加标回收"
      n1262 = global read "全局1.vi" "枚举"() -> (w1833:enum16{"返回请求应答", "上传数据", "返回执行结果"})
      n1263 = case shown="\"上传数据\"" w1833 {
        tunnel: ["9011" ("CN") "2063" ("ST") "9012" ("CN")] -> w1832
        frame "返回请求应答", Default {
        }
        frame "上传数据" {
        }
        frame "返回执行结果" {
        }
      }
      n1264 = local read "QN"() -> (w1830:string)
    }
    frame "提取平行样" {
      # "提取平行样"
      n1265 = global read "全局1.vi" "枚举"() -> (w1841:enum16{"返回请求应答", "上传数据", "返回执行结果"})
      n1266 = case shown="\"上传数据\"" w1841 {
        tunnel: ["9011" ("CN") "2064" ("ST") "9012" ("CN")] -> w1840
        frame "返回请求应答", Default {
        }
        frame "上传数据" {
        }
        frame "返回执行结果" {
        }
      }
      n1267 = local read "QN"() -> (w1838:string)
    }
    frame "空白测试", "零点核查" {
      # "零点核查"
      n1268 = global read "全局1.vi" "枚举"() -> (w1849:enum16{"返回请求应答", "上传数据", "返回执行结果"})
      n1269 = case shown="\"上传数据\"" w1849 {
        tunnel: ["9011" ("CN") "2065" ("ST") "9012" ("CN")] -> w1848
        frame "返回请求应答", Default {
        }
        frame "上传数据" {
        }
        frame "返回执行结果" {
        }
      }
      n1270 = local read "QN"() -> (w1846:string)
    }
    frame "核查数据" {
      # "核查数据"
      n1271 = global read "全局1.vi" "枚举"() -> (w1857:enum16{"返回请求应答", "上传数据", "返回执行结果"})
      n1272 = case shown="\"上传数据\"" w1857 {
        tunnel: ["9011" ("CN") "2062" ("ST") "9012" ("CN")] -> w1856
        frame "返回请求应答", Default {
        }
        frame "上传数据" {
        }
        frame "返回执行结果" {
        }
      }
      n1273 = local read "QN"() -> (w1854:string)
    }
    frame "提取集成干预" {
      # "核查数据"
      n1274 = global read "全局1.vi" "枚举"() -> (w1865:enum16{"返回请求应答", "上传数据", "返回执行结果"})
      n1275 = case shown="\"上传数据\"" w1865 {
        tunnel: ["9011" ("CN") "2082" ("ST") "9012" ("CN")] -> w1864
        frame "返回请求应答", Default {
        }
        frame "上传数据" {
        }
        frame "返回执行结果" {
        }
      }
      n1276 = local read "QN"() -> (w1862:string)
    }
    frame "报警信息", "采配水仪器参数", "操作日志", "仪器参数" {
      n1277 = global read "全局1.vi" "枚举"() -> (w1876:enum16{"返回请求应答", "上传数据", "返回执行结果"})
      n1278 = case shown="\"上传数据\"" w1876 {
        tunnel: ["9011" ("CN") "3020" ("CN") "9012" ("CN")] -> w1875
        frame "返回请求应答", Default {
        }
        frame "上传数据" {
        }
        frame "返回执行结果" {
        }
      }
      n1279 = Get Date/Time In Seconds() -> (seconds since 1Jan1904=w1873:timestamp)
      n1280 = Format Date/Time String(time format string (%c)="%Y%m%d%H%M%S%3u" ("时间格式字符串(%c)"), seconds (now)=w1873) -> (date/time string=w1872:string)  [unwired: 1 in]
      n1281 = Search and Replace String(input string=w1872, search string="." ("搜索字符串")) -> (result string=w1870:string)  [unwired: 6 in, 3 out]
    }
    frame "3092日志信息" {
      n1282 = global read "全局1.vi" "枚举"() -> (w1888:enum16{"返回请求应答", "上传数据", "返回执行结果"})
      n1283 = case shown="\"上传数据\"" w1888 {
        tunnel: ["9011" ("CN") "3092" ("CN") "9012" ("CN")] -> w1887
        frame "返回请求应答", Default {
        }
        frame "上传数据" {
        }
        frame "返回执行结果" {
        }
      }
      n1284 = Get Date/Time In Seconds() -> (seconds since 1Jan1904=w1885:timestamp)
      n1285 = Format Date/Time String(time format string (%c)="%Y%m%d%H%M%S%3u" ("时间格式字符串(%c)"), seconds (now)=w1885) -> (date/time string=w1884:string)  [unwired: 1 in]
      n1286 = Search and Replace String(input string=w1884, search string="." ("搜索字符串")) -> (result string=w1882:string)  [unwired: 6 in, 3 out]
    }
    frame "3093报警信息" {
      n1287 = global read "全局1.vi" "枚举"() -> (w1900:enum16{"返回请求应答", "上传数据", "返回执行结果"})
      n1288 = case shown="\"上传数据\"" w1900 {
        tunnel: ["9011" ("CN") "3093" ("CN") "9012" ("CN")] -> w1899
        frame "返回请求应答", Default {
        }
        frame "上传数据" {
        }
        frame "返回执行结果" {
        }
      }
      n1289 = Get Date/Time In Seconds() -> (seconds since 1Jan1904=w1897:timestamp)
      n1290 = Format Date/Time String(time format string (%c)="%Y%m%d%H%M%S%3u" ("时间格式字符串(%c)"), seconds (now)=w1897) -> (date/time string=w1896:string)  [unwired: 1 in]
      n1291 = Search and Replace String(input string=w1896, search string="." ("搜索字符串")) -> (result string=w1894:string)  [unwired: 6 in, 3 out]
    }
    frame "3090仪器参数" {
      n1292 = global read "全局1.vi" "枚举"() -> (w1912:enum16{"返回请求应答", "上传数据", "返回执行结果"})
      n1293 = case shown="\"上传数据\"" w1912 {
        tunnel: ["9011" ("CN") "3090" ("CN") "9012" ("CN")] -> w1911
        frame "返回请求应答", Default {
        }
        frame "上传数据" {
        }
        frame "返回执行结果" {
        }
      }
      n1294 = Get Date/Time In Seconds() -> (seconds since 1Jan1904=w1909:timestamp)
      n1295 = Format Date/Time String(time format string (%c)="%Y%m%d%H%M%S%3u" ("时间格式字符串(%c)"), seconds (now)=w1909) -> (date/time string=w1908:string)  [unwired: 1 in]
      n1296 = Search and Replace String(input string=w1908, search string="." ("搜索字符串")) -> (result string=w1906:string)  [unwired: 6 in, 3 out]
    }
    frame "3091校准信息" {
      n1297 = global read "全局1.vi" "枚举"() -> (w1924:enum16{"返回请求应答", "上传数据", "返回执行结果"})
      n1298 = case shown="\"上传数据\"" w1924 {
        tunnel: ["9011" ("CN") "3091" ("CN") "9012" ("CN")] -> w1923
        frame "返回请求应答", Default {
        }
        frame "上传数据" {
        }
        frame "返回执行结果" {
        }
      }
      n1299 = Get Date/Time In Seconds() -> (seconds since 1Jan1904=w1921:timestamp)
      n1300 = Format Date/Time String(time format string (%c)="%Y%m%d%H%M%S%3u" ("时间格式字符串(%c)"), seconds (now)=w1921) -> (date/time string=w1920:string)  [unwired: 1 in]
      n1301 = Search and Replace String(input string=w1920, search string="." ("搜索字符串")) -> (result string=w1918:string)  [unwired: 6 in, 3 out]
    }
    frame "提取仪器参数" {
      n1302 = global read "全局1.vi" "枚举"() -> (w1932:enum16{"返回请求应答", "上传数据", "返回执行结果"})
      n1303 = case shown="\"上传数据\"" w1932 {
        tunnel: ["9011" ("CN") "3020" ("CN") "9012" ("CN")] -> w1931
        frame "返回请求应答", Default {
        }
        frame "上传数据" {
        }
        frame "返回执行结果" {
        }
      }
      n1304 = local read "QN"() -> (w1930:string)
    }
    frame "系统状态" {
      n1305 = local read "QN"() -> (w1938:string)
    }
    frame "运行模式" {
      n1306 = local read "QN"() -> (w1942:string)
    }
    frame "测量周期" {
      n1307 = local read "QN"() -> (w1946:string)
    }
    frame "各参数测量周期" {
      n1308 = local read "QN"() -> (w1950:string)
    }
    frame "超标留样" {
      n1309 = local read "QN"() -> (w1954:string)
    }
    frame "3201告警信息" {
      n1310 = local read "QN"() -> (w1958:string)
    }
  }
  n1311 = Bundle By Name(cluster="数据块", "ST"=w27, "CN"=w2, "FLAG"=w29, "CP"=w1, "QN"=w21, "MN"="MN", "PW"="PW", "PNUM"=w9, "PNO"=w8) -> (w28:T1)
  n1312 = call "HJ212-2017.vi"("PWD？"=FALSE, "数据段"=w28) -> ("通讯包字符串"=w4:string, "通讯包"=→"通讯包":T2)  [unwired: 7 in, 1 out]
  "通讯包字符串" <- w4
  n1313 = String Length(string=w4) -> (length=→"长度":i32)
  "错误常量" <- "错误常量 2"
  "小时数据发送次数" <- 0 ("小时数据发送次数")
  "核查数据发送次数" <- 0 ("核查数据发送次数")
